vi "Beta.vi"() -> ()   [LabVIEW 2019]
uses:
  Classes/Settings/ObjectSettings/ObjectSettings.lvclass/ObjectSettings.ctl
  <vilib>/Utility/miscctls.llb/LVPositionTypeDef.ctl
  Classes/Parse/ParseVectorFile/ParseVectorFile.lvclass
  C:/Program Files (x86)/National Instruments/LabVIEW 2019/vi.lib/JKI/JKI SMO/SMO/SMO.lvclass
  Classes/Settings/Setting Database/Setting Database.lvclass
  Classes/Tool/Tool Data/Tool Data/Tool Data.lvclass
  Classes/Subpanel/Manager/Subpanel.Edit.lvclass
  C:/Users/Albro/Documents/GitHub/AFM-Lithography/lvsrc/Classes/Subpanel/Subpanel.lvclass
  Classes/Render/BigMAQ/BigMAQ.lvclass
  Classes/Selector/Selector.lvclass
  subVIs/AFM API/AFM_Driver_Manager/AFM_Driver_Manager.lvclass
  <userlib>/LevyLab/Configuration/Configuration.lvclass
  Classes/Settings/Setting Database/Typedefs/PublicEvents--Setting Database.RectanglesUpdated.ctl
  Classes/Settings/Rectangle Settings/Rectangle Settings.lvclass
  C:/Users/Albro/Documents/GitHub/AFM-Lithography/lvsrc/Classes/Settings/ObjectSettings/ObjectSettings.lvclass
  Classes/Settings/Setting Database/Typedefs/PublicEvents--Setting Database.PathsUpdated.ctl
  Classes/Settings/Path Settings/Path Settings.lvclass
  Classes/Settings/Setting Database/Typedefs/PublicEvents--Setting Database.FunnelsUpdated.ctl
  Classes/Settings/Funnel Settings/Funnel Settings.lvclass
  Classes/Settings/Setting Database/Typedefs/PublicEvents--Setting Database.DotsUpdated.ctl
  Classes/Settings/Dot Settings/Dot Settings.lvclass
  Classes/Parse/ParsePaths/Path.lvclass
  Classes/Parse/Rectangle/Rectangle.lvclass
  Classes/Parse/Image/SVGImage.lvclass
  Classes/Parse/Dot/Dot.lvclass
  <userlib>/LevyLab/Relay Box/Typedefs/Resistor--enum.ctl
  Classes/Render/Inset/Inset.lvclass
  Classes/Log/Log.Litho/Log.Litho.lvclass
  Classes/Settings/Setting Database/Typedefs/PrivateEvents--Setting Database.Add To Group.ctl
  Classes/Settings/Setting Database/Typedefs/PrivateEvents--Setting Database.Create New Group.ctl
  Classes/Settings/Setting Database/Typedefs/PrivateEvents--Setting Database.Refresh.ctl
  Classes/Tool/Tool Data/Tool Data/Typedefs/PrivateEvents--Tool Data.Update Objects.ctl
  Classes/Parse/Image/SVGImage.lvclass/SVGImage.ctl
  Controls/Configuration.ctl
  a998b7c0-e198-41fb-897a-9ce541eca358.vi
  <vilib>/Platform/browser.llb/Open URL in Default Browser (string).vi
  <vilib>/Utility/sysdir.llb/Get System Directory.vi
  Classes/Tool/Tool Path/Tool Path.lvclass
  Classes/Tool/Tool Funnel/Tool Funnel.lvclass
  Classes/Tool/Tool Rectangle/Tool Rectangle.lvclass
  Classes/Tool/Tool Dot/Tool Dots.lvclass
  <userlib>/LevyLab/Relay Box/Relay-Box.lvclass
  Classes/Subpanel/Subpanel.lvclass
  <vilib>/JKI/JKI SMO/SMO/SMO.lvclass
  Classes/Settings/ObjectSettings/ObjectSettings.lvclass
  Classes/Identity/Identifier.lvclass
panel:
  out "Zoom":string
  in  "Zoom Type":enum32{"Zoom In", "Zoom Out"}(radio)
  in  "Zoom to Fit":bool
  out "Render":T1(plugin-control)
  out "version":string
  out "Ready?":bool
  out "Estimated Time":string
  in  "Run":bool
  in  "Refresh Button":bool
  in  "Done":bool
  in  "Help":bool
  in  "Abort":bool
  in  "Settings":T2(tab)
  out "Status":string
  in  "Background Image":path caption="Path"
  in  "Inkscape File (.svg)":path caption="Path"
  in  "Hide Labels?":bool
  in  "MCLB":i32(listbox) caption="Multicolumn Listbox 2"
  in  "AFM Type":u16(ring) caption="Ring" items=["Asylum"]
  in  "Overwrite?":bool
  in  "Normal Save Path":path caption="Path"
  in  "Save Render":bool caption="Save"
  in  "Autosave?":bool
  in  "Autosave Path":path caption="Path"
  in  "Inset Editor":bool
  out "Image Filename":string
  in  "Image Data Range":cluster{sgl, sgl}(slide)={100.0, 0.0} scale=0.0..100.0
  in  "Page":u32 caption="Numeric" max=3
  # "AFM Lithography"
  # "Render"
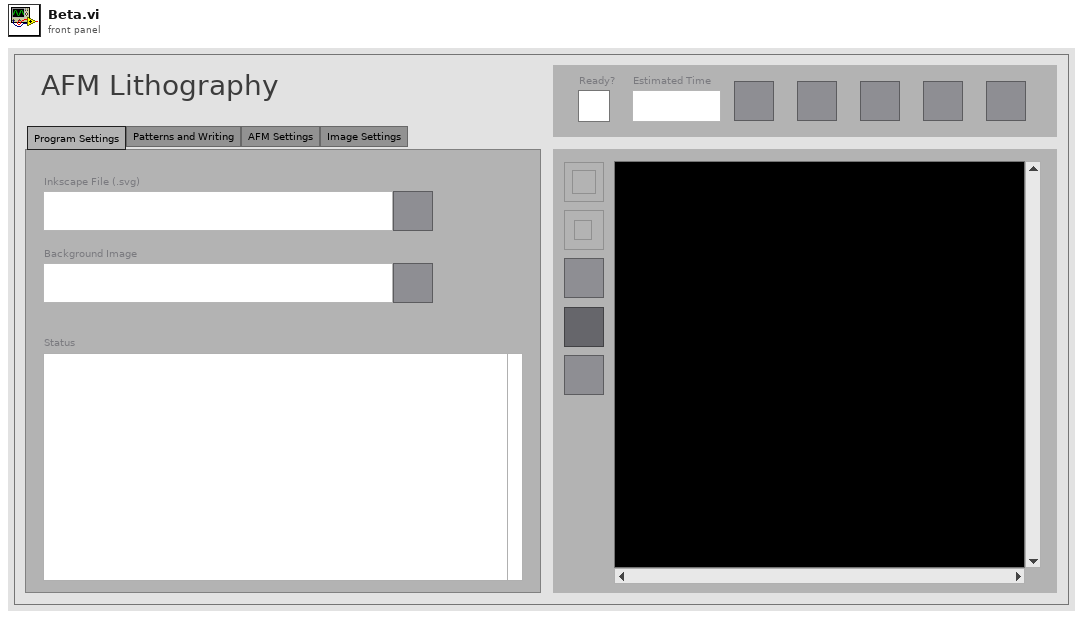
[diagram p1: front panel]
types:
  T1 = typedef "IMAQ Image.ctl" = refnum<image>
  T2 = enum32{"Program Settings", "Patterns and Writing", "AFM Settings", "Image Settings"}
  T3 = cluster{"Groups":string[], "Enable Items":bool[]}
  T4 = typedef "LVPositionTypeDef.ctl" = cluster{"Left":i32, "Top":i32}
  T5 = cluster{"Point":T4, "Button":u16, "PlatMods":cluster{"Shift":bool, "Ctrl":bool, "Alt":bool, "Cmd":bool, "Opt":bool}}
  T6 = enum32{"Invalid", "Standard", "Closed", "Hidden", "Minimized", "Maximized"}
  T7 = enum32{"invalid app kind", "Development System", "Run Time System", "Student Edition", "Embedded LabVIEW", "Evaluation", "Custom"}
  T8 = cluster{"Background.Range":cluster{sgl, sgl}, "Background.Page":i32}
  T9 = enum8{"Enabled", "Disabled", "Disabled and Grayed Out"}
  T10 = cluster{"Pattern":string, "Pattern Label":string, "Prompt":string}
  T11 = cluster{"paths":string[], "funnels":string[], "rects":string[], "dots":string[]}
  T12 = typedef "Setting Database.lvclass/PrivateEvents--Setting Database.Add To Group.ctl" = cluster{"Name":string, "Group":string}
  T13 = typedef "Setting Database.lvclass/PrivateEvents--Setting Database.Create New Group.ctl" = cluster{"Name":string, "Group":string}
  T14 = typedef "Setting Database.lvclass/PrivateEvents--Setting Database.Refresh.ctl" = cluster{"Paths":string[], "Rectangles":string[], "Funnels":string[], "Dots":string[]}
  T15 = cluster{"Paths":refnum<class "Path.lvclass">[], "Rectangles":refnum<class "Rectangle.lvclass">[], "SVGImage":refnum<class "SVGImage.lvclass">, "Dots":refnum<class "Dot.lvclass">[], "Funnels":refnum<class "Path.lvclass">[]}
  T16 = typedef "Tool Data.lvclass/PrivateEvents--Tool Data.Update Objects.ctl" = cluster{"Settings":cluster{"Paths":T17, "Rectangles":T18, "Funnels":T19, "Dots":T20}, "Data":cluster{"Paths":refnum<class "Path.lvclass">[], "Rectangles":refnum<class "Rectangle.lvclass">[], "SVGImage":refnum<class "SVGImage.lvclass">, "Dots":refnum<class "Dot.lvclass">[], "Funnels":refnum<class "Path.lvclass">[]}}
  T17 = typedef "Setting Database.lvclass/PublicEvents--Setting Database.PathsUpdated.ctl" = refnum<class "Path Settings.lvclass">[]
  T18 = typedef "Setting Database.lvclass/PublicEvents--Setting Database.RectanglesUpdated.ctl" = refnum<class "Rectangle Settings.lvclass">[]
  T19 = typedef "Setting Database.lvclass/PublicEvents--Setting Database.FunnelsUpdated.ctl" = refnum<class "Funnel Settings.lvclass">[]
  T20 = typedef "Setting Database.lvclass/PublicEvents--Setting Database.DotsUpdated.ctl" = refnum<class "Dot Settings.lvclass">[]
  T21 = typedef "Configuration.ctl" = cluster{"Inkscape Path":path, "Background Path":path, "Autosave Render Path":path, "Autosave Render":bool, "Hide Labels":bool, "Normal Render Path":path}
  T22 = typedef "Relay-Box.lvclass/Resistor--enum.ctl" = enum16{"open", "discharge tip", "0 ohms", "100k ohm", "10M ohm", "1G ohm"}
  T23 = cluster{"Core":cluster{"Current VI Reference":refnum<vi>, "Close Panel on Exit?":bool}, "tooler":refnum<class "Tool Data.lvclass">, "parser":refnum<class "ParseVectorFile.lvclass">, "settings":refnum<class "Setting Database.lvclass">, "selector":refnum<class "Selector.lvclass">, "sbpnl.edit":refnum<class "Subpanel.Edit.lvclass">, "big-maq":refnum<class "BigMAQ.lvclass">, "config":refnum<class "Configuration.lvclass">, "afm_mngr":refnum<class "AFM_Driver_Manager.lvclass">, "Obj Settings":cluster{"Rectangles":T18, "Paths":T17, "Funnels":T19, "Dots":T20}, "Changed Obj":cluster{"Path Changes":cluster{bool, "index of element":i32}[], "Funnel Changes":cluster{bool, "index of element":i32}[], "Rectangle Changes":cluster{bool, "index of element":i32}[], "Dot Changes":cluster{bool, "index of element":i32}[]}, "GUIDs":cluster{"Dots":string[], "Funnels":string[], "Rects":string[], "Paths":string[]}, "Parsed Obj":cluster{"Paths":refnum<class "Path.lvclass">[], "Rectangles":refnum<class "Rectangle.lvclass">[], "Background":refnum<class "SVGImage.lvclass">, "Dots":refnum<class "Dot.lvclass">[], "Funnels":refnum<class "Path.lvclass">[], "Other Images":refnum<class "SVGImage.lvclass">[]}, "Litho":cluster{"Name":string, "Litho":cluster{"X":dbl, "Y":dbl, "Speed":dbl, "Voltage":dbl}[], "Set Resistance":T22, "Meta":variant}[], "root path":path, "UI":cluster{"Hide Labels":bool, "Image Data Range":cluster{sgl, sgl}, "Status":string, "Autosave Path":path, "Autosave?":bool, "Inkscape File (.svg)":path, "Background Image":path, "Page":u32, "Normal Save Path":path}, "inset":refnum<class "Inset.lvclass">, "log":refnum<class "Log.Litho.lvclass">, "Offline Log":string, "Zoom History":cluster{"X":sgl, "Y":sgl}[]}
  T24 = typedef "LVPoint32TypeDef.ctl" = cluster{"Horizontal":i32, "Vertical":i32}
  T25 = cluster{"Paths":refnum<class "Tool Path.lvclass">[], "Funnels":refnum<class "Tool Funnel.lvclass">[], "Rectangles":refnum<class "Tool Rectangle.lvclass">[], "Dots":refnum<class "Tool Dots.lvclass">[]}
  T26 = cluster{"Shift":bool, "Ctrl":bool, "Alt":bool, "Cmd":bool, "Opt":bool}
  T27 = cluster{"Hide Labels":bool, "Image Data Range":cluster{sgl, sgl}, "Status":string, "Autosave Path":path, "Autosave?":bool, "Inkscape File (.svg)":path, "Background Image":path, "Page":u32, "Normal Save Path":path}
  T28 = cluster{"Name":string, "Litho":cluster{"X":dbl, "Y":dbl, "Speed":dbl, "Voltage":dbl}[], "Set Resistance":T22, "Meta":variant}[]
  T29 = cluster{"Paths":refnum<class "Path.lvclass">[], "Rectangles":refnum<class "Rectangle.lvclass">[], "Background":refnum<class "SVGImage.lvclass">, "Dots":refnum<class "Dot.lvclass">[], "Funnels":refnum<class "Path.lvclass">[], "Other Images":refnum<class "SVGImage.lvclass">[]}
  T30 = cluster{"Dots":string[], "Funnels":string[], "Rects":string[], "Paths":string[]}
  T31 = cluster{"Path Changes":cluster{bool, "index of element":i32}[], "Funnel Changes":cluster{bool, "index of element":i32}[], "Rectangle Changes":cluster{bool, "index of element":i32}[], "Dot Changes":cluster{bool, "index of element":i32}[]}
  T32 = cluster{"Rectangles":T18, "Paths":T17, "Funnels":T19, "Dots":T20}
  T33 = cluster{"Current VI Reference":refnum<vi>, "Close Panel on Exit?":bool}
  T34 = typedef "AFM_Driver_Manager.lvclass/AFM_Driver_Manager.PublicEvents.ctl" = cluster{"Lithography Done":refnum<user-event>}
  T35 = typedef "Setting Database.lvclass/PublicEvents--Cluster.ctl" = cluster{"NewActivePath":refnum<user-event>, "PathsUpdated":refnum<user-event>, "RectanglesUpdated":refnum<user-event>, "NewActiveRectangle":refnum<user-event>, "NewActiveFunnel":refnum<user-event>, "FunnelsUpdated":refnum<user-event>, "NewActiveDot":refnum<user-event>, "DotsUpdated":refnum<user-event>}
  T36 = typedef "ParseVectorFile.lvclass/PublicEvents--Cluster.ctl" = cluster{"ParsedData":refnum<user-event>}
  T37 = typedef "Tool Data.lvclass/PublicEvents--Cluster.ctl" = cluster{"Objects Updated":refnum<user-event>}
  T38 = typedef "SMO.lvclass/SMOState --Enum.ctl" = enum16{"unknown", "Created", "Started", "Stopped"}
  T39 = typedef "Selector.lvclass/Item.ctl" = cluster{"Name":string, "Group":string, "Enabled":bool}
  T40 = cluster{"X":dbl, "Y":dbl, "Speed":dbl, "Voltage":dbl}[]
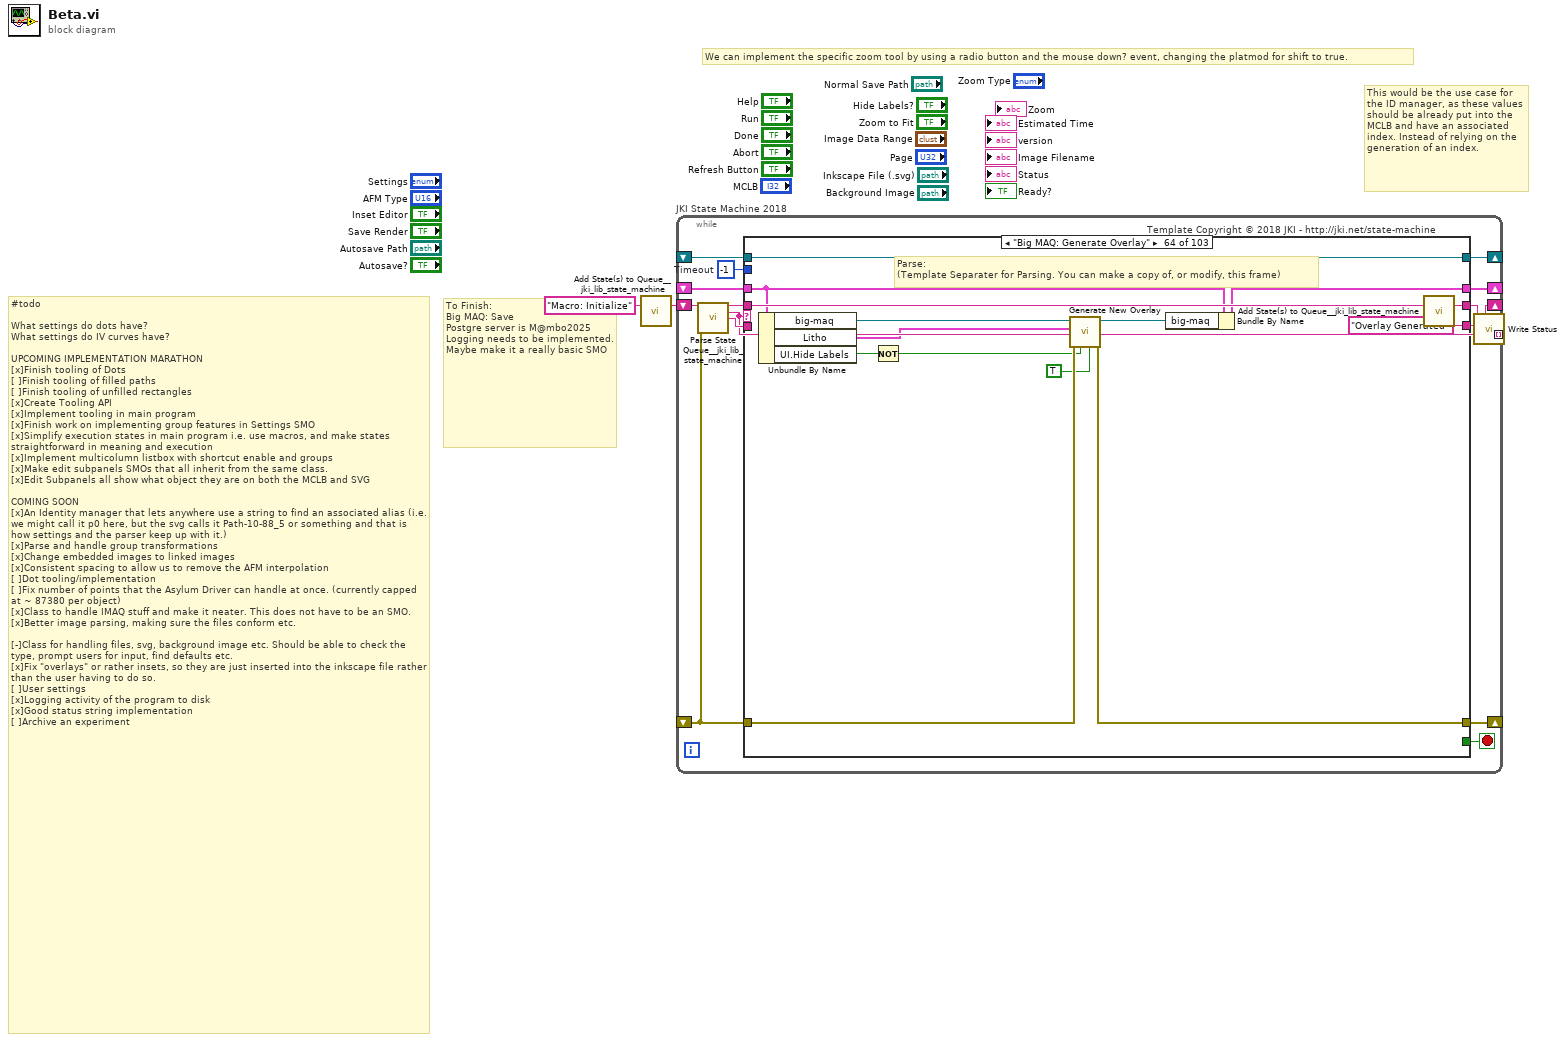
[diagram p0: block diagram]
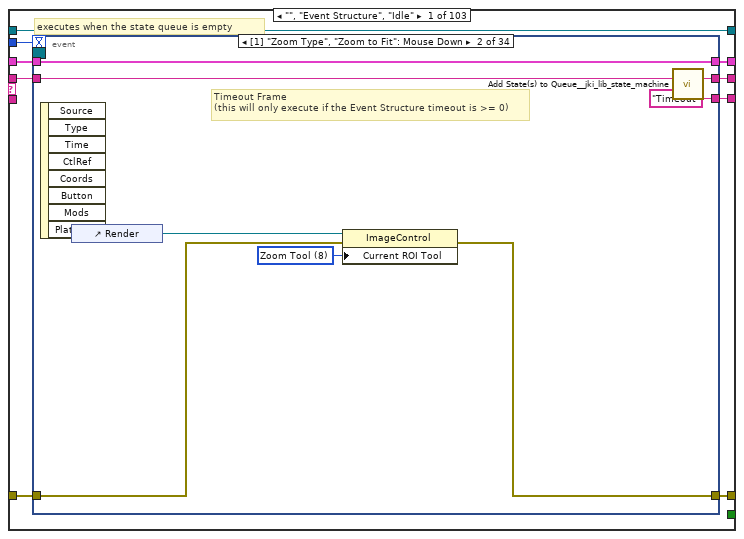
[diagram p2: hidden frame]
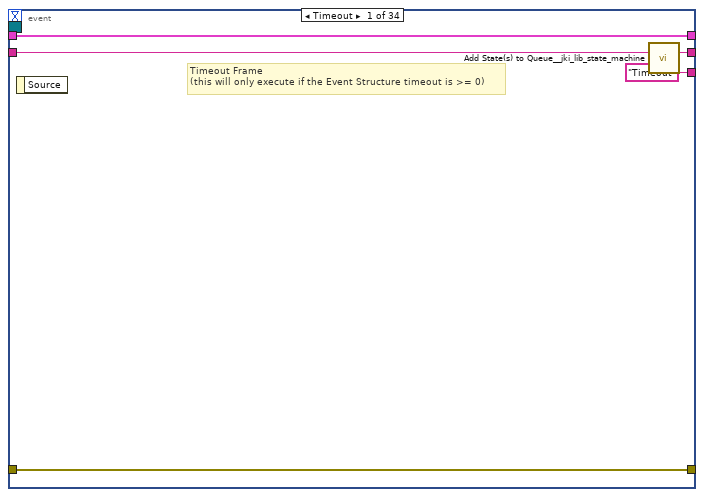
[diagram p3: hidden frame]
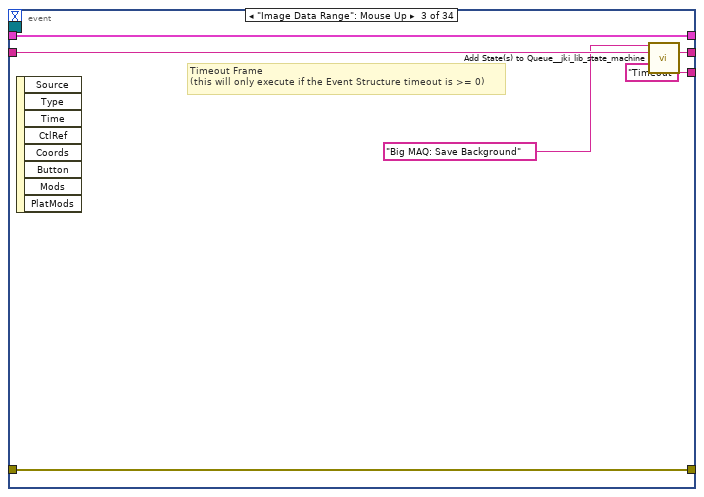
[diagram p4: hidden frame]
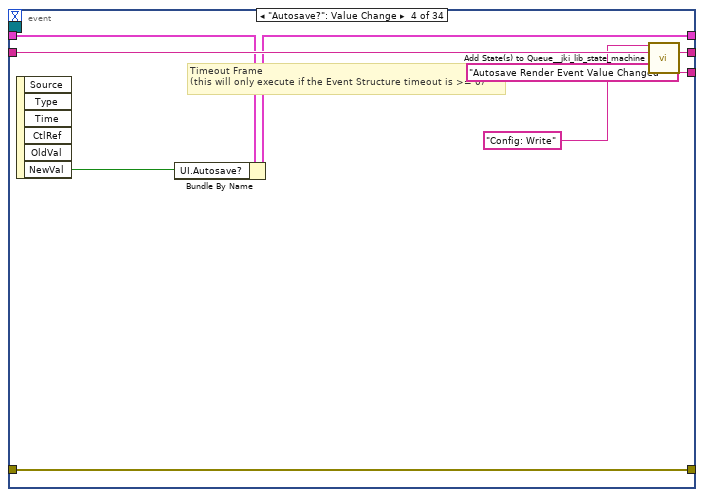
[diagram p5: hidden frame]
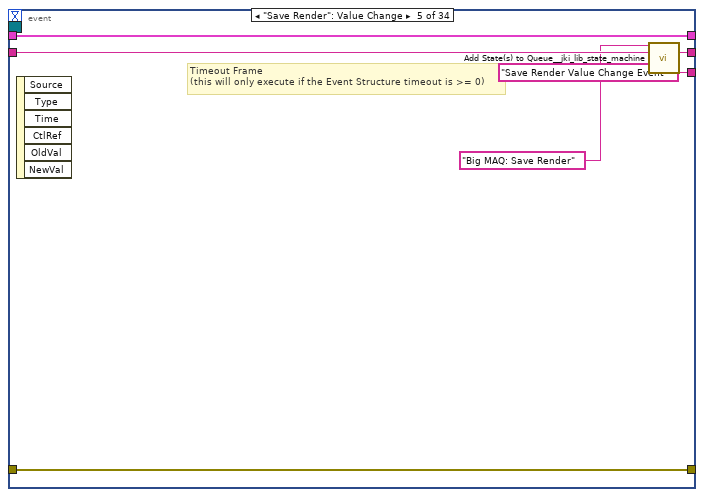
[diagram p6: hidden frame]
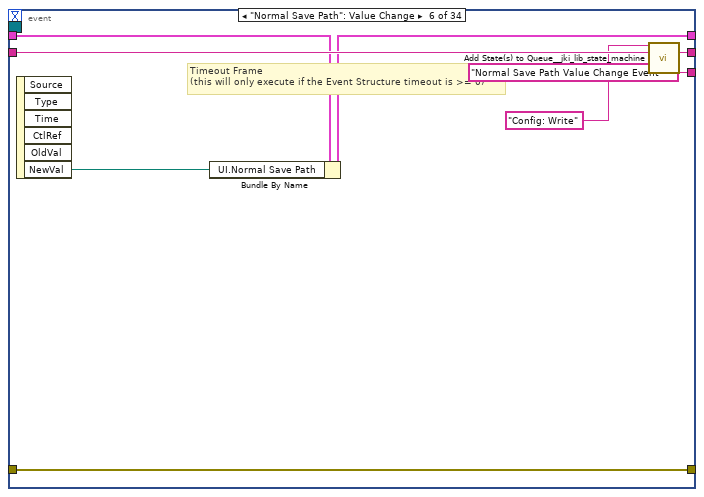
[diagram p7: hidden frame]
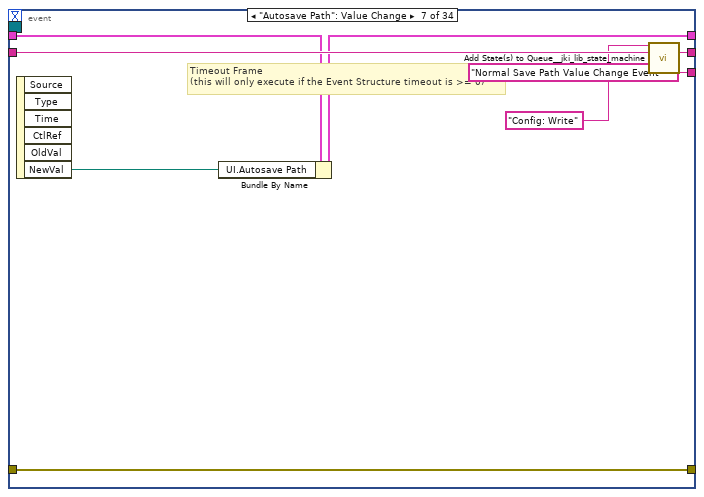
[diagram p8: hidden frame]
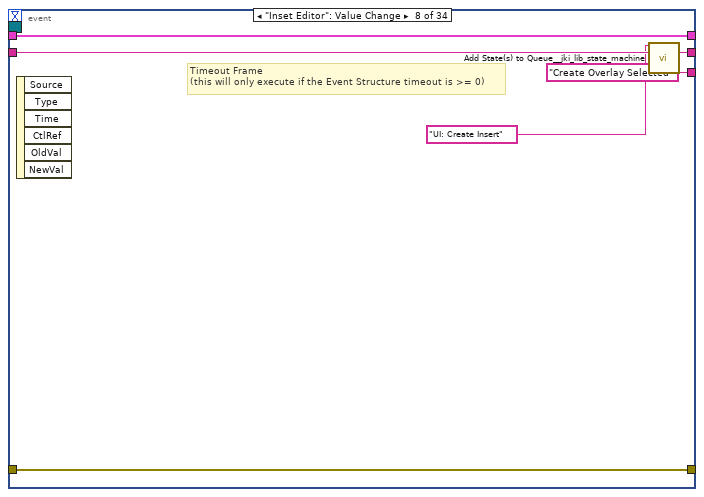
[diagram p9: hidden frame]
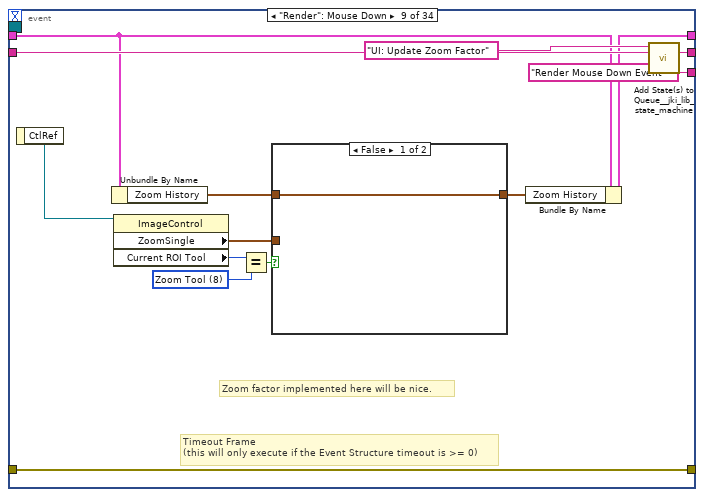
[diagram p10: hidden frame]
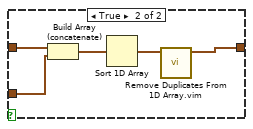
[diagram p11: hidden frame]
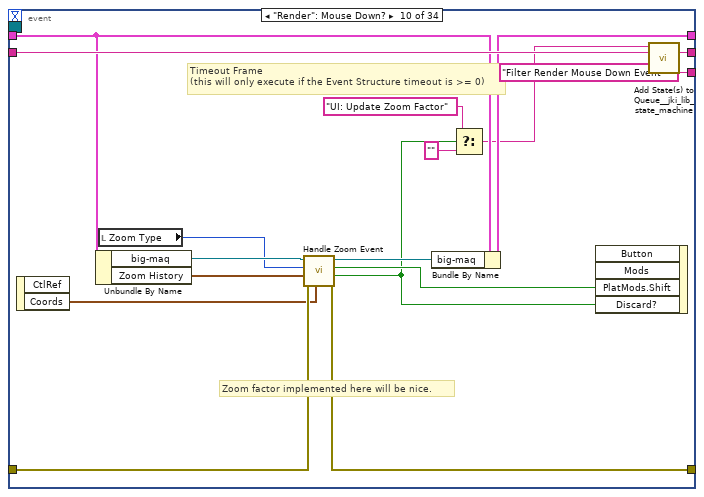
[diagram p12: hidden frame]
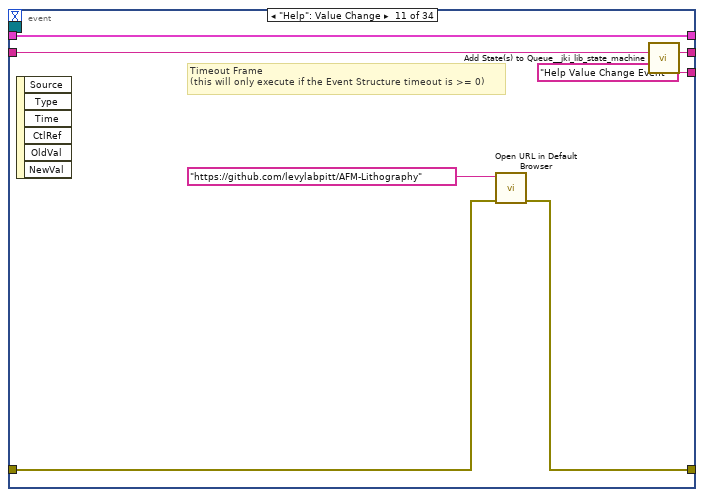
[diagram p13: hidden frame]
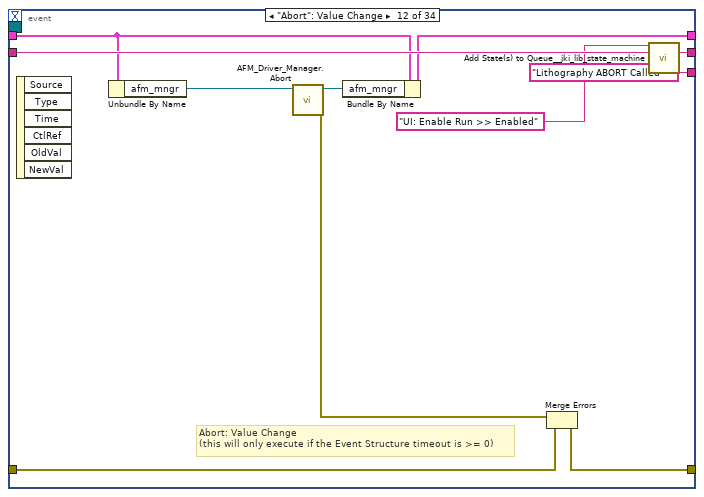
[diagram p14: hidden frame]
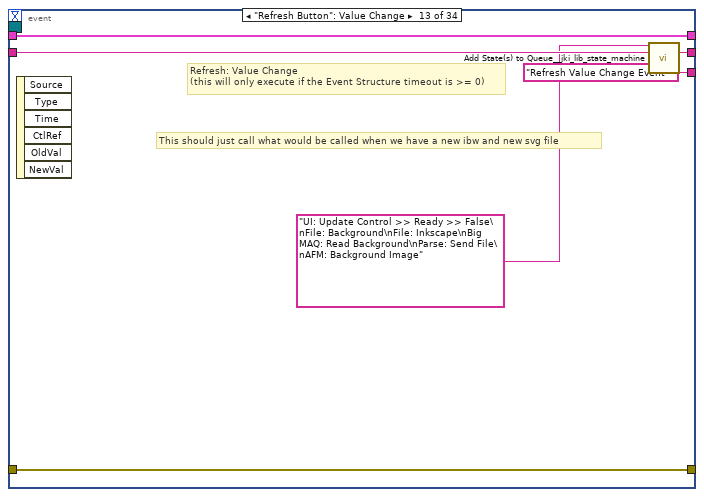
[diagram p15: hidden frame]
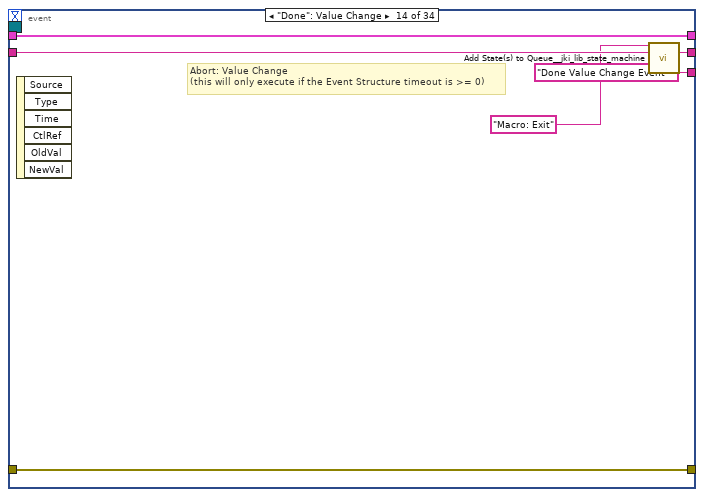
[diagram p16: hidden frame]
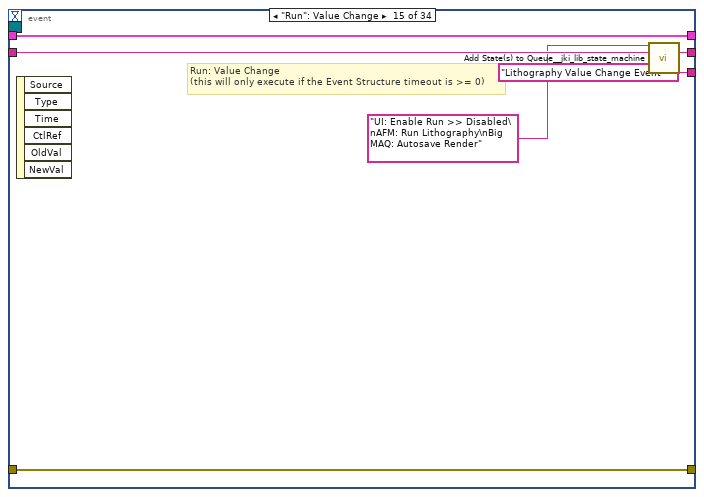
[diagram p17: hidden frame]
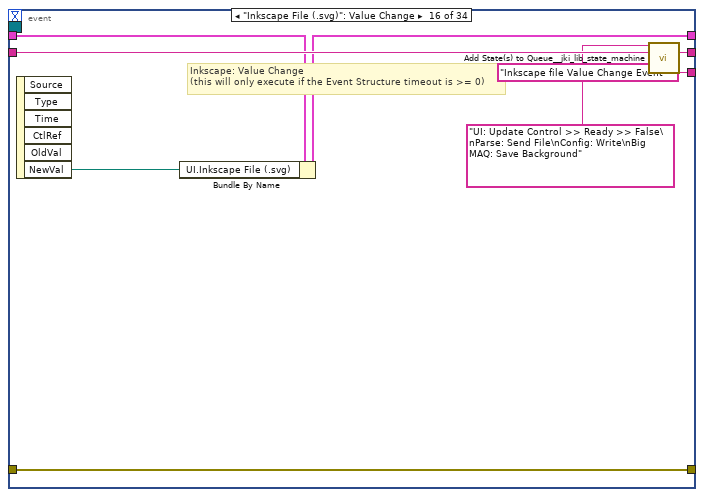
[diagram p18: hidden frame]
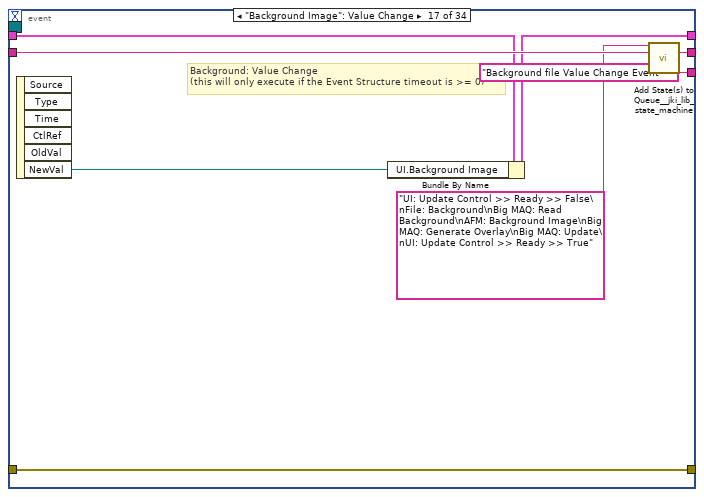
[diagram p19: hidden frame]
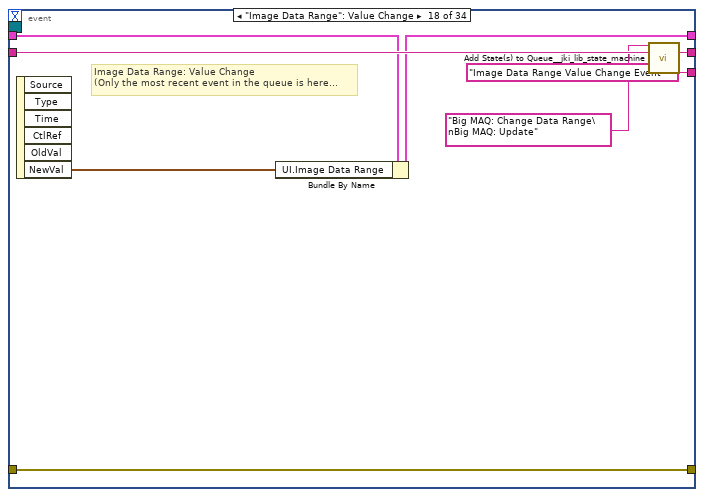
[diagram p20: hidden frame]
diagram:
  # "We can implement the specific zoom tool by using a radio button and the mouse down? event, changing the platmod for shift to true."
  # "#todo\n\nWhat settings do dots have?\nWhat settings do IV curves have?\n\nUPCOMING IMPLEMENTATION MARATHON\n[x]Finish tooling of Dots\n[ ]Finish tooling of filled paths\n[ ]Finish tooling of unfilled rectangles\n[x]Create Tooling API\n[x]Implement tooling in main program\n[x]Finish work on implementing group features in Settings SMO\n[x]Simplify execution states in main program i.e. use macros, and make states straightforward in meaning and execution\n[x]Implement multicolumn listbox with shortcut enable and groups\n[x]Make edit subpanels SMOs that all inherit from the same class.\n[x]Edit Subpanels all show what object they are on both the MCLB and SVG\n\nCOMING SOON\n[x]An Identity manager that lets anywhere use a string to find an associated alias (i.e. we might call it p0 here, but the svg calls it Path-10-88_5 or something and that is how settings and the parser keep up with it.)\n[x]Parse and handle group transformations\n[x]Change embedded images to linked images\n[x]Consistent spacing to allow us to remove the AFM interpolation\n[ ]Dot tooling/implementation\n[ ]Fix number of points that the Asylum Driver can handle at once. (currently capped at ~ 87380 per object)\n[x]Class to handle IMAQ stuff and make it neater. This does not have to be an SMO.\n[x]Better image parsing, making sure the files conform etc.\n\n[-]Class for handling files, svg, background image etc. Should be able to check the type, prompt users for input, find defaults etc.\n[x]Fix \"overlays\" or rather insets, so they are just inserted into the inkscape file rather than the user having to do so.\n[ ]User settings\n[x]Logging activity of the program to disk\n[x]Good status string implementation\n[ ]Archive an experiment"
  # "This would be the use case for the ID manager, as these values should be already put into the MCLB and have an associated index. Instead of relying on the generation of an index."
  # "To Finish:\nBig MAQ: Save\nPostgre server is M@mbo2025\nLogging needs to be implemented. Maybe make it a really basic SMO"
  n1 = call <vilib>:"Add State(s) to Queue__jki_lib_state_machine.vi"("State(s) in (\"\")"="Macro: Initialize") -> ("States Out"=w2:string)  [unwired: 14 in]
  n2 = while "JKI State Machine 2018" {
    shift-right: [w12] -> _
    shift-left: _ -> [w11]
    shift-right: [w14] -> _
    shift-left: _ -> [w9]
    shift-right: [w4] -> _
    shift-left: w2 -> [w15]
    shift-right: [w8] -> _
    shift-left: _ -> [w7]
    tunnel: [w3] -> _ mode=indexing
    stop <- w13 stop-if-true
    w10 = -1  # Timeout
    # "Template Copyright © 2018 JKI - http://jki.net/state-machine"
    n3 = call <vilib>:"Parse State Queue__jki_lib_state_machine.vi"("State Queue"=w15, "Error In (no error)"=w9) -> ("Remaining States"=w17:string, "Current State"=w3:string, "Arguments"=w16:string)  [unwired: 11 in]
    n4 = case shown="\"Big MAQ: Generate Overlay\"" w3 {
      selector: w3 -> [_ _ w443 _ _ _ _ _ _ _ _ _ _ _ _ _ _ _ _ _ _ _ _ _ _ _ _ _ _ _ _ _ _ _ _ _ _ _ _ _ _ _ _ _ _ _ _ _ _ _ _ _ _ _ _ _ _ _ _ _ _ _ _ _ _ _ _ _ _ _ _ _ _ _ _ _ _ _ _ _ _ _ _ _ _ _ _ _ _ _ _ _ _ _ _ _ _ _ _ _ _ _ _]
      tunnel: w17 -> [w26 w441 w447 w468 w475 w481 w486 w493 w523 w530 w535 w555 w562 w567 w597 w610 w620 w635 w661 w682 w690 w766 w779 w791 w861 w867 w873 w879 w885 w891 w902 w907 w916 w924 w929 w948 w979 w991 w998 w1013 w1020 w1031 w1043 w1055 w1062 w1075 w1113 w1131 w1170 w1182 w1197 w1204 w1222 w1245 w1259 w1282 w1295 w1307 w1314 w1335 w1358 w1370 w1380 w1394 w1410 w1425 w1438 w1450 w1462 w1476 w1494 w1506 w1513 w1530 w1558 w1568 w1578 w1595 w1605 w1621 w1647 w1683 w1690 w1702 w1712 w1724 w1731 w1744 w1757 w1764 w1776 w1794 w1814 w1821 w1831 w1841 w1852 w1878 w1894 w1905 w1917 w1931 w1941]
      tunnel: w16 -> [_ _ _ _ _ _ _ _ _ _ _ _ _ _ _ _ _ w624 w642 _ w685 _ w774 w785 _ _ _ _ _ _ _ _ _ _ _ _ _ _ _ _ _ _ _ _ _ w1064 w1106 w1123 _ _ _ _ _ _ _ _ _ _ _ _ w1351 _ _ _ _ _ _ _ _ _ _ _ _ w1514 _ _ _ w1587 _ _ w1639 _ _ w1693 _ _ _ _ _ _ _ _ _ _ _ _ _ _ _ _ w1908 _ _]
      tunnel: w11 -> [w24 w438 w445 w461 w472 w479 w483 w491 _ w525 w532 w551 w560 w564 w592 w599 w614 w633 w648 w677 w693 w759 w777 w787 w858 w864 w870 w876 w882 w888 w899 w904 w911 w917 w926 w933 w970 w988 w996 w1007 w1016 w1028 w1040 w1052 w1058 w1072 w1110 w1128 w1167 w1179 w1194 w1200 w1219 w1236 w1256 w1279 w1292 w1304 w1310 w1332 w1355 w1367 w1377 w1391 w1407 w1422 w1435 w1447 w1459 w1473 w1491 w1503 w1509 w1515 w1555 w1565 w1575 w1592 w1602 w1618 w1644 w1680 w1686 w1699 w1709 w1721 w1727 w1741 w1754 w1760 w1773 w1788 w1811 w1817 w1828 w1838 w1849 w1875 w1891 w1902 w1914 w1928 w1938]
      tunnel: [w23 w439 w449 w465 errorcluster {"status"=FALSE, "code"=0, "source"=""} ("error out") w478 w484 w488 w520 w526 w533 w547 w557 w565 w571 w608 w616 w623 w638 w675 w689 w746 w775 w788 w859 w865 w871 w877 w883 w889 w900 w905 w914 w922 w927 w939 w962 w989 w994 w1010 w1018 w1023 w1034 w1046 w1060 w1066 w1105 w1116 w1156 w1172 w1188 w1202 w1207 w1241 w1252 w1266 w1287 w1298 w1312 w1320 w1348 w1364 w1374 w1388 w1399 w1419 w1431 w1443 w1456 w1470 w1488 w1500 w1511 w1521 w1550 w1561 w1571 w1586 w1598 w1613 w1641 w1678 w1688 w1696 w1706 w1716 w1729 w1735 w1749 w1762 w1767 w1787 w1805 w1819 w1824 w1835 w1845 w1871 w1887 w1898 w1910 w1921 w1934] -> w14
      tunnel: w9 -> [w22 w439 w448 w465 w471 w478 w484 w489 w520 w527 w533 w540 w558 w565 w575 w608 w615 w622 w646 w674 w687 w760 w776 w789 w859 w865 w871 w877 w883 w889 w900 w905 w914 w922 w927 w938 w969 w989 w993 w1009 w1018 w1022 w1033 w1045 w1060 w1065 w1104 w1115 w1157 w1173 w1185 w1202 w1206 w1237 w1251 w1265 w1286 w1297 w1312 w1324 w1347 w1363 w1373 w1387 w1398 w1418 w1430 w1439 w1455 w1469 w1487 w1499 w1511 w1520 w1549 w1560 w1570 w1585 w1599 w1612 w1640 w1677 w1688 w1695 w1705 w1717 w1729 w1734 w1748 w1762 w1766 w1786 w1804 w1819 w1823 w1834 w1844 w1870 w1886 w1897 w1909 w1920 w1933]
      tunnel: [w25 w440 w446 w467 w474 w480 w485 w492 w522 w529 w534 w554 w561 w566 w596 w609 w619 w634 w660 w681 w694 w765 w778 w790 w860 w866 w872 w878 w884 w890 w901 w906 w915 w923 w928 w947 w978 w990 w997 w1012 w1019 w1030 w1042 w1054 w1061 w1074 w1112 w1130 w1169 w1181 w1196 w1203 w1221 w1244 w1258 w1281 w1294 w1306 w1313 w1334 w1357 w1369 w1379 w1393 w1409 w1424 w1437 w1449 w1461 w1475 w1493 w1505 w1512 w1529 w1557 w1567 w1577 w1594 w1604 w1620 w1646 w1682 w1689 w1701 w1711 w1723 w1730 w1743 w1756 w1763 w1775 w1793 w1813 w1820 w1830 w1840 w1851 w1877 w1893 w1904 w1916 w1930 w1940] -> w6
      tunnel: [_ _ _ _ _ TRUE _ _ _ _ _ _ _ _ _ _ _ _ _ _ _ _ _ _ _ _ _ _ _ _ _ _ _ _ _ _ _ _ _ _ _ _ _ _ _ _ _ _ _ _ _ _ _ _ _ _ _ _ _ _ _ _ _ _ _ _ _ _ _ _ _ _ _ _ _ _ _ _ _ _ _ _ _ _ _ _ _ _ _ _ _ _ _ _ _ _ _ _ _ _ _ _ _] -> w13
      tunnel: [w21 w438 w445 w466 w472 w479 w483 w491 w521 w525 w532 w551 w560 w564 w593 w599 w617 w633 w651 w678 w692 w759 w777 w787 w858 w864 w870 w876 w882 w888 w899 w904 w912 w918 w926 w934 w971 w988 w996 w1007 w1017 w1029 w1041 w1053 w1059 w1073 w1111 w1129 w1168 w1180 w1195 w1201 w1220 w1243 w1257 w1280 w1293 w1305 w1311 w1333 w1356 w1368 w1378 w1392 w1408 w1423 w1436 w1448 w1460 w1474 w1492 w1504 w1510 w1528 w1556 w1566 w1576 w1593 w1603 w1619 w1645 w1681 w1687 w1700 w1710 w1722 w1728 w1742 w1755 w1761 w1774 w1792 w1812 w1818 w1829 w1839 w1850 w1876 w1892 w1903 w1915 w1929 w1939] -> w12
      tunnel: w10 -> [w20 _ _ _ _ _ _ _ _ _ _ _ _ _ _ _ _ _ _ _ _ _ _ _ _ _ _ _ _ _ _ _ _ _ _ _ _ _ _ _ _ _ _ _ _ _ _ _ _ _ _ _ _ _ _ _ _ _ _ _ _ _ _ _ _ _ _ _ _ _ _ _ _ _ _ _ _ _ _ _ _ _ _ _ _ _ _ _ _ _ _ _ _ _ _ _ _ _ _ _ _ _ _]
      tunnel: [w19 w437 w442 w455 w469 w476 w482 w490 w505 w524 w531 w553 w559 w563 w595 w607 w618 w632 w659 w680 w688 w764 w773 w784 w857 w863 w869 w875 w881 w886 w892 w903 w913 w921 w925 w946 w977 w987 w995 w1011 w1014 w1027 w1039 w1051 w1056 w1071 w1109 w1127 w1166 w1178 w1193 w1198 w1218 w1242 w1255 w1278 w1291 w1303 w1308 w1331 w1354 w1362 w1372 w1384 w1396 w1412 w1429 w1446 w1454 w1468 w1486 w1498 w1507 w1527 w1554 w1564 w1574 w1584 w1597 w1607 w1638 w1675 w1684 w1692 w1704 w1714 w1725 w1740 w1753 w1758 w1772 w1791 w1810 w1815 w1827 w1837 w1848 w1874 w1890 w1901 w1913 w1927 w1937] -> w8
      tunnel: w7 -> [w19 w437 w442 w455 w469 w476 w482 w490 w505 w524 w531 _ w559 w563 w595 w607 w618 w632 w659 w680 w688 w764 w773 w784 w857 w863 w869 w875 w881 w886 w892 w903 w913 w921 w925 w946 w977 w987 w995 w1011 w1014 w1027 w1039 w1051 w1056 w1071 w1109 w1127 w1166 w1178 w1193 w1198 w1218 w1242 w1255 w1278 w1291 w1303 w1308 w1331 w1354 w1362 w1372 w1384 w1396 w1412 w1429 w1446 w1454 w1468 w1486 w1498 w1507 w1527 w1554 w1564 w1574 w1584 w1597 w1607 w1638 w1675 w1684 w1692 w1704 w1714 w1725 w1740 w1753 w1758 w1772 w1791 w1810 w1815 w1827 w1837 w1848 w1874 w1890 w1901 w1913 w1927 w1937]
      tunnel: [w18 _ _ "" _ _ _ "Status Log Setup" "" _ _ "Events registered" "Events Unregistered" _ "Create Overlay (Currently Disabled)" "Update Zoom Factor Display" "Select Initialization" "Run Enable/Disabled" "" "Big-MAQ Control UI Initialized" w683 "UI Initialization" _ _ _ _ _ _ _ _ _ _ _ _ _ _ _ _ "Identity registry disposed" "Identity Registry Populated" _ "Inkscape File Sent to Parser" "Parser Stopped" "Parser Started" _ "New Active Object -- Settings Database" "Object Enabled State Changed" "Object Group Association Changed -- Sent to Settings Database" "Refresh Settings Database" "Settings Database Stopped" "Settings Database Started" _ "Tooler: Paths Sorted" "Tooler: Object IDs Determined" "Tooler generated Lithography Data" "Data Sent to Tooler" "Tooler Stopped" "Tooler started" _ w1315 "Big MAQ show-hide labels executed" "Big MAQ Zoom to Fit Executed" "Big-MAQ control updated" "Overlay Generated" "New Image Page Selected" "Image Data Range Updated" "Big MAQ Read Background" "Background for inkscape file save." ("t") "Render Saved to Disk" w1463 "Big-MAQ Closed Down" "Big-MAQ IMAQ manager Initialized" _ "Selector value changed by name." ("t") "New population of values inserted into selector." ("t") "Selector Updated" "Checkmarks applied" "Selector Model Value Changed" "Selector Model Order Updated" "Lithography Data Ordered" "Object Group Association Changed" "Selector Created" _ "New Property Subpanel Inserted" "Subpanel Closed" "Properties Subpanel Initialized" _ "Logger started" "Logger Stopped" _ "Configuration Initialized" "Configuration Written" "Configuration Read" _ "Lithography process finished." "AFM Manager Stopped" "Background Image Sent to Driver" "Lithography Data Sent to Driver" "Run Lithography Message Sent" "AFM Driver Inserted Into Subpanel" "Active AFM Driver Set" "AFM Driver Launched and Initialized" "AFM Driver Manager Initialized"] -> w5
      frame "", "Event Structure", "Idle" {
        # "executes when the state queue is empty"
        n5 = event shown="[1] \"Zoom Type\", \"Zoom to Fit\": Mouse Down" {
          selector: w19 -> [_ _ _ _ _ _ _ _ _ _ _ _ _ _ _ _ _ _ _ _ _ _ _ _ _ _ _ _ _ _ _ _ _ _]
          dyn-events: _ -> [_ _ _ _ _ _ _ _ _ _ _ _ _ _ _ _ _ _ _ _ _ _ _ _ _ _ _ _ _ _ _ _ _ _]
          timeout: w20 -> [_ _ _ _ _ _ _ _ _ _ _ _ _ _ _ _ _ _ _ _ _ _ _ _ _ _ _ _ _ _ _ _ _ _]
          tunnel: w26 -> [w31 w39 w45 w53 w59 w67 w75 w81 w95 w118 w125 w136 w142 w148 w154 w162 w170 w178 w186 w192 w205 w211 w229 w260 w291 w322 w351 w363 w378 w397 w406 w417 w430 w436]
          tunnel: [w30 w38 w44 w52 w58 w66 w74 w80 w94 w117 w124 w135 w141 w147 w153 w161 w169 w177 w185 w191 w204 w210 w228 w259 w290 w321 w350 w362 w377 w396 w405 w416 w429 w435] -> w25
          tunnel: w24 -> [w28 w37 w42 w48 w56 w62 w70 w78 w82 w107 w123 w127 w139 w145 w150 w157 w165 w173 w180 w189 w193 w208 w223 w257 w288 w319 w347 w359 w375 w394 w403 w414 w427 w433]
          tunnel: [w29 w34 w43 w51 w57 w65 w73 w79 w93 w112 w120 w132 w140 w146 w152 w160 w168 w176 w184 w190 w203 w209 w214 w252 w283 w314 w349 w361 w366 w386 w399 w410 w424 w434] -> w23
          tunnel: w22 -> [w29 w33 w43 w51 w57 w65 w73 w79 w93 w111 w119 w131 w140 w146 w152 w160 w168 w176 w184 w190 w203 w209 w226 w245 w276 w306 w349 w361 w372 w385 w398 w409 w423 w434]
          tunnel: [w28 w37 w42 w49 w56 w63 w71 w78 w83 w108 w123 w128 w139 w145 w150 w158 w166 w174 w181 w189 w194 w208 w224 w258 w289 w320 w348 w360 w376 w395 w404 w415 w428 w433] -> w21
          tunnel: ["Timeout" "Timeout" "Timeout" "Autosave Render Event Value Changed" "Save Render Value Change Event" "Normal Save Path Value Change Event" "Normal Save Path Value Change Event" "Create Overlay Selected" "Render Mouse Down Event" "Filter Render Mouse Down Event" "Help Value Change Event" "Lithography ABORT Called" "Refresh Value Change Event" "Done Value Change Event" "Lithography Value Change Event" "Inkscape file Value Change Event" "Background file Value Change Event" "Image Data Range Value Change Event" "Page Value Change Event" "Zoom to Fit Event" "Show-Hide Labels Event" "AFM Lithography Finished Event" "Paths Updated" "Rectangles Updated" "Funnels Updated" "Dots Updated" "Tooled Objects Recieved from Tooler" "Parsed Data Recieved" "Multicolumn Listbox Value Change Event" _ _ _ "Multicolumn Listbox RCM Selection Event" _] -> w18
          event Timeout {
            # "Timeout Frame\n(this will only execute if the Event Structure timeout is >= 0)"
            n6 = event-data() -> ()  [unwired: 1 in, 1 out]
            n7 = call <vilib>:"Add State(s) to Queue__jki_lib_state_machine.vi"("State(s) in (\"\")"=w31) -> ("States Out"=w30:string)  [unwired: 14 in]
          }
          event "Zoom Type", "Zoom to Fit": Mouse Down {
            w32 = u32 8 items=["Zoom Tool"=8, "Selection Tool"=0, "Pan Tool"=9, "Point Tool"=1, "Line Tool"=2, "Rectangle Tool"=3, "Rotated Rectangle Tool"=12, "Polyline Tool"=10, "Polygon Tool"=5, "Freehand Tool"=11, "Closed Freehand Tool"=6, "Ellipse Tool"=4, "Annulus Tool"=7] ("Current ROI Tool")
            # "Timeout Frame\n(this will only execute if the Event Structure timeout is >= 0)"
            n8 = event-data() -> ()  [unwired: 1 in, 8 out]
            n9 = control-ref of="Render"() -> (w35:refnum<vi>)
            n10 = property class="ImageControl"(reference=w35, error in=w33, "Current ROI Tool"=w32) -> (error out=w34:errorcluster)  [unwired: 1 out]
            n11 = call <vilib>:"Add State(s) to Queue__jki_lib_state_machine.vi"("State(s) in (\"\")"=w39) -> ("States Out"=w38:string)  [unwired: 14 in]
          }
          event "Image Data Range": Mouse Up {
            # "Timeout Frame\n(this will only execute if the Event Structure timeout is >= 0)"
            n12 = event-data() -> ()  [unwired: 1 in, 8 out]
            n13 = call <vilib>:"Add State(s) to Queue__jki_lib_state_machine.vi"("State(s) in Front (\"\")"="Big MAQ: Save Background" ("State(s) in Front (\"\")"), "State(s) in (\"\")"=w45) -> ("States Out"=w44:string)  [unwired: 13 in]
          }
          event "Autosave?": Value Change {
            # "Timeout Frame\n(this will only execute if the Event Structure timeout is >= 0)"
            n14 = event-data() -> ("NewVal"=w47:bool)  [unwired: 1 in, 5 out]
            n15 = Bundle By Name(cluster=w48, "UI.Autosave?"=w47) -> (w49:T23)
            n16 = call <vilib>:"Add State(s) to Queue__jki_lib_state_machine.vi"("State(s) in Front (\"\")"="Config: Write", "State(s) in (\"\")"=w53) -> ("States Out"=w52:string)  [unwired: 13 in]
          }
          event "Save Render": Value Change {
            # "Timeout Frame\n(this will only execute if the Event Structure timeout is >= 0)"
            n17 = event-data() -> ()  [unwired: 1 in, 6 out]
            n18 = call <vilib>:"Add State(s) to Queue__jki_lib_state_machine.vi"("State(s) in Front (\"\")"="Big MAQ: Save Render", "State(s) in (\"\")"=w59) -> ("States Out"=w58:string)  [unwired: 13 in]
          }
          event "Normal Save Path": Value Change {
            # "Timeout Frame\n(this will only execute if the Event Structure timeout is >= 0)"
            n19 = event-data() -> ("NewVal"=w61:path)  [unwired: 1 in, 5 out]
            n20 = Bundle By Name(cluster=w62, "UI.Normal Save Path"=w61) -> (w63:T23)
            n21 = call <vilib>:"Add State(s) to Queue__jki_lib_state_machine.vi"("State(s) in Front (\"\")"="Config: Write", "State(s) in (\"\")"=w67) -> ("States Out"=w66:string)  [unwired: 13 in]
          }
          event "Autosave Path": Value Change {
            # "Timeout Frame\n(this will only execute if the Event Structure timeout is >= 0)"
            n22 = event-data() -> ("NewVal"=w69:path)  [unwired: 1 in, 5 out]
            n23 = Bundle By Name(cluster=w70, "UI.Autosave Path"=w69) -> (w71:T23)
            n24 = call <vilib>:"Add State(s) to Queue__jki_lib_state_machine.vi"("State(s) in Front (\"\")"="Config: Write", "State(s) in (\"\")"=w75) -> ("States Out"=w74:string)  [unwired: 13 in]
          }
          event "Inset Editor": Value Change {
            # "Timeout Frame\n(this will only execute if the Event Structure timeout is >= 0)"
            n25 = event-data() -> ()  [unwired: 1 in, 6 out]
            n26 = call <vilib>:"Add State(s) to Queue__jki_lib_state_machine.vi"("State(s) in Front (\"\")"="UI: Create Insert", "State(s) in (\"\")"=w81) -> ("States Out"=w80:string)  [unwired: 13 in]
          }
          event "Render": Mouse Down {
            w86 = u32 8 items=["Zoom Tool"=8, "Selection Tool"=0, "Pan Tool"=9, "Point Tool"=1, "Line Tool"=2, "Rectangle Tool"=3, "Rotated Rectangle Tool"=12, "Polyline Tool"=10, "Polygon Tool"=5, "Freehand Tool"=11, "Closed Freehand Tool"=6, "Ellipse Tool"=4, "Annulus Tool"=7] ("Current ROI Tool")
            # "Zoom factor implemented here will be nice."
            # "Timeout Frame\n(this will only execute if the Event Structure timeout is >= 0)"
            n27 = event-data() -> ("CtlRef"=w90:refnum<vi>)  [unwired: 1 in]
            n28 = Unbundle By Name(w82) -> ("Zoom History"=w89:cluster{"X":sgl, "Y":sgl}[])
            n29 = property class="ImageControl"(reference=w90) -> ("ZoomSingle"=w88:cluster{"X":sgl, "Y":sgl}, "Current ROI Tool"=w87:u32)  [unwired: 1 in, 2 out]
            n30 = Equal?(x=w87, y=w86) -> (x = y?=w85:bool)
            n31 = case shown="False" w85 {
              tunnel: w89 -> [w96 w101]
              tunnel: w88 -> [_ w100]
              tunnel: [w96 w97] -> w84
              frame False {
              }
              frame True {
                n32 = Build Array (concatenate)(w101, w100) -> (w99:cluster{"X":sgl, "Y":sgl}[])
                n33 = Sort 1D Array(array=w99) -> (sorted array=w98:cluster{"X":sgl, "Y":sgl}[])
                n34 = call "Remove Duplicates From 1D Array.vim"("array"=w98) -> ("array with duplicates removed"=w97:cluster{"X":sgl, "Y":sgl}[])  [unwired: 10 in]
              }
            }
            n35 = Bundle By Name(cluster=w82, "Zoom History"=w84) -> (w83:T23)
            n36 = call <vilib>:"Add State(s) to Queue__jki_lib_state_machine.vi"("State(s) in Front (\"\")"="UI: Update Zoom Factor", "State(s) in (\"\")"=w95) -> ("States Out"=w94:string)  [unwired: 13 in]
          }
          event "Render": Mouse Down? {
            # "Zoom factor implemented here will be nice."
            # "Timeout Frame\n(this will only execute if the Event Structure timeout is >= 0)"
            n37 = event-data() -> ("Coords"=w106:T24)  [unwired: 1 in, 1 out]
            n38 = Unbundle By Name(w107) -> ("big-maq"=w114:refnum<class "BigMAQ.lvclass">, "Zoom History"=w115:cluster{"X":sgl, "Y":sgl}[])
            n39 = local read "Zoom Type"() -> (w113:enum32{"Zoom In", "Zoom Out"})
            n40 = call "Handle Zoom Event.vi"("Point32"=w106, "error in"=w111, "Zoom History"=w115, "Zoom Type"=w113, "BigMAQ in"=w114) -> ("error out"=w112:errorcluster, "Discard?"=w104:bool, "Zoom Out?"=w110:bool, "BigMAQ out"=w109:refnum<class "BigMAQ.lvclass">)  [unwired: 3 in]
            n41 = Bundle By Name(cluster=w107, "big-maq"=w109) -> (w108:T23)
            n42 = Select(t="UI: Update Zoom Factor", s=w104, f="") -> (s? t:f=w102:string)
            n43 = event-data("PlatMods.Shift"=w110, "Discard?"=w104) -> ()  [unwired: 3 in, 1 out]
            n44 = call <vilib>:"Add State(s) to Queue__jki_lib_state_machine.vi"("State(s) in Front (\"\")"=w102, "State(s) in (\"\")"=w118) -> ("States Out"=w117:string)  [unwired: 13 in]
          }
          event "Help": Value Change {
            # "Timeout Frame\n(this will only execute if the Event Structure timeout is >= 0)"
            n45 = event-data() -> ()  [unwired: 1 in, 6 out]
            n46 = call-poly <vilib>:"Open URL in Default Browser.vi"("error in (no error)"=w119, "URL"="https://github.com/levylabpitt/AFM-Lithography") -> ("error out"=w120:errorcluster)  [unwired: 4 in, 1 out]
            n47 = call <vilib>:"Add State(s) to Queue__jki_lib_state_machine.vi"("State(s) in (\"\")"=w125) -> ("States Out"=w124:string)  [unwired: 14 in]
          }
          event "Abort": Value Change {
            # "Abort: Value Change\n(this will only execute if the Event Structure timeout is >= 0)"
            n48 = event-data() -> ()  [unwired: 1 in, 6 out]
            n49 = Unbundle By Name(w127) -> ("afm_mngr"=w133:refnum<class "AFM_Driver_Manager.lvclass">)
            n50 = call "AFM_Driver_Manager.Abort.vi"("AFM_Driver_Manager in"=w133) -> ("error out"=w130:errorcluster, "AFM_Driver_Manager out"=w129:refnum<class "AFM_Driver_Manager.lvclass">)  [unwired: 9 in]
            n51 = Bundle By Name(cluster=w127, "afm_mngr"=w129) -> (w128:T23)
            n52 = Merge Errors(w130, w131) -> (w132:errorcluster)
            n53 = call <vilib>:"Add State(s) to Queue__jki_lib_state_machine.vi"("State(s) in Front (\"\")"="UI: Enable Run >> Enabled" ("State(s) in Front (\"\")"), "State(s) in (\"\")"=w136) -> ("States Out"=w135:string)  [unwired: 13 in]
          }
          event "Refresh Button": Value Change {
            # "This should just call what would be called when we have a new ibw and new svg file"
            # "Refresh: Value Change\n(this will only execute if the Event Structure timeout is >= 0)"
            n54 = event-data() -> ()  [unwired: 1 in, 6 out]
            n55 = call <vilib>:"Add State(s) to Queue__jki_lib_state_machine.vi"("State(s) in Front (\"\")"="UI: Update Control >> Ready >> False\nFile: Background\nFile: Inkscape\nBig MAQ: Read Background\nParse: Send File\nAFM: Background Image", "State(s) in (\"\")"=w142) -> ("States Out"=w141:string)  [unwired: 13 in]
          }
          event "Done": Value Change {
            # "Abort: Value Change\n(this will only execute if the Event Structure timeout is >= 0)"
            n56 = event-data() -> ()  [unwired: 1 in, 6 out]
            n57 = call <vilib>:"Add State(s) to Queue__jki_lib_state_machine.vi"("State(s) in Front (\"\")"="Macro: Exit" ("State(s) in Front (\"\")"), "State(s) in (\"\")"=w148) -> ("States Out"=w147:string)  [unwired: 13 in]
          }
          event "Run": Value Change {
            # "Run: Value Change\n(this will only execute if the Event Structure timeout is >= 0)"
            n58 = event-data() -> ()  [unwired: 1 in, 6 out]
            n59 = call <vilib>:"Add State(s) to Queue__jki_lib_state_machine.vi"("State(s) in Front (\"\")"="UI: Enable Run >> Disabled\nAFM: Run Lithography\nBig MAQ: Autosave Render", "State(s) in (\"\")"=w154) -> ("States Out"=w153:string)  [unwired: 13 in]
          }
          event "Inkscape File (.svg)": Value Change {
            # "Inkscape: Value Change\n(this will only execute if the Event Structure timeout is >= 0)"
            n60 = event-data() -> ("NewVal"=w156:path)  [unwired: 1 in, 5 out]
            n61 = Bundle By Name(cluster=w157, "UI.Inkscape File (.svg)"=w156) -> (w158:T23)
            n62 = call <vilib>:"Add State(s) to Queue__jki_lib_state_machine.vi"("State(s) in Front (\"\")"="UI: Update Control >> Ready >> False\nParse: Send File\nConfig: Write\nBig MAQ: Save Background", "State(s) in (\"\")"=w162) -> ("States Out"=w161:string)  [unwired: 13 in]
          }
          event "Background Image": Value Change {
            # "Background: Value Change\n(this will only execute if the Event Structure timeout is >= 0)"
            n63 = event-data() -> ("NewVal"=w164:path)  [unwired: 1 in, 5 out]
            n64 = Bundle By Name(cluster=w165, "UI.Background Image"=w164) -> (w166:T23)
            n65 = call <vilib>:"Add State(s) to Queue__jki_lib_state_machine.vi"("State(s) in Front (\"\")"="UI: Update Control >> Ready >> False\nFile: Background\nBig MAQ: Read Background\nAFM: Background Image\nBig MAQ: Generate Overlay\nBig MAQ: Update\nUI: Update Control >> Ready >> True" ("State(s) in Front (\"\")"), "State(s) in (\"\")"=w170) -> ("States Out"=w169:string)  [unwired: 13 in]
          }
          event "Image Data Range": Value Change {
            # "Image Data Range: Value Change\n(Only the most recent event in the queue is here..."
            n66 = event-data() -> ("NewVal"=w172:cluster{sgl, sgl})  [unwired: 1 in, 5 out]
            n67 = Bundle By Name(cluster=w173, "UI.Image Data Range"=w172) -> (w174:T23)
            n68 = call <vilib>:"Add State(s) to Queue__jki_lib_state_machine.vi"("State(s) in Front (\"\")"="Big MAQ: Change Data Range\nBig MAQ: Update", "State(s) in (\"\")"=w178) -> ("States Out"=w177:string)  [unwired: 13 in]
          }
          event "Page": Value Change {
            # "Image Data Range: Value Change\n(this will only execute if the Event Structure timeout is >= 0)"
            n69 = event-data() -> ("NewVal"=w179:u32)  [unwired: 1 in, 5 out]
            n70 = Bundle By Name(cluster=w180, "UI.Page"=w179) -> (w181:T23)
            n71 = call <vilib>:"Add State(s) to Queue__jki_lib_state_machine.vi"("State(s) in Front (\"\")"="Big MAQ: Select Page\nBig MAQ: Update", "State(s) in (\"\")"=w186) -> ("States Out"=w185:string)  [unwired: 13 in]
          }
          event "Zoom to Fit": Value Change {
            # "Timeout Frame\n(this will only execute if the Event Structure timeout is >= 0)"
            n72 = event-data() -> ()  [unwired: 1 in, 6 out]
            n73 = call <vilib>:"Add State(s) to Queue__jki_lib_state_machine.vi"("State(s) in Front (\"\")"="Big MAQ: Zoom Fit\nUI: Update Zoom Factor", "State(s) in (\"\")"=w192) -> ("States Out"=w191:string)  [unwired: 13 in]
          }
          event "Hide Labels?": Value Change {
            # "Timeout Frame\n(this will only execute if the Event Structure timeout is >= 0)"
            n74 = event-data() -> ("NewVal"=w195:bool)  [unwired: 1 in, 5 out]
            n75 = Bundle By Name(cluster=w193, "UI.Hide Labels"=w195) -> (w194:T23)
            n76 = Select(t="show", s=w195, f="hide") -> (s? t:f=w201:string)
            n77 = call <vilib>:"Build State String with Arguments__JKI_lib_State_Machine.vi"("Arguments (\"\")"=w201, "State"="Big MAQ: Labels") -> ("State with Arguments"=w199:string)  [unwired: 4 in]
            n78 = call <vilib>:"Add State(s) to Queue__jki_lib_state_machine.vi"("State(s) in Front (\"\")"=w199, "State(s) in (\"\")"=w205, "State(s) at Back (\"\")"="Big MAQ: Update" ("State(s) at Back (\"\")")) -> ("States Out"=w204:string)  [unwired: 12 in]
          }
          event User Event {
            # "Timeout Frame\n(this will only execute if the Event Structure timeout is >= 0)"
            n79 = event-data() -> ()  [unwired: 1 in, 5 out]
            n80 = call <vilib>:"Add State(s) to Queue__jki_lib_state_machine.vi"("State(s) in Front (\"\")"="UI: Enable Run >> Enabled\nAFM: Lithography Finished", "State(s) in (\"\")"=w211) -> ("States Out"=w210:string)  [unwired: 13 in]
          }
          event User Event {
            # "Timeout Frame\n(this will only execute if the Event Structure timeout is >= 0)"
            n81 = event-data() -> ("PathsUpdated"=w227:T17)  [unwired: 1 in, 1 out]
            n82 = Unbundle By Name(w223) -> ("selector"=w222:refnum<class "Selector.lvclass">)
            n83 = for {
              tunnel: w227 -> [w235] mode=indexing
              tunnel: [w242] -> w219 mode=indexing
              tunnel: [w233] -> w220 mode=indexing
              shift-right: [w238] -> w215
              shift-left: w226 -> [w234]
              tunnel: [w241] -> w218 mode=indexing
              tunnel: [w239] -> w225 mode=indexing
              n84 = call-dynamic "Read GUID.vi"("error in (no error)"=w234, "ObjectSettings in"=w235) -> ("error out"=w231:errorcluster, "GUID"=w232:string, "ObjectSettings out"=w236:refnum<class "Path Settings.lvclass">)  [unwired: 7 in]
              n85 = call "Query Registry.vi"("error in"=w231, "Name In"=w232) -> ("error out"=w230:errorcluster, "Alias"=w233:string)  [unwired: 6 in, 2 out]
              n86 = call-dynamic "Read Group.vi"("error in (no error)"=w230, "ObjectSettings in"=w236) -> ("error out"=w237:errorcluster, "Group"=w241:string, "ObjectSettings out"=w240:refnum<class "Path Settings.lvclass">)  [unwired: 7 in]
              n87 = call "Read Enabled.vi"("error in (no error)"=w237, "ObjectSettings in"=w240) -> ("error out"=w238:errorcluster, "Enabled"=w242:bool, "ObjectSettings out"=w239:refnum<class "Path Settings.lvclass">)  [unwired: 7 in]
            }
            n88 = Bundle(cluster=T3 {"Groups"=[], "Enable Items"=[]} ("Settings"), "Groups"=w218, "Enable Items"=w219) -> (w217:T3)
            n89 = call "UI--Settings by Name.vi"("error in"=w215, "Settings"=w217, "Names"=w220, "Selector in"=w222) -> ("error out"=w214:errorcluster, "Selector out"=w221:refnum<class "Selector.lvclass">)  [unwired: 6 in]
            n90 = Bundle By Name(cluster=w223, "selector"=w221, "Obj Settings.Paths"=w225) -> (w224:T23)
            n91 = call <vilib>:"Add State(s) to Queue__jki_lib_state_machine.vi"("State(s) in Front (\"\")"="Macro: Objects Updated" ("State(s) in Front (\"\")"), "State(s) in (\"\")"=w229) -> ("States Out"=w228:string)  [unwired: 13 in]
          }
          event User Event {
            # "Timeout Frame\n(this will only execute if the Event Structure timeout is >= 0)"
            n92 = event-data() -> ("RectanglesUpdated"=w246:T18)  [unwired: 1 in, 1 out]
            n93 = Unbundle By Name(w257) -> ("selector"=w256:refnum<class "Selector.lvclass">)
            n94 = for {
              tunnel: w246 -> [w266] mode=indexing
              tunnel: [w273] -> w248 mode=indexing
              tunnel: [w264] -> w247 mode=indexing
              shift-right: [w269] -> w244
              shift-left: w245 -> [w265]
              tunnel: [w272] -> w249 mode=indexing
              tunnel: [w270] -> w243 mode=indexing
              n95 = call-dynamic "Read GUID.vi"("error in (no error)"=w265, "ObjectSettings in"=w266) -> ("error out"=w262:errorcluster, "GUID"=w263:string, "ObjectSettings out"=w267:refnum<class "Rectangle Settings.lvclass">)  [unwired: 7 in]
              n96 = call "Query Registry.vi"("error in"=w262, "Name In"=w263) -> ("error out"=w261:errorcluster, "Alias"=w264:string)  [unwired: 6 in, 2 out]
              n97 = call-dynamic "Read Group.vi"("error in (no error)"=w261, "ObjectSettings in"=w267) -> ("error out"=w268:errorcluster, "Group"=w272:string, "ObjectSettings out"=w271:refnum<class "Rectangle Settings.lvclass">)  [unwired: 7 in]
              n98 = call "Read Enabled.vi"("error in (no error)"=w268, "ObjectSettings in"=w271) -> ("error out"=w269:errorcluster, "Enabled"=w273:bool, "ObjectSettings out"=w270:refnum<class "Rectangle Settings.lvclass">)  [unwired: 7 in]
            }
            n99 = Bundle(cluster=T3 {"Groups"=[], "Enable Items"=[]} ("Settings"), "Groups"=w249, "Enable Items"=w248) -> (w254:T3)
            n100 = call "UI--Settings by Name.vi"("error in"=w244, "Settings"=w254, "Names"=w247, "Selector in"=w256) -> ("error out"=w252:errorcluster, "Selector out"=w255:refnum<class "Selector.lvclass">)  [unwired: 6 in]
            n101 = Bundle By Name(cluster=w257, "selector"=w255, "Obj Settings.Rectangles"=w243) -> (w258:T23)
            n102 = call <vilib>:"Add State(s) to Queue__jki_lib_state_machine.vi"("State(s) in Front (\"\")"="Macro: Objects Updated" ("State(s) in Front (\"\")"), "State(s) in (\"\")"=w260) -> ("States Out"=w259:string)  [unwired: 13 in]
          }
          event User Event {
            # "Timeout Frame\n(this will only execute if the Event Structure timeout is >= 0)"
            n103 = event-data() -> ("FunnelsUpdated"=w277:T19)  [unwired: 1 in]
            n104 = Unbundle By Name(w288) -> ("selector"=w287:refnum<class "Selector.lvclass">)
            n105 = for {
              tunnel: w277 -> [w297] mode=indexing
              tunnel: [w304] -> w279 mode=indexing
              tunnel: [w295] -> w278 mode=indexing
              shift-right: [w300] -> w274
              shift-left: w276 -> [w296]
              tunnel: [w303] -> w280 mode=indexing
              tunnel: [w301] -> w275 mode=indexing
              n106 = call-dynamic "Read GUID.vi"("error in (no error)"=w296, "ObjectSettings in"=w297) -> ("error out"=w293:errorcluster, "GUID"=w294:string, "ObjectSettings out"=w298:refnum<class "Funnel Settings.lvclass">)  [unwired: 7 in]
              n107 = call "Query Registry.vi"("error in"=w293, "Name In"=w294) -> ("error out"=w292:errorcluster, "Alias"=w295:string)  [unwired: 6 in, 2 out]
              n108 = call-dynamic "Read Group.vi"("error in (no error)"=w292, "ObjectSettings in"=w298) -> ("error out"=w299:errorcluster, "Group"=w303:string, "ObjectSettings out"=w302:refnum<class "Funnel Settings.lvclass">)  [unwired: 7 in]
              n109 = call "Read Enabled.vi"("error in (no error)"=w299, "ObjectSettings in"=w302) -> ("error out"=w300:errorcluster, "Enabled"=w304:bool, "ObjectSettings out"=w301:refnum<class "Funnel Settings.lvclass">)  [unwired: 7 in]
            }
            n110 = Bundle(cluster=T3 {"Groups"=[], "Enable Items"=[]} ("Settings"), "Groups"=w280, "Enable Items"=w279) -> (w285:T3)
            n111 = call "UI--Settings by Name.vi"("error in"=w274, "Settings"=w285, "Names"=w278, "Selector in"=w287) -> ("error out"=w283:errorcluster, "Selector out"=w286:refnum<class "Selector.lvclass">)  [unwired: 6 in]
            n112 = Bundle By Name(cluster=w288, "selector"=w286, "Obj Settings.Funnels"=w275) -> (w289:T23)
            n113 = call <vilib>:"Add State(s) to Queue__jki_lib_state_machine.vi"("State(s) in Front (\"\")"="Macro: Objects Updated" ("State(s) in Front (\"\")"), "State(s) in (\"\")"=w291) -> ("States Out"=w290:string)  [unwired: 13 in]
          }
          event User Event {
            # "Timeout Frame\n(this will only execute if the Event Structure timeout is >= 0)"
            n114 = event-data() -> ("DotsUpdated"=w305:T20)  [unwired: 1 in]
            n115 = Unbundle By Name(w319) -> ("selector"=w318:refnum<class "Selector.lvclass">)
            n116 = for {
              tunnel: [w335] -> w309 mode=indexing
              tunnel: [w327] -> w311 mode=indexing
              shift-right: [w331] -> w307
              shift-left: w306 -> [w328]
              tunnel: [w334] -> w310 mode=indexing
              tunnel: [w332] -> w308 mode=indexing
              tunnel: w305 -> [w323] mode=indexing
              n117 = call-dynamic "Read GUID.vi"("error in (no error)"=w328, "ObjectSettings in"=w323) -> ("error out"=w325:errorcluster, "GUID"=w326:string, "ObjectSettings out"=w329:refnum<class "Dot Settings.lvclass">)  [unwired: 7 in]
              n118 = call "Query Registry.vi"("error in"=w325, "Name In"=w326) -> ("error out"=w324:errorcluster, "Alias"=w327:string)  [unwired: 6 in, 2 out]
              n119 = call-dynamic "Read Group.vi"("error in (no error)"=w324, "ObjectSettings in"=w329) -> ("error out"=w330:errorcluster, "Group"=w334:string, "ObjectSettings out"=w333:refnum<class "Dot Settings.lvclass">)  [unwired: 7 in]
              n120 = call "Read Enabled.vi"("error in (no error)"=w330, "ObjectSettings in"=w333) -> ("error out"=w331:errorcluster, "Enabled"=w335:bool, "ObjectSettings out"=w332:refnum<class "Dot Settings.lvclass">)  [unwired: 7 in]
            }
            n121 = Bundle(cluster=T3 {"Groups"=[], "Enable Items"=[]} ("Settings"), "Groups"=w310, "Enable Items"=w309) -> (w316:T3)
            n122 = call "UI--Settings by Name.vi"("error in"=w307, "Settings"=w316, "Names"=w311, "Selector in"=w318) -> ("error out"=w314:errorcluster, "Selector out"=w317:refnum<class "Selector.lvclass">)  [unwired: 6 in]
            n123 = Bundle By Name(cluster=w319, "selector"=w317, "Obj Settings.Dots"=w308) -> (w320:T23)
            n124 = call <vilib>:"Add State(s) to Queue__jki_lib_state_machine.vi"("State(s) in Front (\"\")"="Macro: Objects Updated" ("State(s) in Front (\"\")"), "State(s) in (\"\")"=w322) -> ("States Out"=w321:string)  [unwired: 13 in]
          }
          event User Event {
            n125 = event-data() -> ("Paths"=w341:refnum<class "Tool Path.lvclass">[], "Funnels"=w340:refnum<class "Tool Funnel.lvclass">[], "Rectangles"=w339:refnum<class "Tool Rectangle.lvclass">[], "Dots"=w338:refnum<class "Tool Dots.lvclass">[])  [unwired: 1 in, 4 out]
            n126 = Unbundle By Name(w347) -> ("tooler"=w345:refnum<class "Tool Data.lvclass">)
            n127 = property class="Tool Data.lvclass"(reference=w345) -> (reference out=w346:refnum<class "Tool Data.lvclass">, "Accessors:Tooled"=w343:T25)  [unwired: 1 in, 1 out]
            n128 = Bundle By Name(cluster=w343, "Paths"=w341, "Funnels"=w340, "Rectangles"=w339, "Dots"=w338) -> (w342:T25)
            n129 = property class="Tool Data.lvclass"(reference=w346, "Accessors:Tooled"=w342) -> (reference out=w344:refnum<class "Tool Data.lvclass">)  [unwired: 1 in, 1 out]
            n130 = Bundle By Name(cluster=w347, "tooler"=w344) -> (w348:T23)
            n131 = call <vilib>:"Add State(s) to Queue__jki_lib_state_machine.vi"("State(s) in Front (\"\")"="UI: Update Control >> Ready >> False\nTool: Generate Litho Data\nSelect: Order Litho\nBig MAQ: Coerce Size\nBig MAQ: Generate Overlay\nBig MAQ: Update\nAFM: Lithography Data\nUI: Update Control >> Ready >> True" ("State(s) in Front (\"\")"), "State(s) in (\"\")"=w351) -> ("States Out"=w350:string)  [unwired: 13 in]
          }
          event User Event {
            # "Timeout Frame\n(this will only execute if the Event Structure timeout is >= 0)"
            n132 = event-data() -> ("Paths"=w355:refnum<class "Path.lvclass">[], "Rectangles"=w356:refnum<class "Rectangle.lvclass">[], "Background"=w357:refnum<class "SVGImage.lvclass">, "Dots"=w358:refnum<class "Dot.lvclass">[], "Other Images"=w352:refnum<class "SVGImage.lvclass">[])  [unwired: 1 in]
            n133 = Bundle By Name(cluster=w359, "Parsed Obj.Paths"=w355, "Parsed Obj.Rectangles"=w356, "Parsed Obj.Background"=w357, "Parsed Obj.Dots"=w358, "Parsed Obj.Other Images"=w352) -> (w360:T23)
            n134 = call <vilib>:"Add State(s) to Queue__jki_lib_state_machine.vi"("State(s) in Front (\"\")"="Tool: Sort Paths\nTool: Get IDs\nIdentity: Populate\nSelect: New Name Set\nSelect: Update\nSettings: Refresh\nSelect: Change By Name >> First", "State(s) in (\"\")"=w363) -> ("States Out"=w362:string)  [unwired: 13 in]
          }
          event "MCLB": Value Change {
            n135 = event-data() -> ()  [unwired: 1 in, 6 out]
            n136 = Unbundle By Name(w375) -> ("selector"=w374:refnum<class "Selector.lvclass">)
            n137 = call "Event--Value Change.vi"("error in"=w372, "Selector in"=w374) -> ("error out"=w367:errorcluster, "Name"=w368:string, "Selector out"=w373:refnum<class "Selector.lvclass">)  [unwired: 7 in]
            n138 = Bundle By Name(cluster=w375, "selector"=w373) -> (w376:T23)
            n139 = Search and Replace String(replace all?=TRUE ("replace all? (F)"), input string="Select: Reorder\nSettings: Set Active >> <state>\nSubpanel: Insert >> <state>" ("State(s) in Front (\"\")"), search string="<state>", replace string=w368, error in=w367) -> (result string=w365:string, error out=w366:errorcluster)  [unwired: 3 in, 2 out]
            n140 = call <vilib>:"Add State(s) to Queue__jki_lib_state_machine.vi"("State(s) in Front (\"\")"=w365, "State(s) in (\"\")"=w378) -> ("States Out"=w377:string)  [unwired: 13 in]
          }
          event "MCLB": Mouse Down? {
            n141 = event-data() -> ("Coords"=w390:T24, "Button"=w389:u16, "PlatMods"=w388:T26)  [unwired: 1 in]
            n142 = Unbundle By Name(w394) -> ("selector"=w393:refnum<class "Selector.lvclass">)
            n143 = Bundle By Name(cluster=T5 {"Point"={"Left"=0, "Top"=0}, "Button"=0, "PlatMods"={"Shift"=FALSE, "Ctrl"=FALSE, "Alt"=FALSE, "Cmd"=FALSE, "Opt"=FALSE}} ("Event Data"), "Point"=w390, "Button"=w389, "PlatMods"=w388) -> (w387:T5)
            n144 = call "Event--Mouse Down.vi"("error in"=w385, "Event Data"=w387, "Selector in"=w393) -> ("error out"=w386:errorcluster, "Enable Change"=w383:bool, "Name"=w381:string, "Selector out"=w392:refnum<class "Selector.lvclass">)  [unwired: 5 in]
            n145 = call <vilib>:"Build State String with Arguments__JKI_lib_State_Machine.vi"("Arguments (\"\")"=w381, "State"="Settings: Change Enable") -> ("State with Arguments"=w382:string)  [unwired: 4 in]
            n146 = Select(t=w382, s=w383, f="" ("State(s) in Front (\"\")")) -> (s? t:f=w379:string)
            n147 = Bundle By Name(cluster=w394, "selector"=w392) -> (w395:T23)
            n148 = event-data("Discard?"=w383) -> ()  [unwired: 1 in, 1 out]
            n149 = call <vilib>:"Add State(s) to Queue__jki_lib_state_machine.vi"("State(s) in Front (\"\")"=w379, "State(s) in (\"\")"=w397) -> ("States Out"=w396:string)  [unwired: 13 in]
          }
          event "MCLB": Drag Ended {
            n150 = event-data() -> ()  [unwired: 1 in, 5 out]
            n151 = Unbundle By Name(w403) -> ("selector"=w401:refnum<class "Selector.lvclass">)
            n152 = call "Event--Drag Ended.vi"("error in"=w398, "Selector in"=w401) -> ("error out"=w399:errorcluster, "Selector out"=w400:refnum<class "Selector.lvclass">)  [unwired: 8 in]
            n153 = Bundle By Name(cluster=w403, "selector"=w400) -> (w404:T23)
            n154 = call <vilib>:"Add State(s) to Queue__jki_lib_state_machine.vi"("State(s) in Front (\"\")"="Select: Reorder\nSelect: Order Litho" ("State(s) in Front (\"\")"), "State(s) in (\"\")"=w406) -> ("States Out"=w405:string)  [unwired: 13 in]
          }
          event "MCLB": Shortcut Menu Activation? {
            n155 = event-data() -> ("MenuRef"=w408:refnum<k9>, "Coords"=w407:T24)  [unwired: 1 in, 5 out]
            n156 = Unbundle By Name(w414) -> ("selector"=w412:refnum<class "Selector.lvclass">)
            n157 = call "Event--Shortcut Menu Activation.vi"("error in"=w409, "Coords"=w407, "MenuRef"=w408, "Selector in"=w412) -> ("error out"=w410:errorcluster, "Selector out"=w411:refnum<class "Selector.lvclass">)  [unwired: 6 in]
            n158 = Bundle By Name(cluster=w414, "selector"=w411) -> (w415:T23)
            n159 = event-data() -> ()  [unwired: 2 in, 1 out]
            n160 = call <vilib>:"Add State(s) to Queue__jki_lib_state_machine.vi"("State(s) in Front (\"\")"="" ("State(s) in Front (\"\")"), "State(s) in (\"\")"=w417) -> ("States Out"=w416:string)  [unwired: 13 in]
          }
          event "MCLB": Shortcut Menu Selection (User) {
            n161 = event-data() -> ("ItemPath"=w422:string)  [unwired: 1 in]
            n162 = Unbundle By Name(w427) -> ("selector"=w426:refnum<class "Selector.lvclass">)
            n163 = call "Event--Shortcut Menu Selection.vi"("error in"=w423, "ItemPath"=w422, "Selector in"=w426) -> ("error out"=w424:errorcluster, "Selection"=w421:string, "Selector out"=w425:refnum<class "Selector.lvclass">)  [unwired: 6 in]
            n164 = call <vilib>:"Build State String with Arguments__JKI_lib_State_Machine.vi"("Arguments (\"\")"=w421, "State"="Select: Group" ("State(s) in Front (\"\")")) -> ("State with Arguments"=w419:string)  [unwired: 4 in]
            n165 = Bundle By Name(cluster=w427, "selector"=w425) -> (w428:T23)
            n166 = call <vilib>:"Add State(s) to Queue__jki_lib_state_machine.vi"("State(s) in Front (\"\")"=w419, "State(s) in (\"\")"=w430) -> ("States Out"=w429:string)  [unwired: 13 in]
          }
          event Panel Close? {
            # "Discard the event because we'll close the front panel ourselves in Macro: Exit"
            # "Close Panel button (pressed) Event\n(this executes Macro: Exit to terminate the VI)"
            n167 = event-data() -> ()  [unwired: 1 in, 1 out]
            n168 = event-data("Discard?"=TRUE) -> ()  [unwired: 1 in, 1 out]
            n169 = call <vilib>:"Add State(s) to Queue__jki_lib_state_machine.vi"("State(s) in Front (\"\")"="Macro: Exit", "State(s) in (\"\")"=w436) -> ("States Out"=w435:string)  [unwired: 13 in]
          }
        }
      }
      frame "---------- Core ----------" {
        # "Do not put any code in this frame.\n(it is a separator no-op)"
        n170 = call <vilib>:"Add State(s) to Queue__jki_lib_state_machine.vi"("State(s) in (\"\")"=w441) -> ("States Out"=w440:string)  [unwired: 14 in]
      }
      frame Default {
        w452 = 42 items=["No error", "Argument error", "Memory is full", "Out of zone", "End of file", "File already open", "Generic file I/O error", "File not found", "File permission error", "Disk is full", "Duplicate path", "Too many files open", "System feature not enabled", "Resource file not found", "Cannot add resource", "Resource not found", "Image not found", "Image memory error", "Pen does not exist", "Config type invalid", "Config token not found", "Config parse error", "Config memory error", "Bad external code format", "Bad external code offset", "External code not present", "Null window", "Destroy window error", "Null menu", "Print aborted", "Bad print record", "Print driver error", "Windows error during printing", "Memory error during printing", "Print dialog error", "Generic print error", "Invalid device refnum", "Device not found", "Device parameter error", "Device unit error", "Cannot open device", "Device call aborted", "Generic error", "Cancelled by user", "Object ID too low", "Object ID too high", "Object not in heap", "Unknown heap", "Unknown object (invalid DefProc)", "Unknown object (DefProc not in table)", "Message out of range", "Invalid (null) method", "Unknown message", "Manager call not supported", "Bad address", "Network operation in progress", "Network operation timed out", "Connection is busy", "Network attribute not supported", "Network error", "Address in use", "System out of memory", "Connection aborted", "Connection refused", "Not connected", "Already connected", "Connection closed", "Initialization error (interapplication manager)", "Bad occurrence", "Wait on unbound occurrence handler", "Occurrence queue overflow", "Datalog type conflict", "Unused", "Unrecognized type (interapplication manager)", "Memory corrupt", "Failed to make temporary DLL", "Old CIN version", "Drag socket not found", "Failed to load drop-object", "Failed to register OLE object", "Failed to release OLE object", "Format specifier type mismatch", "Unknown format specifier", "Too few format specifiers", "Too many format specifiers", "Scan failed", "Newer CIN version", "Error converting to variant", "Runtime menu error", "Password tampered", "Variant attribute not found", "Incompatible variant data type", "Event data is not available", "Event Store is not present", "Occurrence is not found", "Event Queue is not created", "Event info is not available", "Refnum passed is NULL", "Error retrieving Class GUID", "Error retrieving CoClass GUID", "Error retrieving TypeLib GUID.", "Bad built application magic bytes.", "Specific driver is different from the specific driver associated with the Logical Name.", "There is no session opened to the class driver.", "Max Error", "MAX - Error with config objects", "MAX - Error loading configuration", "MAX - Group not supported"]
        # "State Syntax:\nStateCategory: State >> Argument\nLine Terminator: Line feed\nExample:\nUI: Help >> About\n\nWhere \"UI\" is the state category\nWhere \"Help\" is the state\nWhere \"About\" is the argument\nOther Examples:\nApp Data: Initialize\nUI: Initialize\nHelp >> About\n\nCommenting:\nTo add a comment use \"//\" or \"#\" and all text to the right will be ignored\nCommenting Example:\nUI: Initialize // This initializes the UI\n# This whole line is a comment\n// Another comment line"
        # "Current State"
        # "Do not delete, rename, or modify this frame.\n(this is used to capture unhandled states and typos)"
        # "Handle mistyped state name (developer tool)"
        n171 = Format Into String(format string="Software Exception: Unhandled State \"%s\"." ("message"), error in=w448, w443) -> (resulting string=w451:string, error out=w450:errorcluster)  [unwired: 1 in]
        n172 = call <vilib>:"Error Cluster From Error Code.vi"("show call chain? (False)"=TRUE, "error in (no error)"=w450, "error message (\"\")"=w451, "error code (0)"=w452) -> ("error out"=w449:errorcluster)  [unwired: 5 in]
        n173 = call <vilib>:"Add State(s) to Queue__jki_lib_state_machine.vi"("State(s) in (\"\")"=w447) -> ("States Out"=w446:string)  [unwired: 14 in]
      }
      frame "Initialize Core Data" {
        # "Do not delete, rename, or modify this frame.\n(this is used to determine panel behavior on exit)"
        # "originally closed?"
        # "exe?"
        # "If panel starts closed or is an EXE, then close it when we exit"
        n174 = property class="VI"() -> ("FP.State"=w458:T6)  [unwired: 2 in, 2 out]
        n175 = property class="App"() -> ("App.Kind"=w464:T7)  [unwired: 2 in, 2 out]
        n176 = control-ref of="Current VI Reference"() -> (w459:refnum<vi>)
        n177 = Equal?(x=w458, y=T6."Closed" ("Front Panel Window:State")) -> (x = y?=w456:bool)
        n178 = Equal?(x=w464, y=T7."Run Time System" ("Application:Kind")) -> (x = y?=w462:bool)
        n179 = Or(x=w456, y=w462) -> (x .or. y?=w460:bool)
        n180 = Bundle By Name(cluster=w461, "Core.Current VI Reference"=w459, "Core.Close Panel on Exit?"=w460) -> (w466:T23)
        n181 = call <vilib>:"Add State(s) to Queue__jki_lib_state_machine.vi"("State(s) in (\"\")"=w468) -> ("States Out"=w467:string)  [unwired: 14 in]
      }
      frame "Error Handler" {
        # "Unhandled Error -- Display it"
        # "Handle any errors here.\nYou can also output any states to clean-up after errors occur"
        # "Clear error"
        n182 = call <vilib>:"General Error Handler.vi"("error in (no error)"=w471) -> ()  [unwired: 10 in, 5 out]
        n183 = call <vilib>:"Add State(s) to Queue__jki_lib_state_machine.vi"("State(s) in Front (\"\")"="/* Post Error States", "State(s) in (\"\")"=w475) -> ("States Out"=w474:string)  [unwired: 13 in]
      }
      frame "Exit" {
        # "Do not put any code in this frame.\n(No errors that occur here will be handled.)"
        n184 = call <vilib>:"Add State(s) to Queue__jki_lib_state_machine.vi"("State(s) in (\"\")"=w481) -> ("States Out"=w480:string)  [unwired: 14 in]
      }
      frame "---------- Data ----------" {
        # "Do not put any code in this frame.\n(It is a separator no-op. You can make a copy of this frame to create a new Data frame)"
        n185 = call <vilib>:"Add State(s) to Queue__jki_lib_state_machine.vi"("State(s) in (\"\")"=w486) -> ("States Out"=w485:string)  [unwired: 14 in]
      }
      frame "Data: Status" {
        # "Data: Status\nInitialize the FGV with the name of the state for the status string"
        n186 = flat-sequence {
          tunnel: [w496] -> w488
          tunnel: w489 -> [w496]
          tunnel: [w494] -> _
          frame #0 {
            n187 = call "Status State.vi"("Status State In"="UI: Status", "Write"=TRUE) -> ("Status State Out"=w494:string)  [unwired: 3 in]
          }
        }
        n188 = call <vilib>:"Add State(s) to Queue__jki_lib_state_machine.vi"("State(s) in (\"\")"=w493) -> ("States Out"=w492:string)  [unwired: 14 in]
      }
      frame "Data: Initialize" {
        w498 = cluster{"X":sgl, "Y":sgl}[] []  # Zoom History
        w499 = ""  # Offline Log
        w500 = refnum<class "Log.Litho.lvclass"> refnum  # log
        w501 = refnum<class "Inset.lvclass"> refnum  # inset
        w502 = T27 {"Hide Labels"=FALSE, "Image Data Range"={100.0, 0.0}, "Status"="", "Autosave Path"=path "", "Autosave?"=FALSE, "Inkscape File (.svg)"=path "", "Background Image"=path "", "Page"=0, "Normal Save Path"=path ""}  # UI
        w503 = path ""  # root path
        w506 = T28 []  # Litho
        w507 = T29 {"Paths"=[], "Rectangles"=[], "Background"=refnum, "Dots"=[], "Funnels"=[], "Other Images"=[]}  # Parsed Obj
        w508 = T30 {"Dots"=[], "Funnels"=[], "Rects"=[], "Paths"=[]}  # GUIDs
        w509 = T31 {"Path Changes"=[], "Funnel Changes"=[], "Rectangle Changes"=[], "Dot Changes"=[]}  # Changed Obj
        w510 = T32 {"Rectangles"=[], "Paths"=[], "Funnels"=[], "Dots"=[]}  # Obj Settings
        w512 = refnum<class "Configuration.lvclass"> refnum  # config
        w511 = refnum<class "AFM_Driver_Manager.lvclass"> refnum  # afm_mngr
        w515 = refnum<class "Selector.lvclass"> refnum  # selector
        w513 = refnum<class "BigMAQ.lvclass"> refnum  # big-maq
        w514 = refnum<class "Subpanel.Edit.lvclass"> refnum  # sbpnl.edit
        w518 = refnum<class "Tool Data.lvclass"> refnum  # tooler
        w516 = refnum<class "Setting Database.lvclass"> refnum  # settings
        w517 = refnum<class "ParseVectorFile.lvclass"> refnum  # parser
        w519 = T33 {"Current VI Reference"=refnum, "Close Panel on Exit?"=FALSE}  # Core
        # "do not delete - used by framework"
        # "Data names and types of shift register data are defined by this bundle."
        # "Initialize the shift-register data, here.\n(data names are defined by what you wire into the bundle function)"
        n189 = Bundle("Core"=w519, "tooler"=w518, "parser"=w517, "settings"=w516, "selector"=w515, "sbpnl.edit"=w514, "big-maq"=w513, "config"=w512, "afm_mngr"=w511, "Obj Settings"=w510, "Changed Obj"=w509, "GUIDs"=w508, "Parsed Obj"=w507, "Litho"=w506, "root path"=w503, "UI"=w502, "inset"=w501, "log"=w500, "Offline Log"=w499, "Zoom History"=w498) -> (w521:T23)  [unwired: 1 in]
        n190 = call <vilib>:"Add State(s) to Queue__jki_lib_state_machine.vi"("State(s) in (\"\")"=w523) -> ("States Out"=w522:string)  [unwired: 14 in]
      }
      frame "Data: Cleanup" {
        # "Cleanup any data and references, here.\n(this is called automatically, by the Macro: Exit)"
        n191 = Unbundle By Name(w525) -> ("Core.Current VI Reference"=w528:refnum<vi>)
        n192 = Close Reference(reference=w528, error in (no error)=w527) -> (error out=w526:errorcluster)
        n193 = call <vilib>:"Add State(s) to Queue__jki_lib_state_machine.vi"("State(s) in (\"\")"=w530) -> ("States Out"=w529:string)  [unwired: 14 in]
      }
      frame "---------- Events ----------" {
        # "Do not put any code in this frame.\n(It is a separator no-op. You can make a copy of this frame to create a new UI frame)"
        n194 = call <vilib>:"Add State(s) to Queue__jki_lib_state_machine.vi"("State(s) in (\"\")"=w535) -> ("States Out"=w534:string)  [unwired: 14 in]
      }
      frame "Events: Register" {
        # "Do not put any code in this frame.\n(It is a separator no-op. You can make a copy of this frame to create a new UI frame)"
        n195 = Unbundle By Name(w551) -> ("tooler"=w550:refnum<class "Tool Data.lvclass">, "parser"=w549:refnum<class "ParseVectorFile.lvclass">, "settings"=w548:refnum<class "Setting Database.lvclass">, "afm_mngr"=w539:refnum<class "AFM_Driver_Manager.lvclass">)
        n196 = call "AFM_Driver_Manager.GetPublicEvents.vi"("AFM_Driver_Manager in"=w539) -> ("error out"=w538:errorcluster, "AFM_Driver Events"=w537:T34)  [unwired: 8 in, 1 out]
        n197 = call "Setting Database.GetPublicEvents.vi"("Setting Database"=w548) -> ("error out"=w544:errorcluster, "Public Events"=w543:T35)  [unwired: 8 in, 1 out]
        n198 = call "ParseVectorFile.GetPublicEvents.vi"("ParseVectorFile"=w549) -> ("error out"=w545:errorcluster, "Public Events"=w542:T36)  [unwired: 8 in, 1 out]
        n199 = call "Tool Data.GetPublicEvents.vi"("Tool Data"=w550) -> ("error out"=w546:errorcluster, "Public Events"=w541:T37)  [unwired: 8 in, 1 out]
        n200 = register-events(w541, w542, w543, w537) -> (reference out=w553:refnum<event-registration>, error out=w552:errorcluster)  [unwired: 2 in]
        n201 = Merge Errors(w540, w552, w546, w545, w544, w538) -> (w547:errorcluster)
        n202 = call <vilib>:"Add State(s) to Queue__jki_lib_state_machine.vi"("State(s) in (\"\")"=w555) -> ("States Out"=w554:string)  [unwired: 14 in]
      }
      frame "Events: Unregister" {
        # "Do not put any code in this frame.\n(It is a separator no-op. You can make a copy of this frame to create a new UI frame)"
        n203 = Unregister For Events(event registration refnum=w559, error in=w558) -> (error out=w557:errorcluster)
        n204 = call <vilib>:"Add State(s) to Queue__jki_lib_state_machine.vi"("State(s) in (\"\")"=w562) -> ("States Out"=w561:string)  [unwired: 14 in]
      }
      frame "---------- UI ----------" {
        # "Do not put any code in this frame.\n(It is a separator no-op. You can make a copy of this frame to create a new UI frame)"
        n205 = call <vilib>:"Add State(s) to Queue__jki_lib_state_machine.vi"("State(s) in (\"\")"=w567) -> ("States Out"=w566:string)  [unwired: 14 in]
      }
      frame "UI: Create Insert" {
        # "Do not put any code in this frame.\n(It is a separator no-op. You can make a copy of this frame to create a new UI frame)"
        n206 = Unbundle By Name(w592) -> ("inset"=w587:refnum<class "Inset.lvclass">, "UI.Image Data Range"=w584:cluster{sgl, sgl}, "UI.Page"=w583:u32, "big-maq"=w586:refnum<class "BigMAQ.lvclass">, "UI.Inkscape File (.svg)"=w581:path, "Parsed Obj.Background"=w580:refnum<class "SVGImage.lvclass">)
        n207 = Bundle(cluster=T8 {"Background.Range"={0.0, 100.0}, "Background.Page"=0} ("Display Settings"), "Background.Range"=w584, "Background.Page"=w583) -> (w582:T8)
        n208 = call "Setup Background BigMAQ.vi"("error in"=w575, "BigMAQ"=w586, "Display Settings"=w582, "Inset in"=w587) -> ("error out"=w578:errorcluster, "Inset out"=w591:refnum<class "Inset.lvclass">)  [unwired: 6 in]
        n209 = call "Write SVG Path.vi"("error in"=w578, "Path"=w581, "Inset in"=w591) -> ("error out"=w577:errorcluster, "Inset out"=w590:refnum<class "Inset.lvclass">)  [unwired: 7 in]
        n210 = call-dynamic "Read id.vi"("error in (no error)"=w577, "SVG Object in"=w580) -> ("error out"=w576:errorcluster, "id"=w579:string)  [unwired: 7 in, 1 out]
        n211 = call "Set Background id.vi"("error in"=w576, "id"=w579, "Inset in"=w590) -> ("error out"=w588:errorcluster, "Inset out"=w589:refnum<class "Inset.lvclass">)  [unwired: 7 in]
        n212 = call "User Interface.vi"("error in"=w588, "Inset In"=w589) -> ("error out"=w572:errorcluster, "Inset Out"=w574:refnum<class "Inset.lvclass">)  [unwired: 8 in]
        n213 = call "Get Background Settings.vi"("error in"=w572, "Inset in"=w574) -> ("error out"=w571:errorcluster, "Background.Page"=w569:i32, "Background.Range"=w570:cluster{sgl, sgl}, "Inset out"=w573:refnum<class "Inset.lvclass">)  [unwired: 6 in]
        n214 = Bundle By Name(cluster=w592, "inset"=w573, "UI.Image Data Range"=w570, "UI.Page"=w569) -> (w593:T23)
        n215 = call <vilib>:"Add State(s) to Queue__jki_lib_state_machine.vi"("State(s) in Front (\"\")"="UI: Update Control >> Image Data Range\nUI: Update Control>>Page\nBig MAQ: Select Page\nBig MAQ: Change Data Range\nBig MAQ: Update" ("State(s) in Front (\"\")"), "State(s) in (\"\")"=w597) -> ("States Out"=w596:string)  [unwired: 13 in]
      }
      frame "UI: Update Zoom Factor" {
        # "Do not put any code in this frame.\n(It is a separator no-op. You can make a copy of this frame to create a new UI frame)"
        n216 = control-ref of="Render"() -> (w602:refnum<vi>)
        n217 = property class="ImageControl"(reference=w602) -> ("X Zoom"=w598:sgl)  [unwired: 1 in, 2 out]
        n218 = Format Into String(format string="%3.1f", initial string="", w598) -> (resulting string=w605:string)  [unwired: 1 in, 1 out]
        n219 = Concatenate Strings(w605, "x" ("string")) -> (w601:string)
        n220 = local write "Zoom"(w601) -> ()
        n221 = call <vilib>:"Add State(s) to Queue__jki_lib_state_machine.vi"("State(s) in (\"\")"=w610) -> ("States Out"=w609:string)  [unwired: 14 in]
      }
      frame "UI: Select Initialize" {
        # "Do not put any code in this frame.\n(It is a separator no-op. You can make a copy of this frame to create a new UI frame)"
        n222 = Unbundle By Name(w614) -> ("selector"=w613:refnum<class "Selector.lvclass">)
        n223 = call "UI--Initialize.vi"("error in"=w615, "Selector in"=w613) -> ("error out"=w616:errorcluster, "Selector out"=w612:refnum<class "Selector.lvclass">)  [unwired: 8 in]
        n224 = Bundle By Name(cluster=w614, "selector"=w612) -> (w617:T23)
        n225 = call <vilib>:"Add State(s) to Queue__jki_lib_state_machine.vi"("State(s) in (\"\")"=w620) -> ("States Out"=w619:string)  [unwired: 14 in]
      }
      frame "UI: Enable Run" {
        # "Do not put any code in this frame.\n(It is a separator no-op. You can make a copy of this frame to create a new UI frame)"
        n226 = Match True/False String(2:"Disabled" ("false string"), 3:"Enabled" ("true string"), 4:w624) -> (0:w631:bool)  [unwired: 1 out]
        n227 = Select(t=T9."Enabled" ("Disabled"), s=w631, f=T9."Disabled and Grayed Out" ("Disabled")) -> (s? t:f=w630:T9)
        n228 = control-ref of="Run"() -> (w625:refnum<vi>)
        n229 = property class="Bool (strict)"(reference=w625, error in=w622, "DisabledEnum"=w630) -> (error out=w623:errorcluster)  [unwired: 1 out]
        n230 = call <vilib>:"Add State(s) to Queue__jki_lib_state_machine.vi"("State(s) in (\"\")"=w635) -> ("States Out"=w634:string)  [unwired: 14 in]
      }
      frame "UI: Status" {
        w640 = "\r\n"
        # "This must be empty string otherwise you will get stuck"
        # "Do not put any code in this frame.\n(It is a separator no-op. You can make a copy of this frame to create a new UI frame)"
        n231 = Unbundle By Name(w648) -> ("UI.Status"=w643:string, "log"=w636:refnum<class "Log.Litho.lvclass">)
        n232 = Format Date/Time String(time format string (%c)="%H:%M:%S --") -> (date/time string=w657:string)  [unwired: 2 in]
        n233 = call <vilib>:"GetState.vi"("error in (no error)"=w646, "SMO"=w636) -> ("error out"=w644:errorcluster, "SMO State"=w647:T38, "SMO out"=w645:refnum<class "Log.Litho.lvclass">)  [unwired: 7 in]
        n234 = Concatenate Strings(w657, "\t", w642) -> (w641:string)
        n235 = case shown="\"Started\"" w647 {
          tunnel: w645 -> [w667 w672]
          tunnel: w644 -> [w666 w669]
          tunnel: w641 -> [w663 w668]
          tunnel: [w665 w671] -> w637
          tunnel: [w664 w670] -> w638
          frame Default {
            n236 = call <vilib>:"Clear Errors.vi"("error in (no error)"=w666) -> ("error out"=w662:errorcluster)  [unwired: 5 in, 1 out]
            n237 = call-dynamic "Write Offline Log.vi"("error in (no error)"=w662, "Offline Log"=w663, "Log.Litho in"=w667) -> ("error out"=w664:errorcluster, "Log.Litho out"=w665:refnum<class "Log.Litho.lvclass">)  [unwired: 7 in]
          }
          frame "Started" {
            n238 = call "Log.Litho.Activity.vi"("error in (no error)"=w669, "Activity"=w668, "Log.Litho"=w672) -> ("error out"=w670:errorcluster, "Log.Litho out"=w671:refnum<class "Log.Litho.lvclass">)  [unwired: 7 in]
          }
        }
        n239 = Concatenate Strings(w641, w640, w643) -> (w639:string)
        n240 = call <vilib>:"Delimited String to 1D String Array.vi"("delimiter"=w640, "delimited string"=w639) -> ("string array"=w655:string[])  [unwired: 9 in]
        n241 = Array Subset(array=w655, index=0, length=2000) -> (w652:string[])
        n242 = call <vilib>:"1D String Array to Delimited String.vi"("delimiter"=w640, "string array"=w652) -> ("delimited string"=w650:string)  [unwired: 9 in]
        n243 = local write "Status"(w650) -> ()
        n244 = Bundle By Name(cluster=w648, "UI.Status"=w650, "log"=w637) -> (w651:T23)
        n245 = call <vilib>:"Add State(s) to Queue__jki_lib_state_machine.vi"("State(s) in (\"\")"=w661) -> ("States Out"=w660:string)  [unwired: 14 in]
      }
      frame "UI: Big MAQ Initialize" {
        # "Do not put any code in this frame.\n(It is a separator no-op. You can make a copy of this frame to create a new UI frame)"
        n246 = Unbundle By Name(w677) -> ("big-maq"=w679:refnum<class "BigMAQ.lvclass">)
        n247 = call "Initialize UI.vi"("error in"=w674, "BigMAQ in"=w679) -> ("error out"=w675:errorcluster, "BigMAQ out"=w676:refnum<class "BigMAQ.lvclass">)  [unwired: 8 in]
        n248 = Bundle By Name(cluster=w677, "big-maq"=w676) -> (w678:T23)
        n249 = call <vilib>:"Add State(s) to Queue__jki_lib_state_machine.vi"("State(s) in (\"\")"=w682) -> ("States Out"=w681:string)  [unwired: 14 in]
      }
      frame "UI: Update Control" {
        n250 = call <vilib>:"Parse State Queue__jki_lib_state_machine.vi"("State Queue"=w685, "Error In (no error)"=w687) -> ("Current State"=w686:string, "Arguments"=w684:string)  [unwired: 11 in, 1 out]
        n251 = case shown="\"Image Data Range\"" w686 {
          tunnel: w693 -> [w698 w701 w705 w709 w716 w724 w728 w730 w735 w737 w743]
          tunnel: [w698 w701 w705 w709 w716 w724 w728 w730 w735 w737 w743] -> w692
          tunnel: w690 -> [w697 w703 w707 w711 w715 w723 w727 w732 w733 w740 w745]
          tunnel: [w697 w703 w707 w711 w715 w723 w727 w732 w733 w740 w745] -> w691
          tunnel: w687 -> [w696 w702 w706 w710 w714 w722 w726 w731 w736 w739 w744]
          tunnel: [w696 w702 w706 w710 w714 w722 w726 w731 w736 w739 w744] -> w689
          tunnel: w684 -> [_ _ _ _ w712 w719 w725 _ _ _ _]
          tunnel: ["" "Image Data Range Updated via Program" _ _ "" _ _ _ _ _ "Page Control Updated via Program"] -> w683
          frame Default {
          }
          frame "Image Data Range" {
            n252 = Unbundle By Name(w701) -> ("UI.Image Data Range"=w700:cluster{sgl, sgl})
            n253 = local write "Image Data Range"(w700) -> ()
          }
          frame "Autosave Path" {
            n254 = Unbundle By Name(w705) -> ("UI.Autosave Path"=w704:path)
            n255 = local write "Autosave Path"(w704) -> ()
          }
          frame "Autosave" {
            n256 = Unbundle By Name(w709) -> ("UI.Autosave?"=w708:bool)
            n257 = local write "Autosave?"(w708) -> ()
          }
          frame "Estimated Time" {
            n258 = local write "Estimated Time"(w712) -> ()
          }
          frame "Ready" {
            n259 = To Upper Case(1:w719) -> (0:w717:string)
            n260 = Match True/False String(2:"FALSE" ("false string"), 3:"TRUE" ("true string"), 4:w717) -> (0:w718:bool)  [unwired: 1 out]
            n261 = local write "Ready?"(w718) -> ()
          }
          frame "Image Filename" {
            n262 = local write "Image Filename"(w725) -> ()
          }
          frame "Background Image" {
            n263 = Unbundle By Name(w730) -> ("UI.Background Image"=w729:path)
            n264 = local write "Background Image"(w729) -> ()
          }
          frame "Inkscape" {
            n265 = Unbundle By Name(w735) -> ("UI.Inkscape File (.svg)"=w734:path)
            n266 = local write "Inkscape File (.svg)"(w734) -> ()
          }
          frame "Hide Labels" {
            n267 = Unbundle By Name(w737) -> ("UI.Hide Labels"=w738:bool)
            n268 = local write "Hide Labels?"(w738) -> ()
          }
          frame "Page" {
            n269 = Unbundle By Name(w743) -> ("UI.Page"=w742:u32)
            n270 = local write "Page"(w742) -> ()
          }
        }
        n271 = call <vilib>:"Add State(s) to Queue__jki_lib_state_machine.vi"("State(s) in (\"\")"=w691) -> ("States Out"=w694:string)  [unwired: 14 in]
      }
      frame "UI: Initialize" {
        # "Initialize the User Interface, here.\n(this is called automatically, by the Macro: Init)"
        n272 = Unbundle By Name(w759) -> ("Core.Current VI Reference"=w758:refnum<vi>)
        n273 = control-ref of="Status"() -> (w763:refnum<vi>)
        n274 = call <userlib>:"MGI Get Executable Version.vi"() -> ("Version"=w757:string)  [unwired: 7 in]
        n275 = Concatenate Strings("v" ("string"), w757, "_beta" ("string")) -> (w756:string)
        n276 = property class="Str"(reference=w763, error in=w760, "Text.FontName"="Consolas" ("Text.Font:Name"), "Text.FontSize"=u32 20 ("Text.Font:Size")) -> (error out=w751:errorcluster)  [unwired: 1 out]
        n277 = control-ref of="AFM Type"() -> (w753:refnum<vi>)
        n278 = local write "version"(w756) -> ()
        n279 = property class="Ring (strict)"(reference=w753, error in=w751, "Strings []"=string[] ["Asylum"] ("t")) -> (error out=w750:errorcluster)  [unwired: 1 out]
        n280 = local write "Image Data Range"(cluster{sgl, sgl} {100.0, 0.0} ("Image Data Range")) -> ()
        n281 = call <userlib>:"Fit VI window to Largest Dec__ogtk.vi"("error in (no error)"=w750, "VI Ref (calling VI)"=w758) -> ("error out"=w747:errorcluster)  [unwired: 4 in, 1 out]
        n282 = flat-sequence {
          tunnel: w747 -> [w767]
          tunnel: [w767] -> w746
          frame #0 {
            n283 = local write "Abort"(FALSE ("Abort")) -> ()
            n284 = local write "Help"(FALSE ("Help")) -> ()
            n285 = local write "Done"(FALSE ("Done")) -> ()
            n286 = local write "Refresh Button"(FALSE ("Refresh Button")) -> ()
            n287 = local write "Run"(FALSE ("Run")) -> ()
          }
        }
        n288 = call <vilib>:"Add State(s) to Queue__jki_lib_state_machine.vi"("State(s) in (\"\")"=w766) -> ("States Out"=w765:string)  [unwired: 14 in]
      }
      frame "UI: Cursor Set" {
        # "Argument"
        # "Set and Unset Cursor Busy.\n(Usage: \"UI: Cursor Set >> Busy|Idle\")"
        n289 = case shown="\"Idle\", Default" w774 {
          tunnel: w776 -> [w781 w783]
          tunnel: [w780 w782] -> w775
          frame "Idle", Default {
            n290 = call <vilib>:"Unset Busy.vi"("error in (no error)"=w781) -> ("error out"=w780:errorcluster)  [unwired: 10 in]
          }
          frame "Busy" {
            n291 = call <vilib>:"Set Busy.vi"("error in (no error)"=w783) -> ("error out"=w782:errorcluster)  [unwired: 9 in, 1 out]
          }
        }
        n292 = call <vilib>:"Add State(s) to Queue__jki_lib_state_machine.vi"("State(s) in (\"\")"=w779) -> ("States Out"=w778:string)  [unwired: 14 in]
      }
      frame "UI: Front Panel State" {
        # "Argument"
        # "Set Front Panel Open or Closed\n(Usage: \"UI: Front Panel State >> Open|Close\")"
        n293 = Unbundle By Name(w787) -> ("Core.Current VI Reference"=w786:refnum<vi>)
        n294 = case shown="\"Open\", \"Standard\", Default" w785 {
          tunnel: w789 -> [w797 w812 w823 w836 w849]
          tunnel: [w799 w813 w825 w838 w851] -> w788
          tunnel: w786 -> [w798 w810 w824 w837 w850]
          frame "Open", "Standard", Default {
            w792 = T6."Standard" ("State")
            n295 = property class="VI"(reference=w798, error in=w797) -> (reference out=w795:refnum<vi>, error out=w796:errorcluster, "FP.State"=w794:T6)
            n296 = Not Equal?(x=w794, y=w792) -> (x != y?=w793:bool)
            n297 = case shown="False" w793 {
              tunnel: [w803 w805] -> w799
              tunnel: w796 -> [w802 w805]
              tunnel: w795 -> [w801 _]
              tunnel: w792 -> [w800 _]
              frame True {
                n298 = invoke class="VI" method="FP.Open"(reference=w801, error in=w802, "Activate"=TRUE, "State"=w800) -> (error out=w803:errorcluster)  [unwired: 1 in, 4 out]
              }
              frame False {
              }
            }
          }
          frame "Close", "Closed" {
            n299 = property class="VI"(reference=w810, error in=w812) -> (reference out=w809:refnum<vi>, error out=w811:errorcluster, "FP.State"=w807:T6)
            n300 = Not Equal?(x=w807, y=T6."Closed" ("Front Panel Window:State")) -> (x != y?=w806:bool)
            n301 = case shown="True" w806 {
              tunnel: [w814 w817] -> w813
              tunnel: w811 -> [w814 w816]
              tunnel: w809 -> [_ w815]
              frame False {
              }
              frame True {
                n302 = invoke class="VI" method="FP.Close"(reference=w815, error in=w816) -> (error out=w817:errorcluster)  [unwired: 1 in, 2 out]
              }
            }
          }
          frame "Hidden", "Hide" {
            w818 = T6."Hidden" ("State")
            n303 = property class="VI"(reference=w824, error in=w823) -> (reference out=w821:refnum<vi>, error out=w822:errorcluster, "FP.State"=w820:T6)
            n304 = Not Equal?(x=w820, y=w818) -> (x != y?=w819:bool)
            n305 = case shown="True" w819 {
              tunnel: [w829 w830] -> w825
              tunnel: w822 -> [w828 w830]
              tunnel: w821 -> [w827 _]
              tunnel: w818 -> [w826 _]
              frame True {
                n306 = invoke class="VI" method="FP.Open"(reference=w827, error in=w828, "State"=w826) -> (error out=w829:errorcluster)  [unwired: 2 in, 4 out]
              }
              frame False {
              }
            }
          }
          frame "Minimize", "Minimized" {
            w831 = T6."Minimized" ("State")
            n307 = property class="VI"(reference=w837, error in=w836) -> (reference out=w834:refnum<vi>, error out=w835:errorcluster, "FP.State"=w833:T6)
            n308 = Not Equal?(x=w833, y=w831) -> (x != y?=w832:bool)
            n309 = case shown="True" w832 {
              tunnel: [w842 w843] -> w838
              tunnel: w835 -> [w841 w843]
              tunnel: w834 -> [w840 _]
              tunnel: w831 -> [w839 _]
              frame True {
                n310 = invoke class="VI" method="FP.Open"(reference=w840, error in=w841, "State"=w839) -> (error out=w842:errorcluster)  [unwired: 2 in, 4 out]
              }
              frame False {
              }
            }
          }
          frame "Maximize", "Maximized" {
            w844 = T6."Maximized" ("State")
            n311 = property class="VI"(reference=w850, error in=w849) -> (reference out=w847:refnum<vi>, error out=w848:errorcluster, "FP.State"=w846:T6)
            n312 = Not Equal?(x=w846, y=w844) -> (x != y?=w845:bool)
            n313 = case shown="True" w845 {
              tunnel: [w855 w856] -> w851
              tunnel: w848 -> [w854 w856]
              tunnel: w847 -> [w853 _]
              tunnel: w844 -> [w852 _]
              frame True {
                n314 = invoke class="VI" method="FP.Open"(reference=w853, error in=w854, "State"=w852) -> (error out=w855:errorcluster)  [unwired: 2 in, 4 out]
              }
              frame False {
              }
            }
          }
        }
        n315 = call <vilib>:"Add State(s) to Queue__jki_lib_state_machine.vi"("State(s) in (\"\")"=w791) -> ("States Out"=w790:string)  [unwired: 14 in]
      }
      frame "---------- Macro ----------" {
        # "Do not put any code in this frame.\n(It is a separator no-op. You can make a copy of this frame to create a new Macro frame)"
        n316 = call <vilib>:"Add State(s) to Queue__jki_lib_state_machine.vi"("State(s) in (\"\")"=w861) -> ("States Out"=w860:string)  [unwired: 14 in]
      }
      frame "Macro: Start SMOs" {
        # "Do not put any code in this frame.\n(It is a separator no-op. You can make a copy of this frame to create a new Macro frame)"
        n317 = call <vilib>:"Add State(s) to Queue__jki_lib_state_machine.vi"("State(s) in Front (\"\")"="Tool: Start\nSettings: Start\nSubpanel: Initialize //This also has SMOs in it for the subpanels\nParse: Start", "State(s) in (\"\")"=w867) -> ("States Out"=w866:string)  [unwired: 13 in]
      }
      frame "Macro: Start Subsystems" {
        # "Do not put any code in this frame.\n(It is a separator no-op. You can make a copy of this frame to create a new Macro frame)"
        n318 = call <vilib>:"Add State(s) to Queue__jki_lib_state_machine.vi"("State(s) in Front (\"\")"="Select: Create\nBig MAQ: Initialize", "State(s) in (\"\")"=w873) -> ("States Out"=w872:string)  [unwired: 13 in]
      }
      frame "Macro: Initialize UI" {
        # "Do not put any code in this frame.\n(It is a separator no-op. You can make a copy of this frame to create a new Macro frame)"
        n319 = call <vilib>:"Add State(s) to Queue__jki_lib_state_machine.vi"("State(s) in Front (\"\")"="UI: Initialize\nUI: Enable Run >> Enabled\nUI: Big MAQ Initialize\nUI: Select Initialize\nUI: Update Control >> Hide Labels\nUI: Front Panel State >> Open", "State(s) in (\"\")"=w879) -> ("States Out"=w878:string)  [unwired: 13 in]
      }
      frame "Macro: Objects Updated" {
        # "Do not put any code in this frame.\n(It is a separator no-op. You can make a copy of this frame to create a new Macro frame)"
        n320 = call <vilib>:"Add State(s) to Queue__jki_lib_state_machine.vi"("State(s) in Front (\"\")"="UI: Update Control >> Ready >> False\nSelect: Apply Symbols\nSelect: Update\nTool: Objects" ("State(s) in Front (\"\")"), "State(s) in (\"\")"=w885) -> ("States Out"=w884:string)  [unwired: 13 in]
      }
      frame "Macro: Initialize" {
        # "Initialization Macro\n(This is called once, when the VI starts)"
        n321 = call <vilib>:"Add State(s) to Queue__jki_lib_state_machine.vi"("State(s) in Front (\"\")"="Data: Initialize\nInitialize Core Data\nData: Status //needs to be initialized really early\nLog: Start\nUI: Update Control >> Ready >> False\nFile: Get Root Path\nConfig: Initialize\nConfig: Read\nUI: Update Control >> Autosave Path\nUI: Update Control >> Autosave\n//File: Get Control Values\nAFM: Initialize Manager\nAFM: Initialize Driver\nAFM: Set Active >> 0\nAFM: Insert Into Subpanel\nMacro: Start SMOs\nEvents: Register\nMacro: Start Subsystems\nMacro: Initialize UI\nFile: Inkscape\nFile: Background\nAFM: Background Image\nBig MAQ: Read Background\nBig MAQ: Update\nBig MAQ: Zoom Fit\nBig MAQ: Save Background\nUI: Update Zoom Factor\nParse: Send File // this event will kick everything else off", "State(s) in (\"\")"=w891) -> ("States Out"=w890:string)  [unwired: 13 in]
      }
      frame "Macro: Exit" {
        # "Exit Macro\n(This is called once, when the VI exits)"
        n322 = Unbundle By Name(w899) -> ("Core.Close Panel on Exit?"=w898:bool)
        n323 = Select(t="UI: Front Panel State >> Close", s=w898, f="") -> (s? t:f=w895:string)
        n324 = call <vilib>:"Add State(s) to Queue__jki_lib_state_machine.vi"("State(s) in (\"\")"=w895, "State(s) at Back (\"\")"="Config: Write\nAFM: Stop Manager\nParse: Stop\nSubpanel: Close\nSettings: Stop\nTool: Stop\nBig MAQ: Cleanup\nIdentity: Destroy Registry\nLog: Stop\nData: Cleanup\nEvents: Unregister\nExit") -> ("States Out"=w893:string)  [unwired: 13 in]
        n325 = call <vilib>:"Add State(s) to Queue__jki_lib_state_machine.vi"("State(s) in Front (\"\")"=w893, "State(s) in (\"\")"=w902) -> ("States Out"=w901:string)  [unwired: 13 in]
      }
      frame "---------- File ----------" {
        # "Do not put any code in this frame.\n(It is a separator no-op. You can make a copy of this frame to create a new UI frame)"
        n326 = call <vilib>:"Add State(s) to Queue__jki_lib_state_machine.vi"("State(s) in (\"\")"=w907) -> ("States Out"=w906:string)  [unwired: 14 in]
      }
      frame "File: Get Control Values" {
        # "Do not put any code in this frame.\n(It is a separator no-op. You can make a copy of this frame to create a new UI frame)"
        n327 = local read "Background Image"() -> (w910:path)
        n328 = local read "Inkscape File (.svg)"() -> (w908:path)
        n329 = local read "Autosave Path"() -> (w909:path)
        n330 = Bundle By Name(cluster=w911, "UI.Inkscape File (.svg)"=w908, "UI.Background Image"=w910, "UI.Autosave Path"=w909) -> (w912:T23)
        n331 = call <vilib>:"Add State(s) to Queue__jki_lib_state_machine.vi"("State(s) in (\"\")"=w916) -> ("States Out"=w915:string)  [unwired: 14 in]
      }
      frame "File: Get Root Path" {
        # "Do not put any code in this frame.\n(It is a separator no-op. You can make a copy of this frame to create a new UI frame)"
        n332 = call <userlib>:"Current VI's Path__ogtk.vi"() -> ("Current VI's Path (+ Relative)"=w920:path)  [unwired: 1 in]
        n333 = Strip Path(path=w920) -> (stripped path=w919:path)  [unwired: 1 out]
        n334 = Bundle By Name(cluster=w917, "root path"=w919) -> (w918:T23)
        n335 = call <vilib>:"Add State(s) to Queue__jki_lib_state_machine.vi"("State(s) in (\"\")"=w924) -> ("States Out"=w923:string)  [unwired: 14 in]
      }
      frame "File: Autosave Path" {
        # "Do not put any code in this frame.\n(It is a separator no-op. You can make a copy of this frame to create a new UI frame)"
        n336 = call <vilib>:"Add State(s) to Queue__jki_lib_state_machine.vi"("State(s) in (\"\")"=w929) -> ("States Out"=w928:string)  [unwired: 14 in]
      }
      frame "File: Inkscape" {
        # "Do not put any code in this frame.\n(It is a separator no-op. You can make a copy of this frame to create a new UI frame)"
        n337 = Unbundle By Name(w933) -> ("UI.Inkscape File (.svg)"=w945:path)
        n338 = call "CheckFileConformity.vi"("error in (no error)"=w938, "File Data"=T10 {"Pattern"="svg", "Pattern Label"="Scalable Vector Graphics", "Prompt"="Choose an SVG file"}, "Path In"=w945) -> ("error out"=w943:errorcluster, "No File"=w940:bool, "Path Out"=w944:path, "Asked to Change?"=w937:bool)  [unwired: 5 in]
        n339 = case shown="False" w940 {
          tunnel: w944 -> [w950 _]
          tunnel: w943 -> [w949 w953]
          tunnel: [w949 w955] -> w939
          tunnel: [w950 w954] -> w942
          frame False {
          }
          frame True {
            n340 = call "Display Message to User2"("error in (no error)"=w953, "Message"="No Valid File Selected. Using Default.") -> ("error out"=w952:errorcluster)  [unwired: 8 in, 1 out]
            n341 = call "GenerateDefaultSVGFile.vi"("error in (no error)"=w952) -> ("error out"=w955:errorcluster, "Path"=w954:path)  [unwired: 9 in]
          }
        }
        n342 = Select(t="", s=w937, f="Config: Write") -> (s? t:f=w931:string)
        n343 = Bundle By Name(cluster=w933, "UI.Inkscape File (.svg)"=w942) -> (w934:T23)
        n344 = call <vilib>:"Add State(s) to Queue__jki_lib_state_machine.vi"("State(s) in Front (\"\")"=w931, "State(s) in (\"\")"="UI: Update Control >> Inkscape" ("State(s) at Back (\"\")")) -> ("States Out"=w930:string)  [unwired: 13 in]
        n345 = call <vilib>:"Add State(s) to Queue__jki_lib_state_machine.vi"("State(s) in Front (\"\")"=w930, "State(s) in (\"\")"=w948) -> ("States Out"=w947:string)  [unwired: 13 in]
      }
      frame "File: Background" {
        # "Do not put any code in this frame.\n(It is a separator no-op. You can make a copy of this frame to create a new UI frame)"
        n346 = Unbundle By Name(w970) -> ("UI.Background Image"=w976:path)
        n347 = call "CheckFileConformity.vi"("error in (no error)"=w969, "File Data"=T10 {"Pattern"="ibw", "Pattern Label"="Igor Binary Wave", "Prompt"="Choose an IBW file"}, "Path In"=w976) -> ("error out"=w973:errorcluster, "No File"=w972:bool, "Path Out"=w974:path, "Asked to Change?"=w968:bool)  [unwired: 5 in]
        n348 = case shown="True" w972 {
          tunnel: w973 -> [w980 w983]
          tunnel: w974 -> [w981 _]
          tunnel: [w981 w985] -> w965
          tunnel: [w980 w986] -> w963
          frame False {
          }
          frame True {
            n349 = call "Display Message to User"("error in (no error)"=w983, "Message"="No Valid File Selected. Using Default.") -> ("error out"=w982:errorcluster)  [unwired: 8 in, 1 out]
            n350 = call "GenerateDefaultIBWFile.vi"("error in (no error)"=w982) -> ("error out"=w986:errorcluster, "Path"=w985:path)  [unwired: 9 in]
          }
        }
        n351 = Select(t="", s=w968, f="Config: Write") -> (s? t:f=w958:string)
        n352 = call <vilib>:"Get File Extension.vi"("error in (no error)"=w963, "file"=w965) -> ("error out"=w962:errorcluster, "filename without extension"=w961:string, "dup file"=w964:path)  [unwired: 5 in, 2 out]
        n353 = call <vilib>:"Build State String with Arguments__JKI_lib_State_Machine.vi"("Arguments (\"\")"=w961, "State"="UI: Update Control >> Image Filename") -> ("State with Arguments"=w956:string)  [unwired: 4 in]
        n354 = Bundle By Name(cluster=w970, "UI.Background Image"=w964) -> (w971:T23)
        n355 = call <vilib>:"Add State(s) to Queue__jki_lib_state_machine.vi"("State(s) in Front (\"\")"=w958, "State(s) in (\"\")"="UI: Update Control >> Background Image" ("State(s) at Back (\"\")"), "State(s) at Back (\"\")"=w956) -> ("States Out"=w960:string)  [unwired: 12 in]
        n356 = call <vilib>:"Add State(s) to Queue__jki_lib_state_machine.vi"("State(s) in Front (\"\")"=w960, "State(s) in (\"\")"=w979) -> ("States Out"=w978:string)  [unwired: 13 in]
      }
      frame "---------- Identity ----------" {
        # "Do not put any code in this frame.\n(It is a separator no-op. You can make a copy of this frame to create a new UI frame)"
        n357 = call <vilib>:"Add State(s) to Queue__jki_lib_state_machine.vi"("State(s) in (\"\")"=w991) -> ("States Out"=w990:string)  [unwired: 14 in]
      }
      frame "Identity: Destroy Registry" {
        # "Do not put any code in this frame.\n(It is a separator no-op. You can make a copy of this frame to create a new UI frame)"
        n358 = call "Destroy Registry.vi"("error in"=w993) -> ("error out"=w994:errorcluster)  [unwired: 10 in]
        n359 = call <vilib>:"Add State(s) to Queue__jki_lib_state_machine.vi"("State(s) in (\"\")"=w998) -> ("States Out"=w997:string)  [unwired: 14 in]
      }
      frame "Identity: Populate" {
        # "Do not put any code in this frame.\n(It is a separator no-op. You can make a copy of this frame to create a new UI frame)"
        n360 = Unbundle By Name(w1007) -> ("GUIDs.Dots"=w1004:string[], "GUIDs.Funnels"=w1003:string[], "GUIDs.Rects"=w1002:string[], "GUIDs.Paths"=w1005:string[])
        n361 = Bundle By Name(cluster=T11 {"paths"=[], "funnels"=[], "rects"=[], "dots"=[]} ("IDs"), "dots"=w1004, "funnels"=w1003, "rects"=w1002, "paths"=w1005) -> (w1001:T11)
        n362 = call "IDs to Names.vi"("IDs"=w1001) -> ("Names"=w1008:string[], "IDs"=w1000:string[])  [unwired: 9 in]
        n363 = call "Populate Registry.vi"("error in"=w1009, "Aliases"=w1008, "Names"=w1000) -> ("error out"=w1010:errorcluster)  [unwired: 8 in]
        n364 = call <vilib>:"Add State(s) to Queue__jki_lib_state_machine.vi"("State(s) in (\"\")"=w1013) -> ("States Out"=w1012:string)  [unwired: 14 in]
      }
      frame "---------- Parse ----------" {
        # "Parse: \n(Template Separater for Parsing. You can make a copy of, or modify, this frame)"
        n365 = Unbundle By Name(w1016) -> ("parser"=w1015:refnum<class "ParseVectorFile.lvclass">)
        n366 = Bundle By Name(cluster=w1016, "parser"=w1015) -> (w1017:T23)
        n367 = call <vilib>:"Add State(s) to Queue__jki_lib_state_machine.vi"("State(s) in (\"\")"=w1020) -> ("States Out"=w1019:string)  [unwired: 14 in]
      }
      frame "Parse: Send File" {
        # "Parse: \n(Template Separater for Parsing. You can make a copy of, or modify, this frame)"
        n368 = Unbundle By Name(w1028) -> ("parser"=w1026:refnum<class "ParseVectorFile.lvclass">, "UI.Inkscape File (.svg)"=w1024:path)
        n369 = call "ParseVectorFile.NewFileAsynchronous.vi"("error in (no error)"=w1022, "NewFile"=w1024, "ParseVectorFile"=w1026) -> ("error out"=w1023:errorcluster, "ParseVectorFile out"=w1025:refnum<class "ParseVectorFile.lvclass">)  [unwired: 7 in]
        n370 = Bundle By Name(cluster=w1028, "parser"=w1025) -> (w1029:T23)
        n371 = call <vilib>:"Add State(s) to Queue__jki_lib_state_machine.vi"("State(s) in (\"\")"=w1031) -> ("States Out"=w1030:string)  [unwired: 14 in]
      }
      frame "Parse: Stop" {
        # "Parse: \n(Template Separater for Parsing. You can make a copy of, or modify, this frame)"
        n372 = Unbundle By Name(w1040) -> ("parser"=w1035:refnum<class "ParseVectorFile.lvclass">)
        n373 = call <vilib>:"Stop.vi"("error in (no error)"=w1033, "SMO"=w1035) -> ("error out"=w1038:errorcluster, "SMO out"=w1037:refnum<class "ParseVectorFile.lvclass">)  [unwired: 8 in]
        n374 = call <vilib>:"Destroy.vi"("error in (no error)"=w1038, "SMO"=w1037) -> ("error out"=w1034:errorcluster)  [unwired: 9 in]
        n375 = Bundle By Name(cluster=w1040, "parser"=refnum<class "ParseVectorFile.lvclass"> refnum) -> (w1041:T23)
        n376 = call <vilib>:"Add State(s) to Queue__jki_lib_state_machine.vi"("State(s) in (\"\")"=w1043) -> ("States Out"=w1042:string)  [unwired: 14 in]
      }
      frame "Parse: Start" {
        # "Parse: \n(Template Separater for Parsing. You can make a copy of, or modify, this frame)"
        n377 = Unbundle By Name(w1052) -> ("parser"=w1048:refnum<class "ParseVectorFile.lvclass">)
        n378 = call <vilib>:"Create.vi"("error in (no error)"=w1045, "SMO"=w1048) -> ("error out"=w1049:errorcluster, "SMO out"=w1050:refnum<class "ParseVectorFile.lvclass">)  [unwired: 7 in, 1 out]
        n379 = call <vilib>:"Start.vi"("error in (no error)"=w1049, "SMO"=w1050) -> ("error out"=w1046:errorcluster, "SMO out"=w1047:refnum<class "ParseVectorFile.lvclass">)  [unwired: 8 in]
        n380 = Bundle By Name(cluster=w1052, "parser"=w1047) -> (w1053:T23)
        n381 = call <vilib>:"Add State(s) to Queue__jki_lib_state_machine.vi"("State(s) in (\"\")"=w1055) -> ("States Out"=w1054:string)  [unwired: 14 in]
      }
      frame "---------- Settings ----------" {
        # "Settings: \n(Template Separater for Settings. You can make a copy of, or modify, this frame)"
        n382 = Unbundle By Name(w1058) -> ("settings"=w1057:refnum<class "Setting Database.lvclass">)
        n383 = Bundle By Name(cluster=w1058, "settings"=w1057) -> (w1059:T23)
        n384 = call <vilib>:"Add State(s) to Queue__jki_lib_state_machine.vi"("State(s) in (\"\")"=w1062) -> ("States Out"=w1061:string)  [unwired: 14 in]
      }
      frame "Settings: Set Active" {
        # "Settings: \n(Template Separater for Settings. You can make a copy of, or modify, this frame)"
        n385 = call "Name To Type.vi"("Name"=w1064) -> ("Type"=w1070:string)  [unwired: 4 in]
        n386 = call "Name To Index.vi"("Name"=w1064) -> ("Index"=w1069:i32)  [unwired: 4 in]
        n387 = Unbundle By Name(w1072) -> ("settings"=w1068:refnum<class "Setting Database.lvclass">)
        n388 = case shown="Default" w1070 {
          tunnel: w1068 -> [w1080 w1082 w1087 w1092 w1097 w1101]
          tunnel: [w1079 w1081 w1086 w1090 w1095 w1100] -> w1066
          tunnel: w1065 -> [w1076 w1081 w1085 w1089 w1094 w1099]
          tunnel: [w1080 w1082 w1084 w1091 w1096 w1102] -> w1067
          tunnel: w1069 -> [_ _ w1083 w1088 w1093 w1098]
          frame Default {
            n389 = call <vilib>:"Error Cluster From Error Code.vi"("error in (no error)"=w1076, "error message (\"\")"="Unknown Object Type. Cannot Set Active In Database" ("error message (\"\")"), "error code (0)"=1) -> ("error out"=w1079:errorcluster)  [unwired: 6 in]
          }
          frame "" {
            # "There are no objects to set as active\n\nTemp fix for issue \\#78:\nhttps://github.com/levylabpitt/AFM-Lithography/issues/78"
          }
          frame "p" {
            n390 = call "Setting Database.SetActivePath.vi"("error in (no error)"=w1085, "SetActivePath"=w1083, "Setting Database"=w1087) -> ("error out"=w1086:errorcluster, "Setting Database out"=w1084:refnum<class "Setting Database.lvclass">)  [unwired: 7 in]
          }
          frame "r" {
            n391 = call "Setting Database.SetActiveRectangle.vi"("error in (no error)"=w1089, "SetActiveRectangle"=w1088, "Setting Database"=w1092) -> ("error out"=w1090:errorcluster, "Setting Database out"=w1091:refnum<class "Setting Database.lvclass">)  [unwired: 7 in]
          }
          frame "f" {
            n392 = call "Setting Database.SetActiveFunnel.vi"("error in (no error)"=w1094, "SetActiveFunnel"=w1093, "Setting Database"=w1097) -> ("error out"=w1095:errorcluster, "Setting Database out"=w1096:refnum<class "Setting Database.lvclass">)  [unwired: 7 in]
          }
          frame "d" {
            # "Need to send the data event here"
            n393 = call "Setting Database.SetActiveDot.vi"("error in (no error)"=w1099, "SetActiveDot"=w1098, "Setting Database"=w1101) -> ("error out"=w1100:errorcluster, "Setting Database out"=w1102:refnum<class "Setting Database.lvclass">)  [unwired: 7 in]
          }
        }
        n394 = Bundle By Name(cluster=w1072, "settings"=w1067) -> (w1073:T23)
        n395 = call <vilib>:"Add State(s) to Queue__jki_lib_state_machine.vi"("State(s) in (\"\")"=w1075) -> ("States Out"=w1074:string)  [unwired: 14 in]
      }
      frame "Settings: Change Enable" {
        # "Settings: \n(Template Separater for Settings. You can make a copy of, or modify, this frame)"
        n396 = Unbundle By Name(w1110) -> ("settings"=w1108:refnum<class "Setting Database.lvclass">)
        n397 = call "Setting Database.ChangeObjectEnable.vi"("error in (no error)"=w1104, "ChangeObjectEnable"=w1106, "Setting Database"=w1108) -> ("error out"=w1105:errorcluster, "Setting Database out"=w1107:refnum<class "Setting Database.lvclass">)  [unwired: 7 in]
        n398 = Bundle By Name(cluster=w1110, "settings"=w1107) -> (w1111:T23)
        n399 = call <vilib>:"Add State(s) to Queue__jki_lib_state_machine.vi"("State(s) in (\"\")"=w1113) -> ("States Out"=w1112:string)  [unwired: 14 in]
      }
      frame "Settings: Group" {
        # "Settings: \n(Template Separater for Settings. You can make a copy of, or modify, this frame)"
        n400 = Unbundle By Name(w1128) -> ("settings"=w1126:refnum<class "Setting Database.lvclass">)
        n401 = Spreadsheet String To Array(delimiter (Tab)=":", format string="%s", spreadsheet string=w1123, array type (2D Dbl)=string[] []) -> (array=w1120:string[])
        n402 = Index Array(array=w1120) -> (element #1=w1117:string, element #2=w1119:string, element #3=w1118:string)  [unwired: 3 in]
        n403 = case shown="\"remove\"" w1117 {
          tunnel: w1126 -> [w1133 w1140 w1147 w1154]
          tunnel: [w1133 w1141 w1146 w1153] -> w1125
          tunnel: w1119 -> [_ w1138 w1149 w1150]
          tunnel: w1118 -> [_ w1137 w1148 _]
          tunnel: w1115 -> [w1132 w1135 w1145 w1152]
          tunnel: [w1132 w1134 w1144 w1151] -> w1116
          frame Default {
          }
          frame "add" {
            n404 = Bundle(cluster=T12 {"Name"="", "Group"=""} ("Add To Group"), "Name"=w1138, "Group"=w1137) -> (w1136:T12)
            n405 = call "Setting Database.AddToGroup.vi"("error in (no error)"=w1135, "Add To Group"=w1136, "Setting Database"=w1140) -> ("error out"=w1134:errorcluster, "Setting Database out"=w1141:refnum<class "Setting Database.lvclass">)  [unwired: 7 in]
          }
          frame "create" {
            n406 = Bundle(cluster=T13 {"Name"="", "Group"=""} ("Create New Group"), "Name"=w1149, "Group"=w1148) -> (w1142:T13)
            n407 = call "Setting Database.CreateNewGroup.vi"("error in (no error)"=w1145, "Create New Group"=w1142, "Setting Database"=w1147) -> ("error out"=w1144:errorcluster, "Setting Database out"=w1146:refnum<class "Setting Database.lvclass">)  [unwired: 7 in]
          }
          frame "remove" {
            n408 = call "Setting Database.RemoveFromGroup.vi"("error in (no error)"=w1152, "Remove From Group"=w1150, "Setting Database"=w1154) -> ("error out"=w1151:errorcluster, "Setting Database out"=w1153:refnum<class "Setting Database.lvclass">)  [unwired: 7 in]
          }
        }
        n409 = Bundle By Name(cluster=w1128, "settings"=w1125) -> (w1129:T23)
        n410 = call <vilib>:"Add State(s) to Queue__jki_lib_state_machine.vi"("State(s) in (\"\")"=w1131) -> ("States Out"=w1130:string)  [unwired: 14 in]
      }
      frame "Settings: Refresh" {
        # "Settings: \n(Template Separater for Settings. You can make a copy of, or modify, this frame)"
        n411 = Unbundle By Name(w1167) -> ("settings"=w1165:refnum<class "Setting Database.lvclass">, "GUIDs.Paths"=w1163:string[], "GUIDs.Rects"=w1161:string[], "GUIDs.Funnels"=w1160:string[], "GUIDs.Dots"=w1159:string[])
        n412 = Bundle By Name(cluster=T14 {"Paths"=[], "Rectangles"=[], "Funnels"=[], "Dots"=[]} ("Initialize"), "Paths"=w1163, "Rectangles"=w1161, "Funnels"=w1160, "Dots"=w1159) -> (w1158:T14)
        n413 = call "Setting Database.Refresh.vi"("error in (no error)"=w1157, "Initialize"=w1158, "Setting Database"=w1165) -> ("error out"=w1156:errorcluster, "Setting Database out"=w1164:refnum<class "Setting Database.lvclass">)  [unwired: 7 in]
        n414 = Bundle By Name(cluster=w1167, "settings"=w1164) -> (w1168:T23)
        n415 = call <vilib>:"Add State(s) to Queue__jki_lib_state_machine.vi"("State(s) in (\"\")"=w1170) -> ("States Out"=w1169:string)  [unwired: 14 in]
      }
      frame "Settings: Stop" {
        # "Settings: \n(Template Separater for Settings. You can make a copy of, or modify, this frame)"
        n416 = Unbundle By Name(w1179) -> ("settings"=w1176:refnum<class "Setting Database.lvclass">)
        n417 = call <vilib>:"Stop.vi"("error in (no error)"=w1173, "SMO"=w1176) -> ("error out"=w1177:errorcluster, "SMO out"=w1175:refnum<class "Setting Database.lvclass">)  [unwired: 8 in]
        n418 = call <vilib>:"Destroy.vi"("error in (no error)"=w1177, "SMO"=w1175) -> ("error out"=w1172:errorcluster)  [unwired: 9 in]
        n419 = Bundle By Name(cluster=w1179, "settings"=refnum<class "Setting Database.lvclass"> refnum) -> (w1180:T23)
        n420 = call <vilib>:"Add State(s) to Queue__jki_lib_state_machine.vi"("State(s) in (\"\")"=w1182) -> ("States Out"=w1181:string)  [unwired: 14 in]
      }
      frame "Settings: Start" {
        # "Settings: \n(Template Separater for Settings. You can make a copy of, or modify, this frame)"
        n421 = Unbundle By Name(w1194) -> ("settings"=w1189:refnum<class "Setting Database.lvclass">)
        n422 = call "Setting Database Name.vi"("error in (no error)"=w1185) -> ("error out"=w1186:errorcluster, "Name"=w1184:string)  [unwired: 9 in]
        n423 = call <vilib>:"Create.vi"("Shared Resource (F)"=TRUE, "error in (no error)"=w1186, "Subsystem Name (optional)"=w1184, "SMO"=w1189) -> ("error out"=w1191:errorcluster, "SMO out"=w1192:refnum<class "Setting Database.lvclass">)  [unwired: 5 in, 1 out]
        n424 = call <vilib>:"Start.vi"("error in (no error)"=w1191, "SMO"=w1192) -> ("error out"=w1188:errorcluster, "SMO out"=w1190:refnum<class "Setting Database.lvclass">)  [unwired: 8 in]
        n425 = Bundle By Name(cluster=w1194, "settings"=w1190) -> (w1195:T23)
        n426 = call <vilib>:"Add State(s) to Queue__jki_lib_state_machine.vi"("State(s) in (\"\")"=w1197) -> ("States Out"=w1196:string)  [unwired: 14 in]
      }
      frame "---------- Tool ----------" {
        # "Tool: \n(Template Separater for Tooling. You can make a copy of, or modify, this frame)"
        n427 = Unbundle By Name(w1200) -> ("tooler"=w1199:refnum<class "Tool Data.lvclass">)
        n428 = Bundle By Name(cluster=w1200, "tooler"=w1199) -> (w1201:T23)
        n429 = call <vilib>:"Add State(s) to Queue__jki_lib_state_machine.vi"("State(s) in (\"\")"=w1204) -> ("States Out"=w1203:string)  [unwired: 14 in]
      }
      frame "Tool: Sort Paths" {
        # "Tool: \n(Template Separater for Tooling. You can make a copy of, or modify, this frame)"
        n430 = Unbundle By Name(w1219) -> ("Parsed Obj.Paths"=w1210:refnum<class "Path.lvclass">[])
        n431 = call-dynamic "Write Paths Data.vi"("error in (no error)"=w1206, "Paths"=w1210, "Tool Data in"=refnum<class "Tool Data.lvclass"> refnum) -> ("error out"=w1215:errorcluster, "Tool Data out"=w1212:refnum<class "Tool Data.lvclass">)  [unwired: 7 in]
        n432 = call "Sort Funnels and Paths.vi"("error in (no error)"=w1215, "Tool Data in"=w1212) -> ("error out"=w1216:errorcluster, "Tool Data out"=w1213:refnum<class "Tool Data.lvclass">)  [unwired: 8 in]
        n433 = call-dynamic "Read Paths Data.vi"("error in (no error)"=w1216, "Tool Data in"=w1213) -> ("error out"=w1217:errorcluster, "Paths"=w1209:refnum<class "Path.lvclass">[], "Tool Data out"=w1214:refnum<class "Tool Data.lvclass">)  [unwired: 7 in]
        n434 = call-dynamic "Read Funnels Data.vi"("error in (no error)"=w1217, "Tool Data in"=w1214) -> ("error out"=w1207:errorcluster, "Funnels"=w1208:refnum<class "Path.lvclass">[])  [unwired: 7 in, 1 out]
        n435 = Bundle By Name(cluster=w1219, "Parsed Obj.Paths"=w1209, "Parsed Obj.Funnels"=w1208) -> (w1220:T23)
        n436 = call <vilib>:"Add State(s) to Queue__jki_lib_state_machine.vi"("State(s) in (\"\")"=w1222) -> ("States Out"=w1221:string)  [unwired: 14 in]
      }
      frame "Tool: Get IDs" {
        # "Tool: \n(Template Separater for Tooling. You can make a copy of, or modify, this frame)"
        n437 = Unbundle By Name(w1236) -> ("Parsed Obj.Paths"=w1227:refnum<class "Path.lvclass">[], "Parsed Obj.Rectangles"=w1223:refnum<class "Rectangle.lvclass">[], "Parsed Obj.Background"=w1224:refnum<class "SVGImage.lvclass">, "Parsed Obj.Dots"=w1225:refnum<class "Dot.lvclass">[], "Parsed Obj.Funnels"=w1226:refnum<class "Path.lvclass">[])
        n438 = Bundle By Name(cluster=T15 {"Paths"=[], "Rectangles"=[], "SVGImage"=refnum, "Dots"=[], "Funnels"=[]} ("Data"), "Paths"=w1227, "Rectangles"=w1223, "SVGImage"=w1224, "Dots"=w1225, "Funnels"=w1226) -> (w1228:T15)
        n439 = property class="Tool Data.lvclass"(reference=refnum<class "Tool Data.lvclass"> refnum ("Tool Data in"), error in=w1237, "Accessors:Data"=w1228) -> (reference out=w1240:refnum<class "Tool Data.lvclass">, error out=w1238:errorcluster)
        n440 = call "Get IDs.vi"("error in (no error)"=w1238, "Tool Data in"=w1240) -> ("error out"=w1241:errorcluster, "IDs"=w1234:T11)  [unwired: 7 in, 1 out]
        n441 = Unbundle By Name(w1234) -> ("paths"=w1233:string[], "funnels"=w1232:string[], "rects"=w1231:string[], "dots"=w1230:string[])
        n442 = Bundle By Name(cluster=w1236, "GUIDs.Paths"=w1233, "GUIDs.Funnels"=w1232, "GUIDs.Rects"=w1231, "GUIDs.Dots"=w1230) -> (w1243:T23)
        n443 = call <vilib>:"Add State(s) to Queue__jki_lib_state_machine.vi"("State(s) in (\"\")"=w1245) -> ("States Out"=w1244:string)  [unwired: 14 in]
      }
      frame "Tool: Generate Litho Data" {
        # "Tool: \n(Template Separater for Tooling. You can make a copy of, or modify, this frame)"
        n444 = Unbundle By Name(w1256) -> ("tooler"=w1254:refnum<class "Tool Data.lvclass">)
        n445 = call-dynamic "Generate Lithography Data.vi"("error in (no error)"=w1251, "Tool Data in"=w1254) -> ("error out"=w1252:errorcluster, "Lithography Data"=w1247:T28, "Tool Data out"=w1253:refnum<class "Tool Data.lvclass">)  [unwired: 7 in]
        n446 = call "Estimated Time Required.vi"("Lithography Data"=w1247) -> ("Estimated Time Required"=w1249:timestamp)
        n447 = Bundle By Name(cluster=w1256, "tooler"=w1253, "Litho"=w1247) -> (w1257:T23)
        n448 = Format Date/Time String(time format string (%c)="UI: Update Control >> Estimated Time >> %H:%M:%S", seconds (now)=w1249) -> (date/time string=w1246:string)  [unwired: 1 in]
        n449 = call <vilib>:"Add State(s) to Queue__jki_lib_state_machine.vi"("State(s) in Front (\"\")"=w1246, "State(s) in (\"\")"=w1259) -> ("States Out"=w1258:string)  [unwired: 13 in]
      }
      frame "Tool: Objects" {
        # "Tool: \n(Template Separater for Tooling. You can make a copy of, or modify, this frame)"
        n450 = Unbundle By Name(w1279) -> ("tooler"=w1270:refnum<class "Tool Data.lvclass">, "Parsed Obj.Paths"=w1261:refnum<class "Path.lvclass">[], "Parsed Obj.Funnels"=w1260:refnum<class "Path.lvclass">[], "Parsed Obj.Rectangles"=w1276:refnum<class "Rectangle.lvclass">[], "Parsed Obj.Dots"=w1275:refnum<class "Dot.lvclass">[], "Obj Settings.Paths"=w1274:T17, "Obj Settings.Rectangles"=w1273:T18, "Obj Settings.Funnels"=w1272:T19, "Obj Settings.Dots"=w1271:T20)
        n451 = Bundle By Name(cluster=T16 {"Settings"={"Paths"=[], "Rectangles"=[], "Funnels"=[], "Dots"=[]}, "Data"={"Paths"=[], "Rectangles"=[], "SVGImage"=refnum, "Dots"=[], "Funnels"=[]}} ("Updated Objects"), "Data.Paths"=w1261, "Data.Funnels"=w1260, "Data.Rectangles"=w1276, "Data.Dots"=w1275, "Settings.Paths"=w1274, "Settings.Rectangles"=w1273, "Settings.Funnels"=w1272, "Settings.Dots"=w1271) -> (w1269:T16)
        n452 = call "Tool Data.UpdateObjects.vi"("error in (no error)"=w1265, "Updated Objects"=w1269, "Tool Data"=w1270) -> ("error out"=w1267:errorcluster, "Tool Data out"=w1264:refnum<class "Tool Data.lvclass">)  [unwired: 7 in]
        n453 = call-dynamic "Find Changed.vi"("error in (no error)"=w1267, "Update Objects"=w1269, "Tool Data in"=w1264) -> ("error out"=w1266:errorcluster, "Changed Objects"=w1268:T31, "Tool Data out"=w1263:refnum<class "Tool Data.lvclass">)  [unwired: 6 in]
        n454 = Bundle By Name(cluster=w1279, "tooler"=w1263, "Changed Obj"=w1268) -> (w1280:T23)
        n455 = call <vilib>:"Add State(s) to Queue__jki_lib_state_machine.vi"("State(s) in (\"\")"=w1282) -> ("States Out"=w1281:string)  [unwired: 14 in]
      }
      frame "Tool: Stop" {
        # "Tool: \n(Template Separater for Tooling. You can make a copy of, or modify, this frame)"
        n456 = Unbundle By Name(w1292) -> ("tooler"=w1288:refnum<class "Tool Data.lvclass">)
        n457 = call <vilib>:"Stop.vi"("timeout in ms (-1)"=10000, "error in (no error)"=w1286, "SMO"=w1288) -> ("error out"=w1290:errorcluster, "SMO out"=w1289:refnum<class "Tool Data.lvclass">)  [unwired: 7 in]
        n458 = call <vilib>:"Destroy.vi"("error in (no error)"=w1290, "SMO"=w1289) -> ("error out"=w1287:errorcluster)  [unwired: 9 in]
        n459 = Bundle By Name(cluster=w1292, "tooler"=refnum<class "Tool Data.lvclass"> refnum) -> (w1293:T23)
        n460 = call <vilib>:"Add State(s) to Queue__jki_lib_state_machine.vi"("State(s) in (\"\")"=w1295) -> ("States Out"=w1294:string)  [unwired: 14 in]
      }
      frame "Tool: Start" {
        # "Tool: \n(Template Separater for Tooling. You can make a copy of, or modify, this frame)"
        n461 = Unbundle By Name(w1304) -> ("tooler"=w1300:refnum<class "Tool Data.lvclass">)
        n462 = call <vilib>:"Create.vi"("error in (no error)"=w1297, "SMO"=w1300) -> ("error out"=w1301:errorcluster, "SMO out"=w1302:refnum<class "Tool Data.lvclass">)  [unwired: 7 in, 1 out]
        n463 = call <vilib>:"Start.vi"("error in (no error)"=w1301, "SMO"=w1302) -> ("error out"=w1298:errorcluster, "SMO out"=w1299:refnum<class "Tool Data.lvclass">)  [unwired: 8 in]
        n464 = Bundle By Name(cluster=w1304, "tooler"=w1299) -> (w1305:T23)
        n465 = call <vilib>:"Add State(s) to Queue__jki_lib_state_machine.vi"("State(s) in (\"\")"=w1307) -> ("States Out"=w1306:string)  [unwired: 14 in]
      }
      frame "---------- Big MAQ ----------" {
        # "Parse: \n(Template Separater for Parsing. You can make a copy of, or modify, this frame)"
        n466 = Unbundle By Name(w1310) -> ("big-maq"=w1309:refnum<class "BigMAQ.lvclass">)
        n467 = Bundle By Name(cluster=w1310, "big-maq"=w1309) -> (w1311:T23)
        n468 = call <vilib>:"Add State(s) to Queue__jki_lib_state_machine.vi"("State(s) in (\"\")"=w1314) -> ("States Out"=w1313:string)  [unwired: 14 in]
      }
      frame "Big MAQ: Coerce Size" {
        # "Parse: \n(Template Separater for Parsing. You can make a copy of, or modify, this frame)"
        n469 = Unbundle By Name(w1332) -> ("big-maq"=w1327:refnum<class "BigMAQ.lvclass">, "Parsed Obj.Background"=w1330:refnum<class "SVGImage.lvclass">)
        n470 = call "Read Height.vi"("error in (no error)"=w1324, "Image in"=w1330) -> ("error out"=w1325:errorcluster, "Height"=w1329:dbl)  [unwired: 7 in, 1 out]
        n471 = Divide(x=w1329, y=1000.0) -> (x/y=w1319:dbl)
        n472 = call-dynamic "Read Size.vi"("error in (no error)"=w1325, "BigMAQ in"=w1327) -> ("error out"=w1321:errorcluster, "Size"=w1326:dbl, "BigMAQ out"=w1323:refnum<class "BigMAQ.lvclass">)  [unwired: 7 in]
        n473 = Equal?(x=w1326, y=w1319) -> (x = y?=w1317:bool)
        n474 = case shown="False" w1317 {
          tunnel: w1323 -> [w1340 w1342]
          tunnel: [w1339 w1342] -> w1322
          tunnel: w1321 -> [w1338 w1341]
          tunnel: [w1337 w1341] -> w1320
          tunnel: w1319 -> [w1336 _]
          frame False {
            n475 = call-dynamic "Write Size.vi"("error in (no error)"=w1338, "Size"=w1336, "BigMAQ in"=w1340) -> ("error out"=w1337:errorcluster, "BigMAQ out"=w1339:refnum<class "BigMAQ.lvclass">)  [unwired: 7 in]
          }
          frame True {
          }
        }
        n476 = Bundle By Name(cluster=w1332, "big-maq"=w1322) -> (w1333:T23)
        n477 = Select(t="", s=w1317, f="AFM image and Inkscape file image do not  match. ::Using Inkscape file size::") -> (s? t:f=w1315:string)
        n478 = call <vilib>:"Add State(s) to Queue__jki_lib_state_machine.vi"("State(s) in (\"\")"=w1335) -> ("States Out"=w1334:string)  [unwired: 14 in]
      }
      frame "Big MAQ: Labels" {
        # "Parse: \n(Template Separater for Parsing. You can make a copy of, or modify, this frame)"
        n479 = Unbundle By Name(w1355) -> ("big-maq"=w1350:refnum<class "BigMAQ.lvclass">, "Litho"=w1345:T28)
        n480 = To Upper Case(1:w1351) -> (0:w1343:string)
        n481 = Match True/False String(2:"SHOW" ("false string"), 3:"HIDE" ("true string"), 4:w1343) -> (0:w1346:bool)  [unwired: 1 out]
        n482 = call "Label Visibility.vi"("Show Text"=w1346, "error in"=w1347, "Lithography Data"=w1345, "BigMAQ in"=w1350) -> ("error out"=w1348:errorcluster, "BigMAQ out"=w1349:refnum<class "BigMAQ.lvclass">)  [unwired: 6 in]
        n483 = Bundle By Name(cluster=w1355, "big-maq"=w1349) -> (w1356:T23)
        n484 = call <vilib>:"Add State(s) to Queue__jki_lib_state_machine.vi"("State(s) in (\"\")"=w1358) -> ("States Out"=w1357:string)  [unwired: 14 in]
      }
      frame "Big MAQ: Zoom Fit" {
        # "Parse: \n(Template Separater for Parsing. You can make a copy of, or modify, this frame)"
        n485 = Unbundle By Name(w1367) -> ("big-maq"=w1366:refnum<class "BigMAQ.lvclass">)
        n486 = call "Zoom to Fit.vi"("error in"=w1363, "BigMAQ in"=w1366) -> ("error out"=w1364:errorcluster, "ZoomSingle"=w1360:cluster{"X":sgl, "Y":sgl}, "BigMAQ out"=w1365:refnum<class "BigMAQ.lvclass">)  [unwired: 7 in]
        n487 = Build Array(w1360) -> (w1359:cluster{"X":sgl, "Y":sgl}[])
        n488 = Bundle By Name(cluster=w1367, "big-maq"=w1365, "Zoom History"=w1359) -> (w1368:T23)
        n489 = call <vilib>:"Add State(s) to Queue__jki_lib_state_machine.vi"("State(s) in (\"\")"=w1370) -> ("States Out"=w1369:string)  [unwired: 14 in]
      }
      frame "Big MAQ: Update" {
        # "Parse: \n(Template Separater for Parsing. You can make a copy of, or modify, this frame)"
        n490 = Unbundle By Name(w1377) -> ("big-maq"=w1376:refnum<class "BigMAQ.lvclass">)
        n491 = call "Update Control.vi"("error in"=w1373, "BigMAQ in"=w1376) -> ("error out"=w1374:errorcluster, "BigMAQ out"=w1375:refnum<class "BigMAQ.lvclass">)  [unwired: 8 in]
        n492 = Bundle By Name(cluster=w1377, "big-maq"=w1375) -> (w1378:T23)
        n493 = call <vilib>:"Add State(s) to Queue__jki_lib_state_machine.vi"("State(s) in (\"\")"=w1380) -> ("States Out"=w1379:string)  [unwired: 14 in]
      }
      frame "Big MAQ: Generate Overlay" {
        # "Parse: \n(Template Separater for Parsing. You can make a copy of, or modify, this frame)"
        n494 = Unbundle By Name(w1391) -> ("big-maq"=w1390:refnum<class "BigMAQ.lvclass">, "Litho"=w1381:T28, "UI.Hide Labels"=w1386:bool)
        n495 = Not(x=w1386) -> (.not. x?=w1385:bool)
        n496 = call "Generate New Overlay.vi"("Pixellate"=TRUE, "Label?"=w1385, "error in"=w1387, "Lithography Data"=w1381, "BigMAQ in"=w1390) -> ("error out"=w1388:errorcluster, "BigMAQ out"=w1389:refnum<class "BigMAQ.lvclass">)  [unwired: 5 in]
        n497 = Bundle By Name(cluster=w1391, "big-maq"=w1389) -> (w1392:T23)
        n498 = call <vilib>:"Add State(s) to Queue__jki_lib_state_machine.vi"("State(s) in (\"\")"=w1394) -> ("States Out"=w1393:string)  [unwired: 14 in]
      }
      frame "Big MAQ: Select Page" {
        # "Update the page control"
        # "Parse: \n(Template Separater for Parsing. You can make a copy of, or modify, this frame)"
        n499 = Unbundle By Name(w1407) -> ("big-maq"=w1406:refnum<class "BigMAQ.lvclass">, "UI.Page"=w1404:u32)
        n500 = call "Select Page.vi"("error in (no error)"=w1398, "Page"=w1404, "BigMAQ in"=w1406) -> ("error out"=w1399:errorcluster, "Corrected Page"=w1403:u32, "BigMAQ out"=w1405:refnum<class "BigMAQ.lvclass">)  [unwired: 6 in]
        n501 = Equal?(x=w1403, y=w1404) -> (x = y?=w1402:bool)
        n502 = Bundle By Name(cluster=w1407, "big-maq"=w1405) -> (w1408:T23)
        n503 = Select(t="", s=w1402, f="UI: Update Control >> Page") -> (s? t:f=w1401:string)
        n504 = call <vilib>:"Add State(s) to Queue__jki_lib_state_machine.vi"("State(s) in Front (\"\")"=w1401, "State(s) in (\"\")"=w1410) -> ("States Out"=w1409:string)  [unwired: 13 in]
      }
      frame "Big MAQ: Change Data Range" {
        # "Parse: \n(Template Separater for Parsing. You can make a copy of, or modify, this frame)"
        n505 = Unbundle By Name(w1422) -> ("big-maq"=w1421:refnum<class "BigMAQ.lvclass">, "UI.Image Data Range"=w1417:cluster{sgl, sgl})
        n506 = Unbundle(w1417) -> (w1416:sgl, w1415:sgl)
        n507 = Max & Min(x=w1416, y=w1415) -> (max(x,y)=w1414:sgl, min(x,y)=w1413:sgl)
        n508 = call "Change Data Range.vi"("error in"=w1418, "Minimum"=w1413, "Maximum"=w1414, "BigMAQ in"=w1421) -> ("error out"=w1419:errorcluster, "BigMAQ out"=w1420:refnum<class "BigMAQ.lvclass">)  [unwired: 6 in]
        n509 = Bundle By Name(cluster=w1422, "big-maq"=w1420) -> (w1423:T23)
        n510 = call <vilib>:"Add State(s) to Queue__jki_lib_state_machine.vi"("State(s) in (\"\")"=w1425) -> ("States Out"=w1424:string)  [unwired: 14 in]
      }
      frame "Big MAQ: Read Background" {
        # "Parse: \n(Template Separater for Parsing. You can make a copy of, or modify, this frame)"
        n511 = Unbundle By Name(w1435) -> ("big-maq"=w1434:refnum<class "BigMAQ.lvclass">, "UI.Background Image"=w1432:path)
        n512 = call "Read Background.vi"("error in (no error)"=w1430, "Path"=w1432, "BigMAQ in"=w1434) -> ("error out"=w1431:errorcluster, "BigMAQ out"=w1433:refnum<class "BigMAQ.lvclass">)  [unwired: 6 in, 1 out]
        n513 = Bundle By Name(cluster=w1435, "big-maq"=w1433, "UI.Page"=u32 0) -> (w1436:T23)
        n514 = call <vilib>:"Add State(s) to Queue__jki_lib_state_machine.vi"("State(s) in Front (\"\")"="UI: Update Control >> Page\nBig MAQ: Save Background", "State(s) in (\"\")"=w1438) -> ("States Out"=w1437:string)  [unwired: 13 in]
      }
      frame "Big MAQ: Save Background" {
        # "Parse: \n(Template Separater for Parsing. You can make a copy of, or modify, this frame)"
        n515 = Unbundle By Name(w1447) -> ("big-maq"=w1445:refnum<class "BigMAQ.lvclass">, "UI.Inkscape File (.svg)"=w1441:path)
        n516 = call "Get Background Image JPG Path.vi"("Inkscape Path"=w1441) -> ("Background JPG Path"=w1440:path)  [unwired: 2 in]
        n517 = call "Save Background.vi"("error in"=w1439, "File Path"=w1440, "BigMAQ in"=w1445) -> ("error out"=w1443:errorcluster, "BigMAQ out"=w1444:refnum<class "BigMAQ.lvclass">)  [unwired: 7 in]
        n518 = Bundle By Name(cluster=w1447, "big-maq"=w1444) -> (w1448:T23)
        n519 = call <vilib>:"Add State(s) to Queue__jki_lib_state_machine.vi"("State(s) in (\"\")"=w1450) -> ("States Out"=w1449:string)  [unwired: 14 in]
      }
      frame "Big MAQ: Save Render" {
        # "Parse: \n(Template Separater for Parsing. You can make a copy of, or modify, this frame)"
        n520 = Unbundle By Name(w1459) -> ("big-maq"=w1458:refnum<class "BigMAQ.lvclass">, "UI.Normal Save Path"=w1452:path)
        n521 = call "Save Image to Disk.vi"("Image Quality"=u32 1024, "error in"=w1455, "Path"=w1452, "BigMAQ in"=w1458) -> ("error out"=w1456:errorcluster, "BigMAQ out"=w1457:refnum<class "BigMAQ.lvclass">)  [unwired: 6 in]
        n522 = Bundle By Name(cluster=w1459, "big-maq"=w1457) -> (w1460:T23)
        n523 = call <vilib>:"Add State(s) to Queue__jki_lib_state_machine.vi"("State(s) in (\"\")"=w1462) -> ("States Out"=w1461:string)  [unwired: 14 in]
      }
      frame "Big MAQ: Autosave Render" {
        # "Need to change the path to align with the overwrite control"
        # "Parse: \n(Template Separater for Parsing. You can make a copy of, or modify, this frame)"
        n524 = Unbundle By Name(w1473) -> ("big-maq"=w1472:refnum<class "BigMAQ.lvclass">, "UI.Autosave Path"=w1467:path, "UI.Autosave?"=w1464:bool)
        n525 = case shown="True" w1464 {
          tunnel: w1472 -> [w1477 w1484]
          tunnel: [w1477 w1483] -> w1471
          tunnel: [w1478 w1482] -> w1470
          tunnel: w1469 -> [w1478 w1481]
          tunnel: w1467 -> [_ w1480]
          frame False {
          }
          frame True {
            n526 = call "Save Image to Disk.vi"("Image Quality"=u32 512, "error in"=w1481, "Path"=w1480, "BigMAQ in"=w1484) -> ("error out"=w1482:errorcluster, "BigMAQ out"=w1483:refnum<class "BigMAQ.lvclass">)  [unwired: 6 in]
          }
        }
        n527 = Bundle By Name(cluster=w1473, "big-maq"=w1471) -> (w1474:T23)
        n528 = Select(t="Render Autosaved to Disk", s=w1464, f="") -> (s? t:f=w1463:string)
        n529 = call <vilib>:"Add State(s) to Queue__jki_lib_state_machine.vi"("State(s) in (\"\")"=w1476) -> ("States Out"=w1475:string)  [unwired: 14 in]
      }
      frame "Big MAQ: Cleanup" {
        # "Parse: \n(Template Separater for Parsing. You can make a copy of, or modify, this frame)"
        n530 = Unbundle By Name(w1491) -> ("big-maq"=w1490:refnum<class "BigMAQ.lvclass">)
        n531 = call <vilib>:"Destroy.vi"("error in"=w1487, "BigMAQ in"=w1490) -> ("error out"=w1488:errorcluster, "BigMAQ out"=w1489:refnum<class "BigMAQ.lvclass">)  [unwired: 8 in]
        n532 = Bundle By Name(cluster=w1491, "big-maq"=w1489) -> (w1492:T23)
        n533 = call <vilib>:"Add State(s) to Queue__jki_lib_state_machine.vi"("State(s) in (\"\")"=w1494) -> ("States Out"=w1493:string)  [unwired: 14 in]
      }
      frame "Big MAQ: Initialize" {
        (unwired) i32[] [] items=["No Event"=0, "Click Event"=1, "Draw Event"=2, "Size Event"=4, "Scroll Event"=5, "Double Click Event"=8] ("Which Events")
        # "Parse: \n(Template Separater for Parsing. You can make a copy of, or modify, this frame)"
        n534 = control-ref of="Render"() -> (w1495:refnum<vi>)
        n535 = call <vilib>:"Create.vi"("error in (no error)"=w1499, "Resolution"=1024, "Reference"=w1495) -> ("error out"=w1500:errorcluster, "To Control"=→"Render":T1, "BigMAQ out"=w1497:refnum<class "BigMAQ.lvclass">)  [unwired: 6 in]
        n536 = Bundle By Name(cluster=w1503, "big-maq"=w1497) -> (w1504:T23)
        n537 = call <vilib>:"Add State(s) to Queue__jki_lib_state_machine.vi"("State(s) in (\"\")"=w1506) -> ("States Out"=w1505:string)  [unwired: 14 in]
      }
      frame "---------- Select ----------" {
        # "Select: \n(Template Separater for Selector i.e. MCLB. You can make a copy of, or modify, this frame)"
        n538 = Unbundle By Name(w1509) -> ("selector"=w1508:refnum<class "Selector.lvclass">)
        n539 = Bundle By Name(cluster=w1509, "selector"=w1508) -> (w1510:T23)
        n540 = call <vilib>:"Add State(s) to Queue__jki_lib_state_machine.vi"("State(s) in (\"\")"=w1513) -> ("States Out"=w1512:string)  [unwired: 14 in]
      }
      frame "Select: Change By Name" {
        # "Select: \n(Template Separater for Selector i.e. MCLB. You can make a copy of, or modify, this frame)"
        n541 = Unbundle By Name(w1515) -> ("GUIDs"=w1517:T30)
        n542 = case shown="\"first\"" w1514 {
          selector: w1514 -> [w1531 _]
          tunnel: [w1531 w1532] -> w1518
          tunnel: w1517 -> [_ w1540]
          frame Default {
          }
          frame "first" {
            n543 = Unbundle(w1540) -> ("Dots"=w1535:string[], "Funnels"=w1536:string[], "Rects"=w1537:string[], "Paths"=w1538:string[])
            n544 = Bundle(cluster=T11 {"paths"=[], "funnels"=[], "rects"=[], "dots"=[]} ("IDs"), "paths"=w1538, "funnels"=w1536, "rects"=w1537, "dots"=w1535) -> (w1534:T11)
            n545 = call "IDs to Names.vi"("IDs"=w1534) -> ("Names"=w1533:string[])  [unwired: 9 in, 1 out]
            n546 = Index Array(array=w1533) -> (element=w1532:string)  [unwired: 1 in]
          }
        }
        n547 = Unbundle By Name(w1515) -> ("selector"=w1523:refnum<class "Selector.lvclass">)
        n548 = call "Model--Set Value by Name.vi"("error in"=w1520, "Name"=w1518, "Selector in"=w1523) -> ("error out"=w1521:errorcluster, "element"=w1519:T39, "Selector out"=w1522:refnum<class "Selector.lvclass">)  [unwired: 6 in]
        n549 = Unbundle By Name(w1519) -> ("Name"=w1526:string)
        n550 = Bundle By Name(cluster=w1515, "selector"=w1522) -> (w1528:T23)
        n551 = call <vilib>:"Build State String with Arguments__JKI_lib_State_Machine.vi"("Arguments (\"\")"=w1526, "State"="Subpanel: Insert") -> ("State with Arguments"=w1524:string)  [unwired: 4 in]
        n552 = call <vilib>:"Add State(s) to Queue__jki_lib_state_machine.vi"("State(s) in Front (\"\")"=w1524, "State(s) in (\"\")"=w1530) -> ("States Out"=w1529:string)  [unwired: 13 in]
      }
      frame "Select: New Name Set" {
        # "Select: \n(Template Separater for Selector i.e. MCLB. You can make a copy of, or modify, this frame)"
        n553 = Unbundle By Name(w1555) -> ("selector"=w1553:refnum<class "Selector.lvclass">, "GUIDs"=w1543:T30)
        n554 = Unbundle By Name(w1543) -> ("Paths"=w1547:string[], "Funnels"=w1544:string[], "Rects"=w1545:string[], "Dots"=w1546:string[])
        n555 = Bundle By Name(cluster=T11 {"paths"=[], "funnels"=[], "rects"=[], "dots"=[]} ("IDs"), "paths"=w1547, "funnels"=w1544, "rects"=w1545, "dots"=w1546) -> (w1542:T11)
        n556 = call "IDs to Names.vi"("IDs"=w1542) -> ("Names"=w1551:string[])  [unwired: 9 in, 1 out]
        n557 = call-dynamic "Compare New Values.vi"("error in (no error)"=w1549, "New Values"=w1551, "Selector in"=w1553) -> ("error out"=w1550:errorcluster, "Selector out"=w1552:refnum<class "Selector.lvclass">)  [unwired: 6 in, 1 out]
        n558 = Bundle By Name(cluster=w1555, "selector"=w1552) -> (w1556:T23)
        n559 = call <vilib>:"Add State(s) to Queue__jki_lib_state_machine.vi"("State(s) in (\"\")"=w1558) -> ("States Out"=w1557:string)  [unwired: 14 in]
      }
      frame "Select: Update" {
        # "Select: \n(Template Separater for Selector i.e. MCLB. You can make a copy of, or modify, this frame)"
        n560 = Unbundle By Name(w1565) -> ("selector"=w1563:refnum<class "Selector.lvclass">)
        n561 = call "UI--Update.vi"("error in"=w1560, "Selector in"=w1563) -> ("error out"=w1561:errorcluster, "Selector out"=w1562:refnum<class "Selector.lvclass">)  [unwired: 8 in]
        n562 = Bundle By Name(cluster=w1565, "selector"=w1562) -> (w1566:T23)
        n563 = call <vilib>:"Add State(s) to Queue__jki_lib_state_machine.vi"("State(s) in (\"\")"=w1568) -> ("States Out"=w1567:string)  [unwired: 14 in]
      }
      frame "Select: Apply Symbols" {
        # "Select: \n(Template Separater for Selector i.e. MCLB. You can make a copy of, or modify, this frame)"
        n564 = Unbundle By Name(w1575) -> ("selector"=w1573:refnum<class "Selector.lvclass">)
        n565 = call "UI--Apply Item Symbols.vi"("error in"=w1570, "Selector in"=w1573) -> ("error out"=w1571:errorcluster, "Selector out"=w1572:refnum<class "Selector.lvclass">)  [unwired: 8 in]
        n566 = Bundle By Name(cluster=w1575, "selector"=w1572) -> (w1576:T23)
        n567 = call <vilib>:"Add State(s) to Queue__jki_lib_state_machine.vi"("State(s) in (\"\")"=w1578) -> ("States Out"=w1577:string)  [unwired: 14 in]
      }
      frame "Select: Change Value" {
        # "Select: \n(Template Separater for Selector i.e. MCLB. You can make a copy of, or modify, this frame)"
        n568 = Unbundle By Name(w1592) -> ("selector"=w1591:refnum<class "Selector.lvclass">)
        n569 = Decimal String To Number(string=w1587, default (0L)=0 ("default (0 I32)")) -> (number=w1588:i32)  [unwired: 1 in, 1 out]
        n570 = call "Model--Set Value.vi"("error in"=w1585, "Value"=w1588, "Selector in"=w1591) -> ("error out"=w1586:errorcluster, "element"=w1582:T39, "Selector out"=w1590:refnum<class "Selector.lvclass">)  [unwired: 6 in]
        n571 = Unbundle By Name(w1582) -> ("Name"=w1580:string)
        n572 = Bundle By Name(cluster=w1592, "selector"=w1590) -> (w1593:T23)
        n573 = call <vilib>:"Build State String with Arguments__JKI_lib_State_Machine.vi"("Arguments (\"\")"=w1580, "State"="Subpanel: Insert") -> ("State with Arguments"=w1579:string)  [unwired: 4 in]
        n574 = call <vilib>:"Add State(s) to Queue__jki_lib_state_machine.vi"("State(s) in Front (\"\")"=w1579, "State(s) in (\"\")"=w1595) -> ("States Out"=w1594:string)  [unwired: 13 in]
      }
      frame "Select: Reorder" {
        # "Select: \n(Template Separater for Selector i.e. MCLB. You can make a copy of, or modify, this frame)"
        n575 = Unbundle By Name(w1602) -> ("selector"=w1601:refnum<class "Selector.lvclass">)
        n576 = call "Model--Reorder.vi"("error in"=w1599, "Selector in"=w1601) -> ("error out"=w1598:errorcluster, "Selector out"=w1600:refnum<class "Selector.lvclass">)  [unwired: 8 in]
        n577 = Bundle By Name(cluster=w1602, "selector"=w1600) -> (w1603:T23)
        n578 = call <vilib>:"Add State(s) to Queue__jki_lib_state_machine.vi"("State(s) in (\"\")"=w1605) -> ("States Out"=w1604:string)  [unwired: 14 in]
      }
      frame "Select: Order Litho" {
        # "Select: \n(Template Separater for Selector i.e. MCLB. You can make a copy of, or modify, this frame)"
        n579 = Unbundle By Name(w1618) -> ("selector"=w1617:refnum<class "Selector.lvclass">, "Litho"=w1608:T28)
        n580 = for {
          tunnel: w1608 -> [w1626] mode=indexing
          tunnel: [w1624] -> w1609 mode=indexing
          n581 = Unbundle By Name(w1626) -> ("Name"=w1625:string)
          n582 = Bundle By Name(cluster=cluster{"Name":string, "Value":variant} {"Name"="p0", "Value"=variant(cluster{"Name":string, "Litho":cluster{"X":dbl, "Y":dbl, "Speed":dbl, "Voltage":dbl}[], "Set Resistance":enum16{"open", "discharge tip", "0 ohms", "100k ohm", "10M ohm", "1G ohm"}, "Meta":variant} {"Name"="p0", "Litho"=array[5841 elements], "Set Resistance"=enum."1G ohm", "Meta"=variant})} ("KVP"), "Name"=w1625, "Value"=w1626) -> (w1624:cluster{"Name":string, "Value":variant})
        }
        n583 = call "Model--Order Key Values.vi"("error in"=w1612, "KVP In"=w1609, "Selector in"=w1617) -> ("error out"=w1614:errorcluster, "KVP Out"=w1611:cluster{"Name":string, "Value":variant}[], "Selector out"=w1616:refnum<class "Selector.lvclass">)  [unwired: 6 in]
        n584 = for {
          tunnel: w1611 -> [w1623] mode=indexing
          tunnel: [w1622] -> w1610 mode=indexing
          n585 = Unbundle By Name(w1623) -> ("Value"=w1622:variant)
        }
        n586 = Variant To Data(error in=w1614, type=w1608, Variant=w1610) -> (data=w1615:T28, error out=w1613:errorcluster)
        n587 = Bundle By Name(cluster=w1618, "selector"=w1616, "Litho"=w1615) -> (w1619:T23)
        n588 = call <vilib>:"Add State(s) to Queue__jki_lib_state_machine.vi"("State(s) in (\"\")"=w1621) -> ("States Out"=w1620:string)  [unwired: 14 in]
      }
      frame "Select: Group" {
        # "Select: \n(Template Separater for Selector i.e. MCLB. You can make a copy of, or modify, this frame)"
        n589 = Unbundle By Name(w1644) -> ("selector"=w1643:refnum<class "Selector.lvclass">)
        n590 = case shown="\"add\"" w1639 {
          selector: w1639 -> [w1648 w1653 w1660 w1667]
          tunnel: w1643 -> [w1652 w1658 w1665 w1673]
          tunnel: [w1652 w1659 w1666 w1672] -> w1642
          tunnel: [w1651 w1657 w1664 w1671] -> w1641
          tunnel: w1640 -> [w1651 w1656 w1663 w1670]
          tunnel: ["" w1655 w1662 w1669] -> w1636
          tunnel: ["" "" w1661 w1668] -> w1634
          tunnel: [w1648 w1653 w1660 w1667] -> w1635
          frame Default {
          }
          frame "remove" {
            n591 = call "Model--Remove from Group.vi"("error in"=w1656, "Selector in"=w1658) -> ("error out"=w1657:errorcluster, "Name"=w1655:string, "Selector out"=w1659:refnum<class "Selector.lvclass">)  [unwired: 7 in]
          }
          frame "create" {
            n592 = call "Model--Create New Group.vi"("error in"=w1663, "Selector in"=w1665) -> ("error out"=w1664:errorcluster, "Group"=w1661:string, "Name"=w1662:string, "Selector out"=w1666:refnum<class "Selector.lvclass">)  [unwired: 6 in]
          }
          frame "add" {
            n593 = call "Model--Add to Group.vi"("error in"=w1670, "Selector in"=w1673) -> ("error out"=w1671:errorcluster, "Group"=w1668:string, "Name"=w1669:string, "Selector out"=w1672:refnum<class "Selector.lvclass">)  [unwired: 6 in]
          }
        }
        n594 = Build Array(w1635, w1636, w1634) -> (w1632:string[])
        n595 = Array To Spreadsheet String(delimiter (Tab)=":", array=w1632, 3:"%s" ("format string")) -> (spreadsheet string=w1631:string)
        n596 = call <vilib>:"Build State String with Arguments__JKI_lib_State_Machine.vi"("Arguments (\"\")"=w1631, "State"="Settings: Group") -> ("State with Arguments"=w1629:string)  [unwired: 4 in]
        n597 = Bundle By Name(cluster=w1644, "selector"=w1642) -> (w1645:T23)
        n598 = call <vilib>:"Add State(s) to Queue__jki_lib_state_machine.vi"("State(s) in Front (\"\")"=w1629, "State(s) in (\"\")"=w1647) -> ("States Out"=w1646:string)  [unwired: 13 in]
      }
      frame "Select: Create" {
        # "Select: \n(Template Separater for Selector i.e. MCLB. You can make a copy of, or modify, this frame)"
        n599 = control-ref of="MCLB"() -> (w1676:refnum<vi>)
        n600 = call <vilib>:"Create.vi"("error in"=w1677, "Reference"=w1676) -> ("error out"=w1678:errorcluster, "Selector out"=w1679:refnum<class "Selector.lvclass">)  [unwired: 8 in]
        n601 = Bundle By Name(cluster=w1680, "selector"=w1679) -> (w1681:T23)
        n602 = call <vilib>:"Add State(s) to Queue__jki_lib_state_machine.vi"("State(s) in (\"\")"=w1683) -> ("States Out"=w1682:string)  [unwired: 14 in]
      }
      frame "---------- Subpanel ----------" {
        # "Subpanel: \n(Template Separater for Subpanel Editor. You can make a copy of, or modify, this frame)"
        n603 = Unbundle By Name(w1686) -> ("sbpnl.edit"=w1685:refnum<class "Subpanel.Edit.lvclass">)
        n604 = Bundle By Name(cluster=w1686, "sbpnl.edit"=w1685) -> (w1687:T23)
        n605 = call <vilib>:"Add State(s) to Queue__jki_lib_state_machine.vi"("State(s) in (\"\")"=w1690) -> ("States Out"=w1689:string)  [unwired: 14 in]
      }
      frame "Subpanel: Insert" {
        # "Subpanel: \n(Template Separater for Subpanel Editor. You can make a copy of, or modify, this frame)"
        n606 = Unbundle By Name(w1699) -> ("sbpnl.edit"=w1698:refnum<class "Subpanel.Edit.lvclass">)
        n607 = call "Name To Type.vi"("Name"=w1693) -> ("Type"=w1694:string)  [unwired: 4 in]
        n608 = call "Insert Into Subpanel.vi"("error in (no error)"=w1695, "Key"=w1694, "Subpanel.lvclass"=w1698) -> ("error out"=w1696:errorcluster, "Subpanel out"=w1697:refnum<class "Subpanel.Edit.lvclass">)  [unwired: 7 in]
        n609 = Bundle By Name(cluster=w1699, "sbpnl.edit"=w1697) -> (w1700:T23)
        n610 = call <vilib>:"Add State(s) to Queue__jki_lib_state_machine.vi"("State(s) in (\"\")"=w1702) -> ("States Out"=w1701:string)  [unwired: 14 in]
      }
      frame "Subpanel: Close" {
        # "Subpanel: \n(Template Separater for Subpanel Editor. You can make a copy of, or modify, this frame)"
        n611 = Unbundle By Name(w1709) -> ("sbpnl.edit"=w1708:refnum<class "Subpanel.Edit.lvclass">)
        n612 = call "Close.vi"("error in (no error)"=w1705, "Subpanel.lvclass"=w1708) -> ("error out"=w1706:errorcluster, "Subpanel out"=w1707:refnum<class "Subpanel.Edit.lvclass">)  [unwired: 8 in]
        n613 = Bundle By Name(cluster=w1709, "sbpnl.edit"=w1707) -> (w1710:T23)
        n614 = call <vilib>:"Add State(s) to Queue__jki_lib_state_machine.vi"("State(s) in (\"\")"=w1712) -> ("States Out"=w1711:string)  [unwired: 14 in]
      }
      frame "Subpanel: Initialize" {
        # "Subpanel: \n(Template Separater for Subpanel Editor. You can make a copy of, or modify, this frame)"
        n615 = control-ref of="Properties"() -> (w1715:refnum<vi>)
        n616 = call "Get Manager.vi"("error in (no error)"=w1717) -> ("error out"=w1720:errorcluster, "Subpanel.Edit"=w1719:refnum<class "Subpanel.Edit.lvclass">)  [unwired: 9 in]
        n617 = call "Initialize.vi"("error in (no error)"=w1720, "Subpanel.lvclass"=w1719, "Sub Panel"=w1715) -> ("error out"=w1716:errorcluster, "Subpanel out"=w1718:refnum<class "Subpanel.Edit.lvclass">)  [unwired: 7 in]
        n618 = Bundle By Name(cluster=w1721, "sbpnl.edit"=w1718) -> (w1722:T23)
        n619 = call <vilib>:"Add State(s) to Queue__jki_lib_state_machine.vi"("State(s) in (\"\")"=w1724) -> ("States Out"=w1723:string)  [unwired: 14 in]
      }
      frame "---------- Log ----------" {
        # "Parse: \n(Template Separater for Parsing. You can make a copy of, or modify, this frame)"
        n620 = Unbundle By Name(w1727) -> ("log"=w1726:refnum<class "Log.Litho.lvclass">)
        n621 = Bundle By Name(cluster=w1727, "log"=w1726) -> (w1728:T23)
        n622 = call <vilib>:"Add State(s) to Queue__jki_lib_state_machine.vi"("State(s) in (\"\")"=w1731) -> ("States Out"=w1730:string)  [unwired: 14 in]
      }
      frame "Log: Start" {
        # "Tool: \n(Template Separater for Tooling. You can make a copy of, or modify, this frame)"
        n623 = Unbundle By Name(w1741) -> ("log"=w1737:refnum<class "Log.Litho.lvclass">)
        n624 = call <vilib>:"Create.vi"("error in (no error)"=w1734, "SMO"=w1737) -> ("error out"=w1738:errorcluster, "SMO out"=w1739:refnum<class "Log.Litho.lvclass">)  [unwired: 7 in, 1 out]
        n625 = call <vilib>:"Start.vi"("ms timeout (if waiting)"=10000, "error in (no error)"=w1738, "SMO"=w1739) -> ("error out"=w1735:errorcluster, "SMO out"=w1736:refnum<class "Log.Litho.lvclass">)  [unwired: 7 in]
        n626 = Bundle By Name(cluster=w1741, "log"=w1736) -> (w1742:T23)
        n627 = call <vilib>:"Add State(s) to Queue__jki_lib_state_machine.vi"("State(s) in (\"\")"=w1744) -> ("States Out"=w1743:string)  [unwired: 14 in]
      }
      frame "Log: Stop" {
        # "Tool: \n(Template Separater for Tooling. You can make a copy of, or modify, this frame)"
        n628 = Unbundle By Name(w1754) -> ("log"=w1750:refnum<class "Log.Litho.lvclass">)
        n629 = call <vilib>:"Stop.vi"("timeout in ms (-1)"=10000, "error in (no error)"=w1748, "SMO"=w1750) -> ("error out"=w1752:errorcluster, "SMO out"=w1751:refnum<class "Log.Litho.lvclass">)  [unwired: 7 in]
        n630 = call <vilib>:"Destroy.vi"("error in (no error)"=w1752, "SMO"=w1751) -> ("error out"=w1749:errorcluster)  [unwired: 9 in]
        n631 = Bundle By Name(cluster=w1754, "log"=refnum<class "Log.Litho.lvclass"> refnum) -> (w1755:T23)
        n632 = call <vilib>:"Add State(s) to Queue__jki_lib_state_machine.vi"("State(s) in (\"\")"=w1757) -> ("States Out"=w1756:string)  [unwired: 14 in]
      }
      frame "---------- Config ----------" {
        # "Parse: \n(Template Separater for Parsing. You can make a copy of, or modify, this frame)"
        n633 = Unbundle By Name(w1760) -> ("config"=w1759:refnum<class "Configuration.lvclass">)
        n634 = Bundle By Name(cluster=w1760, "config"=w1759) -> (w1761:T23)
        n635 = call <vilib>:"Add State(s) to Queue__jki_lib_state_machine.vi"("State(s) in (\"\")"=w1764) -> ("States Out"=w1763:string)  [unwired: 14 in]
      }
      frame "Config: Initialize" {
        # "Parse: \n(Template Separater for Parsing. You can make a copy of, or modify, this frame)"
        n636 = Unbundle By Name(w1773) -> ("config"=w1769:refnum<class "Configuration.lvclass">)
        n637 = call "Base INI Folder Path.vi"() -> ("Base Path"=w1770:path)  [unwired: 11 in]
        n638 = call <userlib>:"Write Path.vi"("error in (no error)"=w1766, "Filename [Configuration.ini]"="Config.ini" ("File (Configuration.ini)"), "Path"=w1770, "Configuration in"=w1769) -> ("error out"=w1767:errorcluster, "Configuration out"=w1768:refnum<class "Configuration.lvclass">)  [unwired: 6 in]
        n639 = Bundle By Name(cluster=w1773, "config"=w1768) -> (w1774:T23)
        n640 = call <vilib>:"Add State(s) to Queue__jki_lib_state_machine.vi"("State(s) in (\"\")"=w1776) -> ("States Out"=w1775:string)  [unwired: 14 in]
      }
      frame "Config: Write" {
        # "Parse: \n(Template Separater for Parsing. You can make a copy of, or modify, this frame)"
        n641 = Unbundle By Name(w1788) -> ("config"=w1790:refnum<class "Configuration.lvclass">, "UI.Inkscape File (.svg)"=w1782:path, "UI.Background Image"=w1783:path, "UI.Autosave Path"=w1784:path, "UI.Autosave?"=w1781:bool, "UI.Hide Labels"=w1778:bool, "UI.Normal Save Path"=w1777:path)
        n642 = Bundle By Name(cluster=T21 {"Inkscape Path"=path "", "Background Path"=path "", "Autosave Render Path"=path "", "Autosave Render"=FALSE, "Hide Labels"=FALSE, "Normal Render Path"=path ""} ("Configuration Data"), "Inkscape Path"=w1782, "Background Path"=w1783, "Autosave Render Path"=w1784, "Autosave Render"=w1781, "Hide Labels"=w1778, "Normal Render Path"=w1777) -> (w1780:T21)
        n643 = call <userlib>:"Write Configuration.vi"("error in (no error)"=w1786, "Variant"=w1780, "Configuration in"=w1790) -> ("error out"=w1787:errorcluster, "Configuration out"=w1789:refnum<class "Configuration.lvclass">)  [unwired: 7 in]
        n644 = Bundle By Name(cluster=w1788, "config"=w1789) -> (w1792:T23)
        n645 = call <vilib>:"Add State(s) to Queue__jki_lib_state_machine.vi"("State(s) in (\"\")"=w1794) -> ("States Out"=w1793:string)  [unwired: 14 in]
      }
      frame "Config: Read" {
        w1798 = T21 {"Inkscape Path"=path "", "Background Path"=path "", "Autosave Render Path"=path "", "Autosave Render"=FALSE, "Hide Labels"=FALSE, "Normal Render Path"=path ""} ("Configuration Data")
        # "Parse: \n(Template Separater for Parsing. You can make a copy of, or modify, this frame)"
        n646 = Unbundle By Name(w1811) -> ("config"=w1807:refnum<class "Configuration.lvclass">)
        n647 = call <userlib>:"Read Configuration.vi"("INI Fomatted Cluster Type"=w1798, "error in (no error)"=w1804, "Configuration in"=w1807) -> ("error out"=w1808:errorcluster, "Configuration"=w1809:variant, "Configuration out"=w1806:refnum<class "Configuration.lvclass">)  [unwired: 6 in]
        n648 = Variant To Data(error in=w1808, type=w1798, Variant=w1809) -> (data=w1803:T21, error out=w1805:errorcluster)
        n649 = Unbundle By Name(w1803) -> ("Inkscape Path"=w1802:path, "Background Path"=w1801:path, "Autosave Render Path"=w1800:path, "Autosave Render"=w1799:bool, "Hide Labels"=w1796:bool, "Normal Render Path"=w1795:path)
        n650 = Bundle By Name(cluster=w1811, "config"=w1806, "UI.Inkscape File (.svg)"=w1802, "UI.Background Image"=w1801, "UI.Autosave Path"=w1800, "UI.Autosave?"=w1799, "UI.Hide Labels"=w1796, "UI.Normal Save Path"=w1795) -> (w1812:T23)
        n651 = call <vilib>:"Add State(s) to Queue__jki_lib_state_machine.vi"("State(s) in (\"\")"=w1814) -> ("States Out"=w1813:string)  [unwired: 14 in]
      }
      frame "---------- AFM ----------" {
        # "Parse: \n(Template Separater for Parsing. You can make a copy of, or modify, this frame)"
        n652 = Unbundle By Name(w1817) -> ("afm_mngr"=w1816:refnum<class "AFM_Driver_Manager.lvclass">)
        n653 = Bundle By Name(cluster=w1817, "afm_mngr"=w1816) -> (w1818:T23)
        n654 = call <vilib>:"Add State(s) to Queue__jki_lib_state_machine.vi"("State(s) in (\"\")"=w1821) -> ("States Out"=w1820:string)  [unwired: 14 in]
      }
      frame "AFM: Lithography Finished" {
        # "Parse: \n(Template Separater for Parsing. You can make a copy of, or modify, this frame)"
        n655 = Unbundle By Name(w1828) -> ("afm_mngr"=w1826:refnum<class "AFM_Driver_Manager.lvclass">)
        n656 = call "AFM_Driver_Manager.OnLithographyFinish.vi"("error in (no error)"=w1823, "AFM_Driver_Manager in"=w1826) -> ("error out"=w1824:errorcluster, "AFM_Driver_Manager out"=w1825:refnum<class "AFM_Driver_Manager.lvclass">)  [unwired: 8 in]
        n657 = Bundle By Name(cluster=w1828, "afm_mngr"=w1825) -> (w1829:T23)
        n658 = call <vilib>:"Add State(s) to Queue__jki_lib_state_machine.vi"("State(s) in (\"\")"=w1831) -> ("States Out"=w1830:string)  [unwired: 14 in]
      }
      frame "AFM: Stop Manager" {
        # "Parse: \n(Template Separater for Parsing. You can make a copy of, or modify, this frame)"
        n659 = Unbundle By Name(w1838) -> ("afm_mngr"=w1836:refnum<class "AFM_Driver_Manager.lvclass">)
        n660 = call "AFM_Driver_Manager.Shutdown.vi"("error in (no error)"=w1834, "AFM_Driver_Manager in"=w1836) -> ("error out"=w1835:errorcluster)  [unwired: 9 in]
        n661 = Bundle By Name(cluster=w1838, "afm_mngr"=refnum<class "AFM_Driver_Manager.lvclass"> refnum) -> (w1839:T23)
        n662 = call <vilib>:"Add State(s) to Queue__jki_lib_state_machine.vi"("State(s) in (\"\")"=w1841) -> ("States Out"=w1840:string)  [unwired: 14 in]
      }
      frame "AFM: Background Image" {
        # "Parse: \n(Template Separater for Parsing. You can make a copy of, or modify, this frame)"
        n663 = Unbundle By Name(w1849) -> ("afm_mngr"=w1847:refnum<class "AFM_Driver_Manager.lvclass">, "UI.Background Image"=w1843:path)
        n664 = call "AFM_Driver_Manager.SendBackgroundImage.vi"("error in (no error)"=w1844, "Path"=w1843, "AFM_Driver_Manager in"=w1847) -> ("error out"=w1845:errorcluster, "AFM_Driver_Manager out"=w1846:refnum<class "AFM_Driver_Manager.lvclass">)  [unwired: 7 in]
        n665 = Bundle By Name(cluster=w1849, "afm_mngr"=w1846) -> (w1850:T23)
        n666 = call <vilib>:"Add State(s) to Queue__jki_lib_state_machine.vi"("State(s) in (\"\")"=w1852) -> ("States Out"=w1851:string)  [unwired: 14 in]
      }
      frame "AFM: Lithography Data" {
        # "Parse: \n(Template Separater for Parsing. You can make a copy of, or modify, this frame)"
        n667 = Unbundle By Name(w1875) -> ("afm_mngr"=w1873:refnum<class "AFM_Driver_Manager.lvclass">, "Litho"=w1853:T28)
        n668 = for {
          tunnel: [w1880] -> w1868
          tunnel: w1853 -> [w1881] mode=indexing
          stop <- w1879 continue-if-true
          n669 = Unbundle By Name(w1881) -> ("Litho"=w1880:T40)
          n670 = Empty Array?(array=w1880) -> (empty?=w1879:bool)
        }
        n671 = for {
          tunnel: w1868 -> [w1884] mode=indexing
          tunnel: [w1883] -> w1865 mode=indexing
          tunnel: [w1882] -> w1862 mode=indexing
          n672 = Unbundle(w1884) -> ("X"=w1883:dbl, "Y"=w1882:dbl)  [unwired: 2 out]
        }
        n673 = call "AFM_Driver_Manager.SendLithography.vi"("error in (no error)"=w1870, "Lithography Data"=w1853, "AFM_Driver_Manager in"=w1873) -> ("error out"=w1871:errorcluster, "AFM_Driver_Manager out"=w1872:refnum<class "AFM_Driver_Manager.lvclass">)  [unwired: 7 in]
        n674 = Bundle By Name(cluster=w1875, "afm_mngr"=w1872) -> (w1876:T23)
        n675 = Rotate 1D Array(1:w1865, 2:1 ("n")) -> (0:w1866:dbl[])
        n676 = Rotate 1D Array(1:w1862, 2:1 ("n")) -> (0:w1864:dbl[])
        n677 = Subtract(x=w1866, y=w1865) -> (x-y=w1861:dbl[])
        n678 = Subtract(x=w1864, y=w1862) -> (x-y=w1860:dbl[])
        n679 = Square(x=w1861) -> (x^2=w1859:dbl[])
        n680 = Square(x=w1860) -> (x^2=w1858:dbl[])
        n681 = Add(x=w1859, y=w1858) -> (x+y=w1857:dbl[])
        n682 = Square Root(x=w1857) -> (sqrt(x)=w1856:dbl[])
        n683 = Delete From Array(array=w1856, length=2, index=0) -> ()  [unwired: 2 out]
        n684 = call <vilib>:"Add State(s) to Queue__jki_lib_state_machine.vi"("State(s) in (\"\")"=w1878) -> ("States Out"=w1877:string)  [unwired: 14 in]
      }
      frame "AFM: Run Lithography" {
        # "Parse: \n(Template Separater for Parsing. You can make a copy of, or modify, this frame)"
        n685 = Unbundle By Name(w1891) -> ("afm_mngr"=w1889:refnum<class "AFM_Driver_Manager.lvclass">)
        n686 = call "AFM_Driver_Manager.SendRun.vi"("error in (no error)"=w1886, "AFM_Driver_Manager in"=w1889) -> ("error out"=w1887:errorcluster, "AFM_Driver_Manager out"=w1888:refnum<class "AFM_Driver_Manager.lvclass">)  [unwired: 8 in]
        n687 = Bundle By Name(cluster=w1891, "afm_mngr"=w1888) -> (w1892:T23)
        n688 = call <vilib>:"Add State(s) to Queue__jki_lib_state_machine.vi"("State(s) in (\"\")"=w1894) -> ("States Out"=w1893:string)  [unwired: 14 in]
      }
      frame "AFM: Insert Into Subpanel" {
        # "Parse: \n(Template Separater for Parsing. You can make a copy of, or modify, this frame)"
        n689 = Unbundle By Name(w1902) -> ("afm_mngr"=w1900:refnum<class "AFM_Driver_Manager.lvclass">)
        n690 = control-ref of="AFM Settings"() -> (w1896:refnum<vi>)
        n691 = call "AFM_Driver_Manager.InsertActiveIntoSubpanel.vi"("error in (no error)"=w1897, "SubPnl Refnum"=w1896, "AFM_Driver_Manager in"=w1900) -> ("error out"=w1898:errorcluster, "AFM_Driver_Manager out"=w1899:refnum<class "AFM_Driver_Manager.lvclass">)  [unwired: 7 in]
        n692 = Bundle By Name(cluster=w1902, "afm_mngr"=w1899) -> (w1903:T23)
        n693 = call <vilib>:"Add State(s) to Queue__jki_lib_state_machine.vi"("State(s) in (\"\")"=w1905) -> ("States Out"=w1904:string)  [unwired: 14 in]
      }
      frame "AFM: Set Active" {
        # "Parse: \n(Template Separater for Parsing. You can make a copy of, or modify, this frame)"
        n694 = Unbundle By Name(w1914) -> ("afm_mngr"=w1912:refnum<class "AFM_Driver_Manager.lvclass">)
        n695 = Decimal String To Number(string=w1908) -> (number=w1907:i32)  [unwired: 2 in, 1 out]
        n696 = call "AFM_Driver_Manager.SetActive.vi"("error in (no error)"=w1909, "Active Index"=w1907, "AFM_Driver_Manager in"=w1912) -> ("error out"=w1910:errorcluster, "AFM_Driver_Manager out"=w1911:refnum<class "AFM_Driver_Manager.lvclass">)  [unwired: 7 in]
        n697 = Bundle By Name(cluster=w1914, "afm_mngr"=w1911) -> (w1915:T23)
        n698 = call <vilib>:"Add State(s) to Queue__jki_lib_state_machine.vi"("State(s) in (\"\")"=w1917) -> ("States Out"=w1916:string)  [unwired: 14 in]
      }
      frame "AFM: Initialize Driver" {
        # "Parse: \n(Template Separater for Parsing. You can make a copy of, or modify, this frame)"
        n699 = Unbundle By Name(w1928) -> ("afm_mngr"=w1926:refnum<class "AFM_Driver_Manager.lvclass">, "root path"=w1919:path)
        n700 = Build Path(base path=w1919, name or relative path="AFMs\\Asylum_Driver\\Asylum_Driver.vi") -> (appended path=w1924:path)
        n701 = Build Array(w1924) -> (w1922:path[])
        n702 = call "AFM_Driver_Manager.InitializeDrivers.vi"("error in (no error)"=w1920, "Paths"=w1922, "AFM_Driver_Manager in"=w1926) -> ("error out"=w1921:errorcluster, "AFM_Driver_Manager out"=w1925:refnum<class "AFM_Driver_Manager.lvclass">)  [unwired: 7 in]
        n703 = Bundle By Name(cluster=w1928, "afm_mngr"=w1925) -> (w1929:T23)
        n704 = call <vilib>:"Add State(s) to Queue__jki_lib_state_machine.vi"("State(s) in (\"\")"=w1931) -> ("States Out"=w1930:string)  [unwired: 14 in]
      }
      frame "AFM: Initialize Manager" {
        # "Parse: \n(Template Separater for Parsing. You can make a copy of, or modify, this frame)"
        n705 = Unbundle By Name(w1938) -> ("afm_mngr"=w1936:refnum<class "AFM_Driver_Manager.lvclass">)
        n706 = call "AFM_Driver_Manager.Initialize.vi"("error in (no error)"=w1933, "AFM_Driver_Manager in"=w1936) -> ("error out"=w1934:errorcluster, "AFM_Driver_Manager out"=w1935:refnum<class "AFM_Driver_Manager.lvclass">)  [unwired: 8 in]
        n707 = Bundle By Name(cluster=w1938, "afm_mngr"=w1935) -> (w1939:T23)
        n708 = call <vilib>:"Add State(s) to Queue__jki_lib_state_machine.vi"("State(s) in (\"\")"=w1941) -> ("States Out"=w1940:string)  [unwired: 14 in]
      }
    }
    n709 = call "Write Status.vi"("Status"=w5, "States In"=w6) -> ("States Out"=w4:string)  [unwired: 9 in]
  }
